vi "grading table searching.vi"() -> ()   [LabVIEW 2019, in "database.lvlib"]
uses:
  database.lvlib
panel:
  in  "OK":bool
  out "Query String":string
  out "String 4":string="Parameter"
  out "String 3":string="Operation"
  out "String 2":string="Value 2"
  out "String 1":string="Value 1"
  out "Value String 12":string="Value"
  out "Value String 11":string="Value"
  out "Value String 10":string="Value"
  out "Value String 9":string="Value"
  out "Value String 8":string="Value"
  out "Value String 7":string="Value"
  out "Value String 6":string="Value"
  out "Value String 5":string="Value"
  out "Value String 4":string="Value"
  out "Value String 3":string="Value"
  out "Value String 2":string="Value"
  out "Value String 1":string="Value"
  in  "Operator 17":u16(ring) items=["AND", "OR"]
  in  "Operator 16":u16(ring) items=["AND", "OR"]
  in  "Operator 15":u16(ring) items=["AND", "OR"]
  in  "Operator 14":u16(ring) items=["AND", "OR"]
  in  "Operator 13":u16(ring) items=["AND", "OR"]
  in  "sub 5":bool=TRUE
  in  "sub 4":bool=TRUE
  in  "sub 3":bool=TRUE
  in  "sub 2":bool=TRUE
  in  "sub 1":bool=TRUE
  in  "add 5":bool=TRUE
  in  "add 4":bool=TRUE
  in  "add 3":bool=TRUE
  in  "add 2":bool=TRUE
  in  "Operator 11":u16(ring) items=["All", "P=V1", "P#V1", "P<V1", "P<=V1", "P>V1", "P>=V1", "V1<P<V2", "V1<=P<V2", "V1<P<=V2", "V1<=P<=V2"]
  in  "Operator 9":u16(ring) items=["All", "P=V1", "P#V1", "P<V1", "P<=V1", "P>V1", "P>=V1", "V1<P<V2", "V1<=P<V2", "V1<P<=V2", "V1<=P<=V2"]
  in  "Operator 7":u16(ring) items=["All", "P=V1", "P#V1", "P<V1", "P<=V1", "P>V1", "P>=V1", "V1<P<V2", "V1<=P<V2", "V1<P<=V2", "V1<=P<=V2"]
  in  "Projector Situation 12":u16(ring) items=["OFF", "ON"]
  in  "Projector Situation 11":u16(ring) items=["OFF", "ON"]
  in  "Camera Situation 12":u16(ring) items=["OFF", "ON"]
  in  "Camera Situation 11":u16(ring) items=["OFF", "ON"]
  in  "Control Mode 12":u16(ring) items=["Manual", "Auto"]
  in  "Control Mode 11":u16(ring) items=["Manual", "Auto"]
  in  "Disc Situation 12":u16(ring) items=["Stop", "Run"]
  in  "Disc Situation 11":u16(ring) items=["Stop", "Run"]
  in  "Time 12":timestamp format="%<%H:%M:%S>T"
  in  "Time 11":timestamp format="%<%H:%M:%S>T"
  in  "Date 12":timestamp format="%<%Y/%m/%d>T"
  in  "Date 11":timestamp format="%<%Y/%m/%d>T"
  in  "Parameter 11":u16(ring) items=["Choose parameter", "Date", "Time", "Disc Situation", "Control Mode", "Camera Situation", "Projector Situation"]
  in  "Projector Situation 10":u16(ring) items=["OFF", "ON"]
  in  "Projector Situation 9":u16(ring) items=["OFF", "ON"]
  in  "Camera Situation 10":u16(ring) items=["OFF", "ON"]
  in  "Camera Situation 9":u16(ring) items=["OFF", "ON"]
  in  "Control Mode 10":u16(ring) items=["Manual", "Auto"]
  in  "Control Mode 9":u16(ring) items=["Manual", "Auto"]
  in  "Disc Situation 10":u16(ring) items=["Stop", "Run"]
  in  "Disc Situation 9":u16(ring) items=["Stop", "Run"]
  in  "Time 10":timestamp format="%<%H:%M:%S>T"
  in  "Time 9":timestamp format="%<%H:%M:%S>T"
  in  "Date 10":timestamp format="%<%Y/%m/%d>T"
  in  "Date 9":timestamp format="%<%Y/%m/%d>T"
  in  "Operator 5":u16(ring) items=["All", "P=V1", "P#V1", "P<V1", "P<=V1", "P>V1", "P>=V1", "V1<P<V2", "V1<=P<V2", "V1<P<=V2", "V1<=P<=V2"]
  in  "Parameter 9":u16(ring) items=["Choose parameter", "Date", "Time", "Disc Situation", "Control Mode", "Camera Situation", "Projector Situation"]
  in  "Projector Situation 8":u16(ring) items=["OFF", "ON"]
  in  "Projector Situation 7":u16(ring) items=["OFF", "ON"]
  in  "Camera Situation 8":u16(ring) items=["OFF", "ON"]
  in  "Camera Situation 7":u16(ring) items=["OFF", "ON"]
  in  "Control Mode 8":u16(ring) items=["Manual", "Auto"]
  in  "Control Mode 7":u16(ring) items=["Manual", "Auto"]
  in  "Disc Situation 8":u16(ring) items=["Stop", "Run"]
  in  "Disc Situation 7":u16(ring) items=["Stop", "Run"]
  in  "Time 8":timestamp format="%<%H:%M:%S>T"
  in  "Time 7":timestamp format="%<%H:%M:%S>T"
  in  "Date 8":timestamp format="%<%Y/%m/%d>T"
  in  "Date 7":timestamp format="%<%Y/%m/%d>T"
  in  "Parameter 7":u16(ring) items=["Choose parameter", "Date", "Time", "Disc Situation", "Control Mode", "Camera Situation", "Projector Situation"]
  in  "Projector Situation 6":u16(ring) items=["OFF", "ON"]
  in  "Projector Situation 5":u16(ring) items=["OFF", "ON"]
  in  "Camera Situation 6":u16(ring) items=["OFF", "ON"]
  in  "Camera Situation 5":u16(ring) items=["OFF", "ON"]
  in  "Control Mode 6":u16(ring) items=["Manual", "Auto"]
  in  "Control Mode 5":u16(ring) items=["Manual", "Auto"]
  in  "Disc Situation 6":u16(ring) items=["Stop", "Run"]
  in  "Disc Situation 5":u16(ring) items=["Stop", "Run"]
  in  "Time 6":timestamp format="%<%H:%M:%S>T"
  in  "Time 5":timestamp format="%<%H:%M:%S>T"
  in  "Date 6":timestamp format="%<%Y/%m/%d>T"
  in  "Date 5":timestamp format="%<%Y/%m/%d>T"
  in  "Operator 3":u16(ring) items=["All", "P=V1", "P#V1", "P<V1", "P<=V1", "P>V1", "P>=V1", "V1<P<V2", "V1<=P<V2", "V1<P<=V2", "V1<=P<=V2"]
  in  "Parameter 5":u16(ring) items=["Choose parameter", "Date", "Time", "Disc Situation", "Control Mode", "Camera Situation", "Projector Situation"]
  in  "Projector Situation 4":u16(ring) items=["OFF", "ON"]
  in  "Projector Situation 3":u16(ring) items=["OFF", "ON"]
  in  "Camera Situation 4":u16(ring) items=["OFF", "ON"]
  in  "Camera Situation 3":u16(ring) items=["OFF", "ON"]
  in  "Control Mode 4":u16(ring) items=["Manual", "Auto"]
  in  "Control Mode 3":u16(ring) items=["Manual", "Auto"]
  in  "Disc Situation 4":u16(ring) items=["Stop", "Run"]
  in  "Disc Situation 3":u16(ring) items=["Stop", "Run"]
  in  "Time 4":timestamp format="%<%H:%M:%S>T"
  in  "Time 3":timestamp format="%<%H:%M:%S>T"
  in  "Date 4":timestamp format="%<%Y/%m/%d>T"
  in  "Date 3":timestamp format="%<%Y/%m/%d>T"
  in  "Parameter 3":u16(ring) items=["Choose parameter", "Date", "Time", "Disc Situation", "Control Mode", "Camera Situation", "Projector Situation"]
  in  "Projector Situation 2":u16(ring) items=["OFF", "ON"]
  in  "Projector Situation 1":u16(ring) items=["OFF", "ON"]
  in  "Camera Situation 2":u16(ring) items=["OFF", "ON"]
  in  "Camera Situation 1":u16(ring) items=["OFF", "ON"]
  in  "Control Mode 2":u16(ring) items=["Manual", "Auto"]
  in  "Control Mode 1":u16(ring) items=["Manual", "Auto"]
  in  "Disc Situation 2":u16(ring) items=["Stop", "Run"]
  in  "Disc Situation 1":u16(ring) items=["Stop", "Run"]
  in  "Time 2":timestamp format="%<%H:%M:%S>T"
  in  "Time 1":timestamp format="%<%H:%M:%S>T"
  in  "Date 2":timestamp format="%<%Y/%m/%d>T"
  in  "Date 1":timestamp format="%<%Y/%m/%d>T"
  in  "Operator 1":u16(ring) items=["All", "P=V1", "P#V1", "P<V1", "P<=V1", "P>V1", "P>=V1", "V1<P<V2", "V1<=P<V2", "V1<P<=V2", "V1<=P<=V2"]
  in  "add 1":bool=TRUE
  in  "Parameter 1":u16(ring) items=["Choose parameter", "Date", "Time", "Disc Situation", "Control Mode", "Camera Situation", "Projector Situation"]
  out "Name":string="Search in Database"
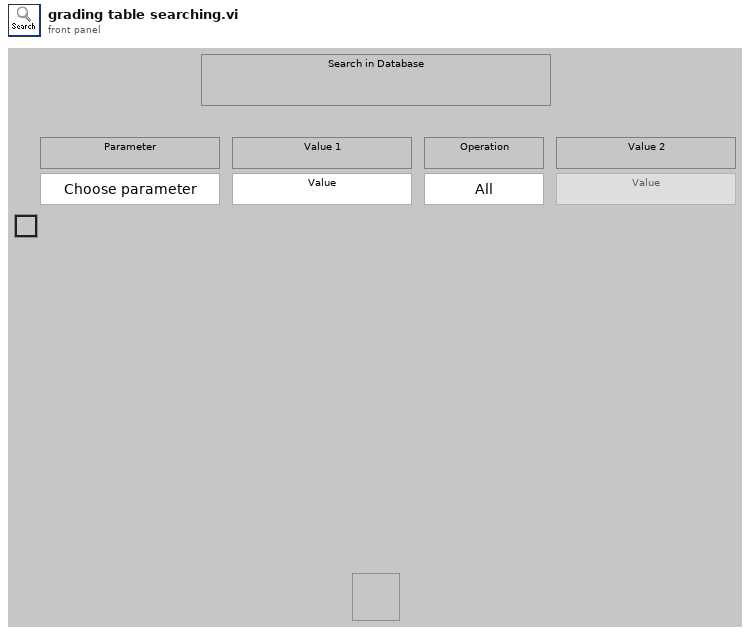
[diagram p1: front panel]
types:
  T1 = enum8{"Enabled", "Disabled", "Disabled and Grayed Out"}
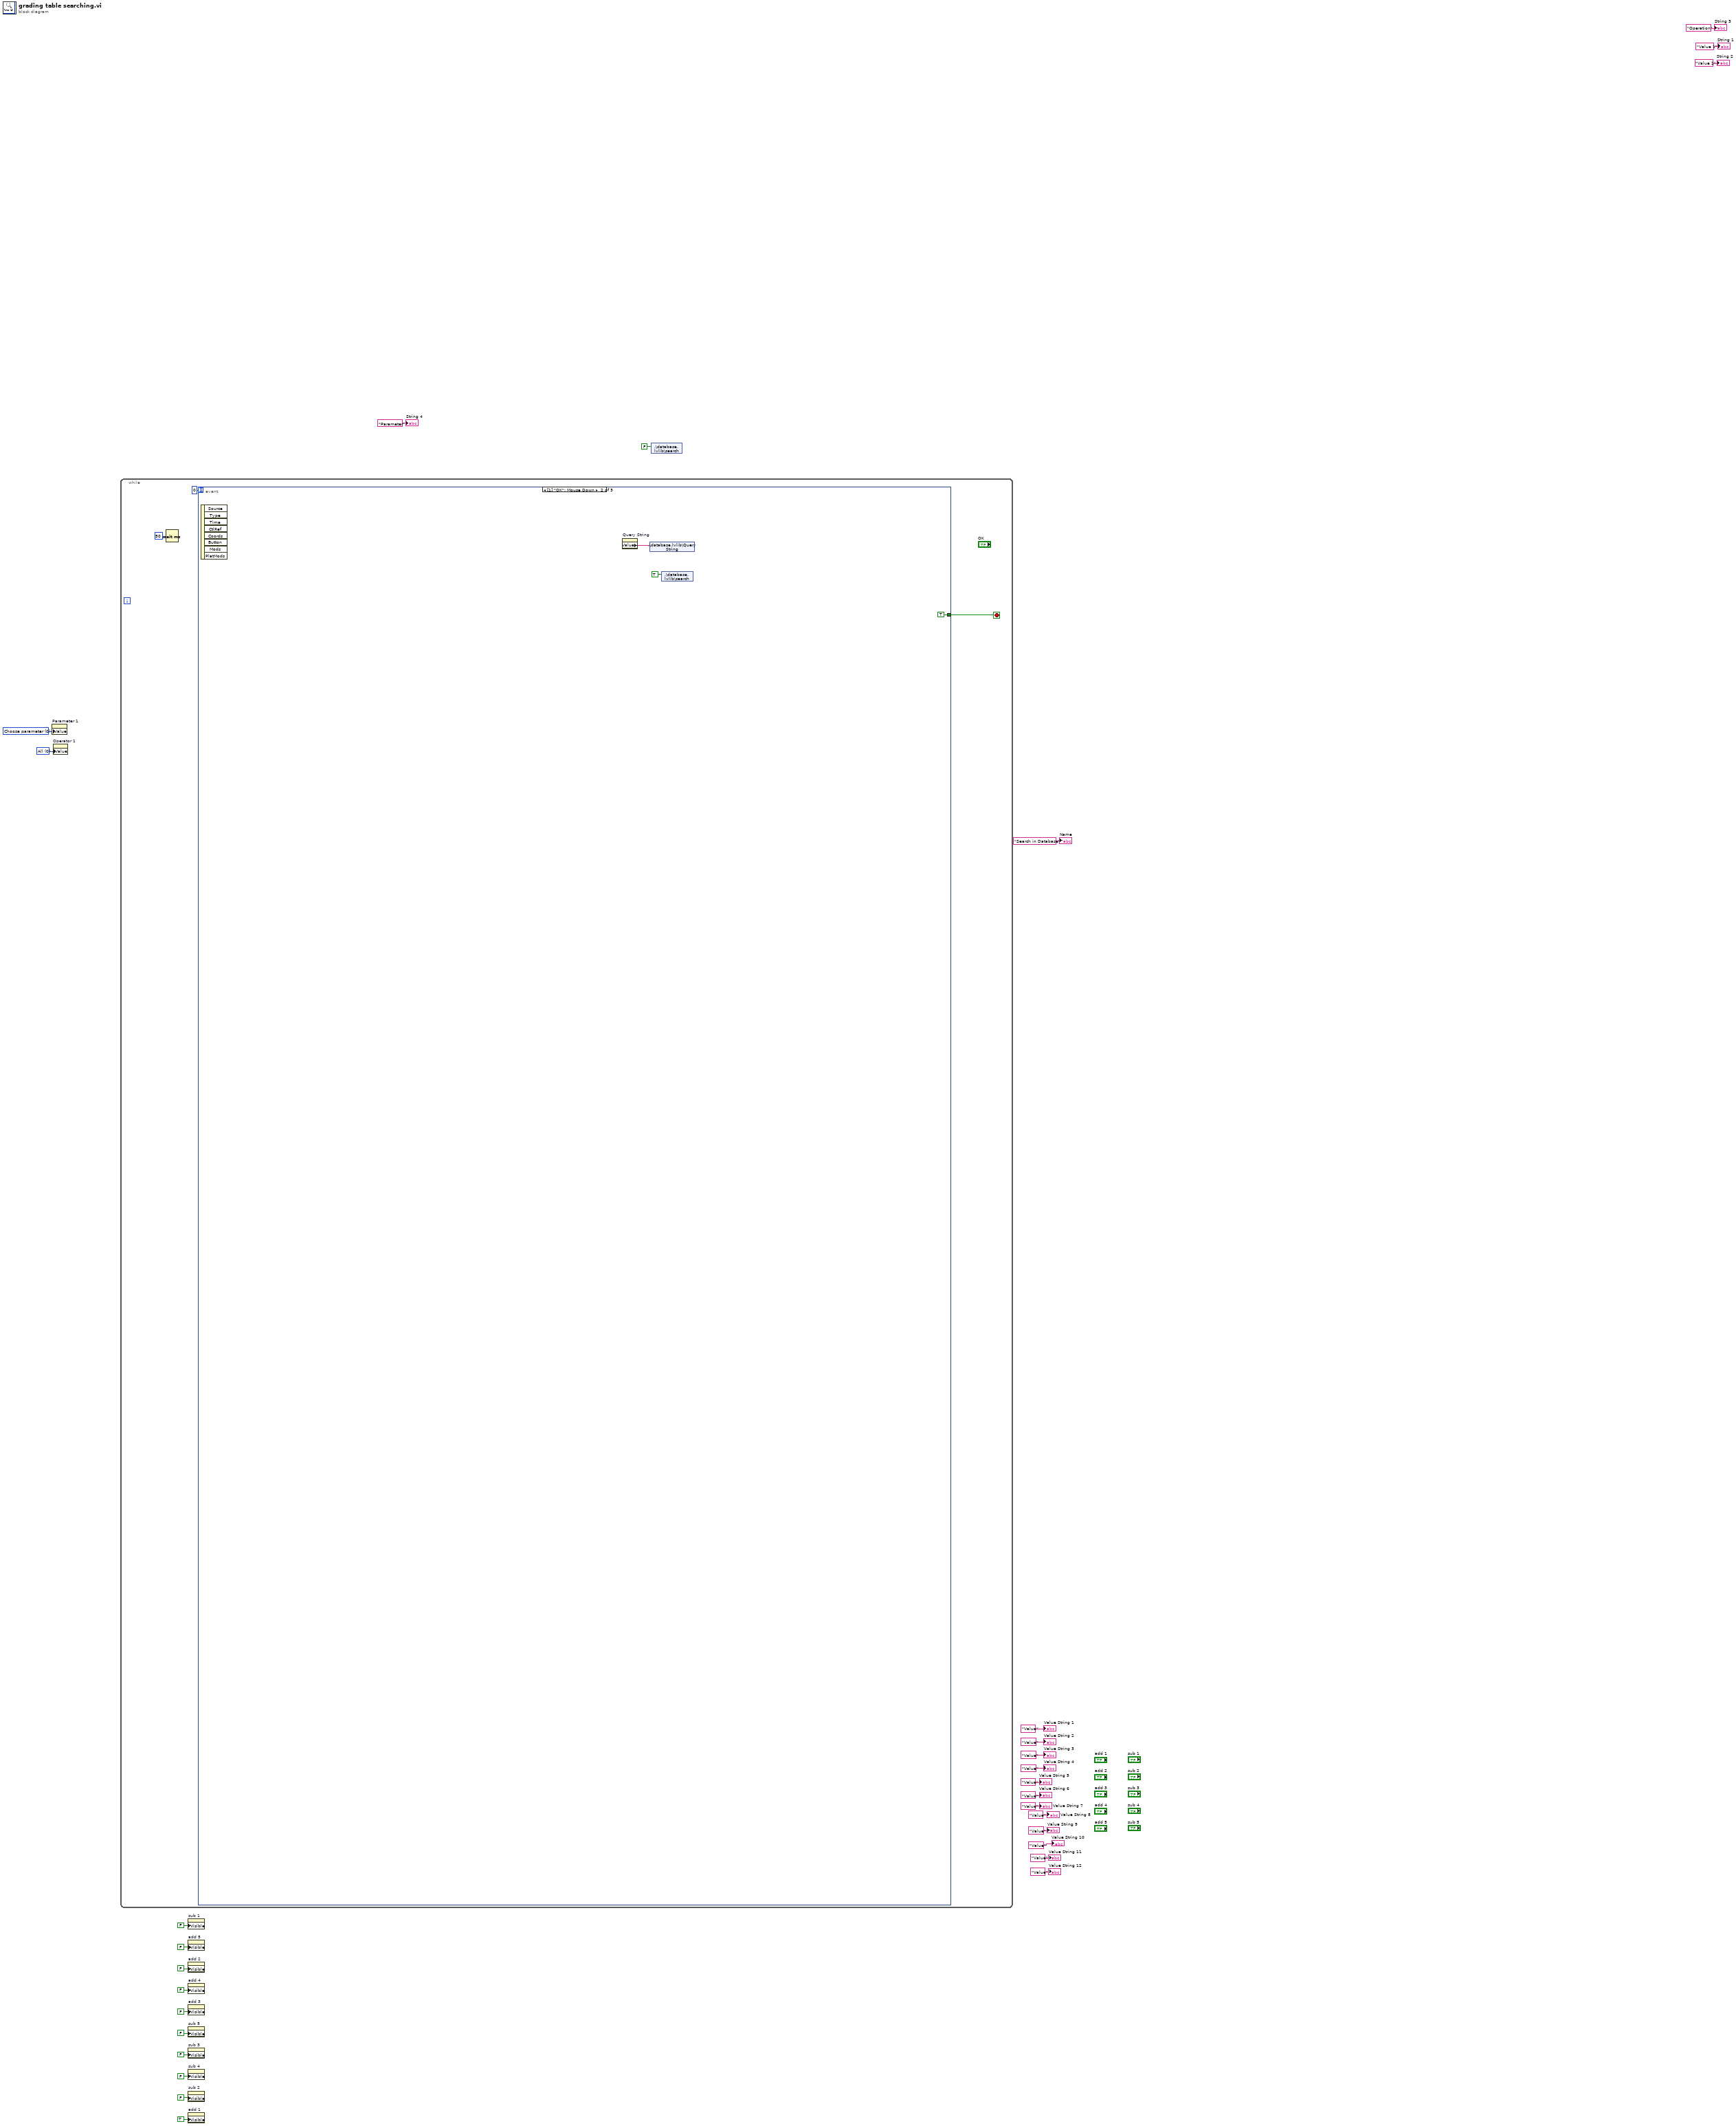
[diagram p0: block diagram]
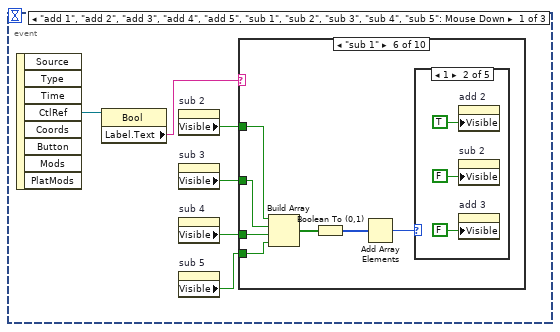
[diagram p2: hidden frame]
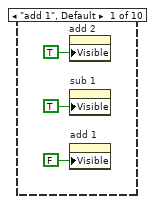
[diagram p3: hidden frame]
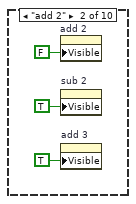
[diagram p4: hidden frame]
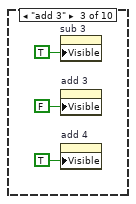
[diagram p5: hidden frame]
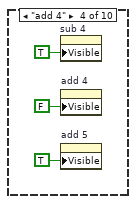
[diagram p6: hidden frame]
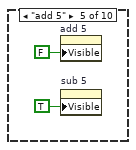
[diagram p7: hidden frame]
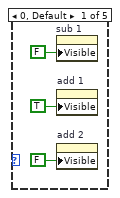
[diagram p8: hidden frame]
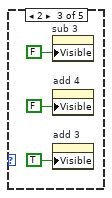
[diagram p9: hidden frame]
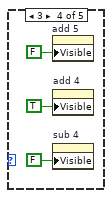
[diagram p10: hidden frame]
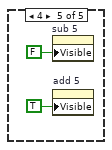
[diagram p11: hidden frame]
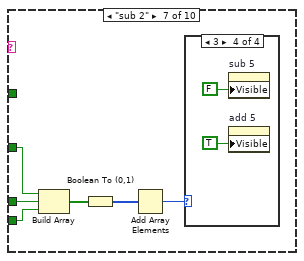
[diagram p12: hidden frame]
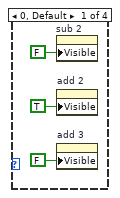
[diagram p13: hidden frame]
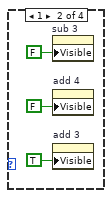
[diagram p14: hidden frame]
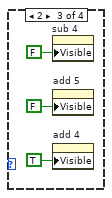
[diagram p15: hidden frame]
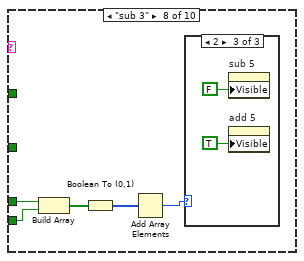
[diagram p16: hidden frame]
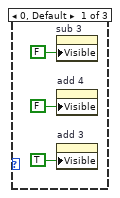
[diagram p17: hidden frame]
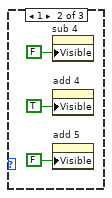
[diagram p18: hidden frame]
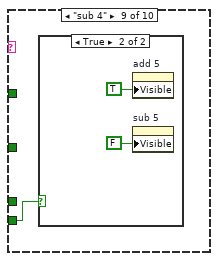
[diagram p19: hidden frame]
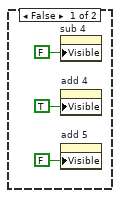
[diagram p20: hidden frame]
diagram:
  w3 = u16 0 items=["All", "P=V1", "P#V1", "P<V1", "P<=V1", "P>V1", "P>=V1", "V1<P<V2", "V1<=P<V2", "V1<P<=V2", "V1<=P<=V2"] ("Operator 1")
  w4 = u16 0 items=["Choose parameter", "Date", "Time", "Disc Situation", "Control Mode", "Camera Situation", "Projector Situation"] ("Parameter 1")
  n1 = property on="Parameter 1" class="Ring (strict)"("Value"=w4) -> ()  [unwired: 2 in, 2 out]
  n2 = property on="Operator 1" class="Ring (strict)"("Value"=w3) -> ()  [unwired: 2 in, 2 out]
  n3 = while {
    stop <- w31 stop-if-true
    n4 = Wait (ms)(milliseconds to wait=u32 50) -> ()  [unwired: 1 out]
    n5 = event shown="[1] \"OK\": Mouse Down" {
      selector: _ -> [_ _ _]
      dyn-events: _ -> [_ _ _]
      timeout: 0 -> [_ _ _]
      tunnel: [_ TRUE _] -> w31
      event "add 1", "add 2", "add 3", "add 4", "add 5", "sub 1", "sub 2", "sub 3", "sub 4", "sub 5": Mouse Down {
        n6 = event-data() -> ("CtlRef"=w39:refnum<vi>)  [unwired: 1 in, 7 out]
        n7 = property class="Bool"(reference=w39) -> ("Label.Text"=w38:string)  [unwired: 1 in, 2 out]
        n8 = property on="sub 2" class="Bool"() -> ("Visible"=w37:bool)  [unwired: 2 in, 2 out]
        n9 = property on="sub 3" class="Bool"() -> ("Visible"=w36:bool)  [unwired: 2 in, 2 out]
        n10 = property on="sub 4" class="Bool"() -> ("Visible"=w35:bool)  [unwired: 2 in, 2 out]
        n11 = property on="sub 5" class="Bool"() -> ("Visible"=w34:bool)  [unwired: 2 in, 2 out]
        n12 = case shown="\"sub 1\"" w38 {
          tunnel: w37 -> [_ _ _ _ _ w58 _ _ _ _]
          tunnel: w36 -> [_ _ _ _ _ w57 w78 _ _ _]
          tunnel: w35 -> [_ _ _ _ _ w56 w77 w94 _ _]
          tunnel: w34 -> [_ _ _ _ _ w55 w76 w93 w105 _]
          frame "add 1", Default {
            n13 = property on="add 2" class="Bool"("Visible"=TRUE) -> ()  [unwired: 2 in, 2 out]
            n14 = property on="sub 1" class="Bool"("Visible"=TRUE) -> ()  [unwired: 2 in, 2 out]
            n15 = property on="add 1" class="Bool"("Visible"=FALSE) -> ()  [unwired: 2 in, 2 out]
          }
          frame "add 2" {
            n16 = property on="add 2" class="Bool"("Visible"=FALSE) -> ()  [unwired: 2 in, 2 out]
            n17 = property on="sub 2" class="Bool"("Visible"=TRUE) -> ()  [unwired: 2 in, 2 out]
            n18 = property on="add 3" class="Bool"("Visible"=TRUE) -> ()  [unwired: 2 in, 2 out]
          }
          frame "add 3" {
            n19 = property on="sub 3" class="Bool"("Visible"=TRUE) -> ()  [unwired: 2 in, 2 out]
            n20 = property on="add 3" class="Bool"("Visible"=FALSE) -> ()  [unwired: 2 in, 2 out]
            n21 = property on="add 4" class="Bool"("Visible"=TRUE) -> ()  [unwired: 2 in, 2 out]
          }
          frame "add 4" {
            n22 = property on="sub 4" class="Bool"("Visible"=TRUE) -> ()  [unwired: 2 in, 2 out]
            n23 = property on="add 4" class="Bool"("Visible"=FALSE) -> ()  [unwired: 2 in, 2 out]
            n24 = property on="add 5" class="Bool"("Visible"=TRUE) -> ()  [unwired: 2 in, 2 out]
          }
          frame "add 5" {
            n25 = property on="add 5" class="Bool"("Visible"=FALSE) -> ()  [unwired: 2 in, 2 out]
            n26 = property on="sub 5" class="Bool"("Visible"=TRUE) -> ()  [unwired: 2 in, 2 out]
          }
          frame "sub 1" {
            n27 = Build Array(w58, w57, w56, w55) -> (w54:bool[])
            n28 = Boolean To (0,1)(Boolean=w54) -> (0, 1=w59:i16[])
            n29 = Add Array Elements(numeric array=w59) -> (sum=w60:i16)
            n30 = case shown="1" w60 {
              frame 0, Default {
                n31 = property on="sub 1" class="Bool"("Visible"=FALSE) -> ()  [unwired: 2 in, 2 out]
                n32 = property on="add 1" class="Bool"("Visible"=TRUE) -> ()  [unwired: 2 in, 2 out]
                n33 = property on="add 2" class="Bool"("Visible"=FALSE) -> ()  [unwired: 2 in, 2 out]
              }
              frame 1 {
                n34 = property on="add 2" class="Bool"("Visible"=TRUE) -> ()  [unwired: 2 in, 2 out]
                n35 = property on="sub 2" class="Bool"("Visible"=FALSE) -> ()  [unwired: 2 in, 2 out]
                n36 = property on="add 3" class="Bool"("Visible"=FALSE) -> ()  [unwired: 2 in, 2 out]
              }
              frame 2 {
                n37 = property on="sub 3" class="Bool"("Visible"=FALSE) -> ()  [unwired: 2 in, 2 out]
                n38 = property on="add 4" class="Bool"("Visible"=FALSE) -> ()  [unwired: 2 in, 2 out]
                n39 = property on="add 3" class="Bool"("Visible"=TRUE) -> ()  [unwired: 2 in, 2 out]
              }
              frame 3 {
                n40 = property on="add 5" class="Bool"("Visible"=FALSE) -> ()  [unwired: 2 in, 2 out]
                n41 = property on="add 4" class="Bool"("Visible"=TRUE) -> ()  [unwired: 2 in, 2 out]
                n42 = property on="sub 4" class="Bool"("Visible"=FALSE) -> ()  [unwired: 2 in, 2 out]
              }
              frame 4 {
                n43 = property on="sub 5" class="Bool"("Visible"=FALSE) -> ()  [unwired: 2 in, 2 out]
                n44 = property on="add 5" class="Bool"("Visible"=TRUE) -> ()  [unwired: 2 in, 2 out]
              }
            }
          }
          frame "sub 2" {
            n45 = Build Array(w78, w77, w76) -> (w79:bool[])
            n46 = Boolean To (0,1)(Boolean=w79) -> (0, 1=w80:i16[])
            n47 = Add Array Elements(numeric array=w80) -> (sum=w75:i16)
            n48 = case shown="3" w75 {
              frame 0, Default {
                n49 = property on="sub 2" class="Bool"("Visible"=FALSE) -> ()  [unwired: 2 in, 2 out]
                n50 = property on="add 2" class="Bool"("Visible"=TRUE) -> ()  [unwired: 2 in, 2 out]
                n51 = property on="add 3" class="Bool"("Visible"=FALSE) -> ()  [unwired: 2 in, 2 out]
              }
              frame 1 {
                n52 = property on="sub 3" class="Bool"("Visible"=FALSE) -> ()  [unwired: 2 in, 2 out]
                n53 = property on="add 4" class="Bool"("Visible"=FALSE) -> ()  [unwired: 2 in, 2 out]
                n54 = property on="add 3" class="Bool"("Visible"=TRUE) -> ()  [unwired: 2 in, 2 out]
              }
              frame 2 {
                n55 = property on="sub 4" class="Bool"("Visible"=FALSE) -> ()  [unwired: 2 in, 2 out]
                n56 = property on="add 5" class="Bool"("Visible"=FALSE) -> ()  [unwired: 2 in, 2 out]
                n57 = property on="add 4" class="Bool"("Visible"=TRUE) -> ()  [unwired: 2 in, 2 out]
              }
              frame 3 {
                n58 = property on="sub 5" class="Bool"("Visible"=FALSE) -> ()  [unwired: 2 in, 2 out]
                n59 = property on="add 5" class="Bool"("Visible"=TRUE) -> ()  [unwired: 2 in, 2 out]
              }
            }
          }
          frame "sub 3" {
            n60 = Build Array(w94, w93) -> (w95:bool[])
            n61 = Boolean To (0,1)(Boolean=w95) -> (0, 1=w96:i16[])
            n62 = Add Array Elements(numeric array=w96) -> (sum=w92:i16)
            n63 = case shown="2" w92 {
              frame 0, Default {
                n64 = property on="sub 3" class="Bool"("Visible"=FALSE) -> ()  [unwired: 2 in, 2 out]
                n65 = property on="add 4" class="Bool"("Visible"=FALSE) -> ()  [unwired: 2 in, 2 out]
                n66 = property on="add 3" class="Bool"("Visible"=TRUE) -> ()  [unwired: 2 in, 2 out]
              }
              frame 1 {
                n67 = property on="sub 4" class="Bool"("Visible"=FALSE) -> ()  [unwired: 2 in, 2 out]
                n68 = property on="add 4" class="Bool"("Visible"=TRUE) -> ()  [unwired: 2 in, 2 out]
                n69 = property on="add 5" class="Bool"("Visible"=FALSE) -> ()  [unwired: 2 in, 2 out]
              }
              frame 2 {
                n70 = property on="sub 5" class="Bool"("Visible"=FALSE) -> ()  [unwired: 2 in, 2 out]
                n71 = property on="add 5" class="Bool"("Visible"=TRUE) -> ()  [unwired: 2 in, 2 out]
              }
            }
          }
          frame "sub 4" {
            n72 = case shown="True" w105 {
              frame False {
                n73 = property on="sub 4" class="Bool"("Visible"=FALSE) -> ()  [unwired: 2 in, 2 out]
                n74 = property on="add 4" class="Bool"("Visible"=TRUE) -> ()  [unwired: 2 in, 2 out]
                n75 = property on="add 5" class="Bool"("Visible"=FALSE) -> ()  [unwired: 2 in, 2 out]
              }
              frame True {
                n76 = property on="add 5" class="Bool"("Visible"=TRUE) -> ()  [unwired: 2 in, 2 out]
                n77 = property on="sub 5" class="Bool"("Visible"=FALSE) -> ()  [unwired: 2 in, 2 out]
              }
            }
          }
          frame "sub 5" {
            n78 = property on="sub 5" class="Bool"("Visible"=FALSE) -> ()  [unwired: 2 in, 2 out]
            n79 = property on="add 5" class="Bool"("Visible"=TRUE) -> ()  [unwired: 2 in, 2 out]
          }
        }
      }
      event "OK": Mouse Down {
        n80 = event-data() -> ()  [unwired: 1 in, 8 out]
        n81 = property on="Query String" class="Str"() -> ("Value"=w115:string)  [unwired: 2 in, 2 out]
        n82 = shared-variable ".\\database.lvlib\\Query String"(w115) -> ()  [unwired: 1 in, 1 out]
        n83 = shared-variable ".\\database.lvlib\\search"(TRUE ("search")) -> ()  [unwired: 1 in, 1 out]
      }
      event Timeout {
        n84 = event-data() -> ()  [unwired: 1 in, 3 out]
        n85 = property on="sub 5" class="Bool"() -> ("Visible"=w158:bool)  [unwired: 2 in, 2 out]
        n86 = property on="sub 2" class="Bool"() -> ("Visible"=w173:bool)  [unwired: 2 in, 2 out]
        n87 = property on="sub 4" class="Bool"() -> ("Visible"=w159:bool)  [unwired: 2 in, 2 out]
        n88 = property on="sub 3" class="Bool"() -> ("Visible"=w164:bool)  [unwired: 2 in, 2 out]
        n89 = property on="sub 1" class="Bool"() -> ("Visible"=w174:bool)  [unwired: 2 in, 2 out]
        n90 = property on="sub 1" class="Bool"() -> ("Visible"=w188:bool)  [unwired: 2 in, 2 out]
        n91 = property on="sub 2" class="Bool"() -> ("Visible"=w189:bool)  [unwired: 2 in, 2 out]
        n92 = property on="sub 3" class="Bool"() -> ("Visible"=w190:bool)  [unwired: 2 in, 2 out]
        n93 = property on="sub 4" class="Bool"() -> ("Visible"=w191:bool)  [unwired: 2 in, 2 out]
        n94 = property on="sub 5" class="Bool"() -> ("Visible"=w192:bool)  [unwired: 2 in, 2 out]
        n95 = case shown="True" w158 {
          tunnel: "Parameter 11" -> [_ w375]
          tunnel: ["" ("format string") w374] -> w156
          tunnel: ["" w373] -> w155
          tunnel: ["" ("date/time string") w372] -> w154
          frame False {
            w356 = u16 0 items=["Choose parameter", "Date", "Time", "Disc Situation", "Control Mode", "Camera Situation", "Projector Situation"] ("Parameter 11")
            w357 = u16 0 items=["All", "P=V1", "P#V1", "P<V1", "P<=V1", "P>V1", "P>=V1", "V1<P<V2", "V1<=P<V2", "V1<P<=V2", "V1<=P<=V2"] ("Operator 11")
            n96 = property on="Date 12" class="AbsTime (strict)"("Visible"=FALSE) -> ()  [unwired: 2 in, 2 out]
            n97 = property on="Date 11" class="AbsTime (strict)"("Visible"=FALSE) -> ()  [unwired: 2 in, 2 out]
            n98 = property on="Time 11" class="AbsTime (strict)"("Visible"=FALSE) -> ()  [unwired: 2 in, 2 out]
            n99 = property on="Time 12" class="AbsTime (strict)"("Visible"=FALSE) -> ()  [unwired: 2 in, 2 out]
            n100 = property on="Disc Situation 12" class="Ring (strict)"("Visible"=FALSE) -> ()  [unwired: 2 in, 2 out]
            n101 = property on="Disc Situation 11" class="Ring (strict)"("Visible"=FALSE) -> ()  [unwired: 2 in, 2 out]
            n102 = property on="Camera Situation 11" class="Ring (strict)"("Visible"=FALSE) -> ()  [unwired: 2 in, 2 out]
            n103 = property on="Camera Situation 12" class="Ring (strict)"("Visible"=FALSE) -> ()  [unwired: 2 in, 2 out]
            n104 = property on="Value String 11" class="Str"("Visible"=FALSE) -> ()  [unwired: 2 in, 2 out]
            n105 = property on="Value String 12" class="Str"("Visible"=FALSE) -> ()  [unwired: 2 in, 2 out]
            n106 = property on="Control Mode 11" class="Ring (strict)"("Visible"=FALSE) -> ()  [unwired: 2 in, 2 out]
            n107 = property on="Control Mode 12" class="Ring (strict)"("Visible"=FALSE) -> ()  [unwired: 2 in, 2 out]
            n108 = property on="Operator 11" class="Ring (strict)"("Value"=w357) -> ()  [unwired: 2 in, 2 out]
            n109 = property on="Parameter 11" class="Ring (strict)"("Value"=w356) -> ()  [unwired: 2 in, 2 out]
            n110 = property on="Projector Situation 11" class="Ring (strict)"("Visible"=FALSE) -> ()  [unwired: 2 in, 2 out]
            n111 = property on="Projector Situation 12" class="Ring (strict)"("Visible"=FALSE) -> ()  [unwired: 2 in, 2 out]
          }
          frame True {
            n112 = case shown="0, Default" w375 {
              tunnel: ["" "date" ("format string") "time" ("format string") "disc_situation" ("format string") "control_mode" ("format string") "camera_situation" ("format string") "projector_situation" ("format string")] -> w374
              tunnel: ["" w398 w427 w454 w474 w495 w517] -> w373
              tunnel: ["" ("date/time string") w397 w425 "" ("date/time string") "" ("date/time string") "" ("date/time string") "" ("date/time string")] -> w372
              frame 0, Default {
                w376 = u16 0 items=["All", "P=V1", "P#V1", "P<V1", "P<=V1", "P>V1", "P>=V1", "V1<P<V2", "V1<=P<V2", "V1<P<=V2", "V1<=P<=V2"] ("Operator 11")
                n113 = property on="Date 12" class="AbsTime (strict)"("Visible"=FALSE) -> ()  [unwired: 2 in, 2 out]
                n114 = property on="Date 11" class="AbsTime (strict)"("Visible"=FALSE) -> ()  [unwired: 2 in, 2 out]
                n115 = property on="Time 11" class="AbsTime (strict)"("Visible"=FALSE) -> ()  [unwired: 2 in, 2 out]
                n116 = property on="Time 12" class="AbsTime (strict)"("Visible"=FALSE) -> ()  [unwired: 2 in, 2 out]
                n117 = property on="Disc Situation 12" class="Ring (strict)"("Visible"=FALSE) -> ()  [unwired: 2 in, 2 out]
                n118 = property on="Disc Situation 11" class="Ring (strict)"("Visible"=FALSE) -> ()  [unwired: 2 in, 2 out]
                n119 = property on="Camera Situation 11" class="Ring (strict)"("Visible"=FALSE) -> ()  [unwired: 2 in, 2 out]
                n120 = property on="Camera Situation 12" class="Ring (strict)"("Visible"=FALSE) -> ()  [unwired: 2 in, 2 out]
                n121 = property on="Value String 11" class="Str"("Visible"=TRUE) -> ()  [unwired: 2 in, 2 out]
                n122 = property on="Value String 12" class="Str"("Visible"=TRUE) -> ()  [unwired: 2 in, 2 out]
                n123 = property on="Control Mode 11" class="Ring (strict)"("Visible"=FALSE) -> ()  [unwired: 2 in, 2 out]
                n124 = property on="Control Mode 12" class="Ring (strict)"("Visible"=FALSE) -> ()  [unwired: 2 in, 2 out]
                n125 = property on="Projector Situation 11" class="Ring (strict)"("Visible"=FALSE) -> ()  [unwired: 2 in, 2 out]
                n126 = property on="Projector Situation 12" class="Ring (strict)"("Visible"=FALSE) -> ()  [unwired: 2 in, 2 out]
                n127 = property on="Operator 11" class="Ring (strict)"("Disabled Items []"=i32[] [1, 2, 3, 4, 5, 6, 7, 8, 9, 10], "Value"=w376) -> ()  [unwired: 2 in, 2 out]
              }
              frame 1 {
                n128 = property on="Date 12" class="AbsTime (strict)"("Visible"=TRUE) -> ()  [unwired: 2 in, 2 out]
                n129 = property on="Date 11" class="AbsTime (strict)"("Visible"=TRUE) -> ()  [unwired: 2 in, 2 out]
                n130 = property on="Time 11" class="AbsTime (strict)"("Visible"=FALSE) -> ()  [unwired: 2 in, 2 out]
                n131 = property on="Time 12" class="AbsTime (strict)"("Visible"=FALSE) -> ()  [unwired: 2 in, 2 out]
                n132 = property on="Disc Situation 12" class="Ring (strict)"("Visible"=FALSE) -> ()  [unwired: 2 in, 2 out]
                n133 = property on="Disc Situation 11" class="Ring (strict)"("Visible"=FALSE) -> ()  [unwired: 2 in, 2 out]
                n134 = property on="Camera Situation 11" class="Ring (strict)"("Visible"=FALSE) -> ()  [unwired: 2 in, 2 out]
                n135 = property on="Camera Situation 12" class="Ring (strict)"("Visible"=FALSE) -> ()  [unwired: 2 in, 2 out]
                n136 = property on="Value String 11" class="Str"("Visible"=FALSE) -> ()  [unwired: 2 in, 2 out]
                n137 = property on="Value String 12" class="Str"("Visible"=FALSE) -> ()  [unwired: 2 in, 2 out]
                n138 = property on="Control Mode 11" class="Ring (strict)"("Visible"=FALSE) -> ()  [unwired: 2 in, 2 out]
                n139 = property on="Control Mode 12" class="Ring (strict)"("Visible"=FALSE) -> ()  [unwired: 2 in, 2 out]
                n140 = Format Date/Time String(time format string (%c)="%Y/%m/%d", seconds (now)="Date 12") -> (date/time string=w407:string)  [unwired: 1 in]
                n141 = Format Date/Time String(time format string (%c)="%Y/%m/%d", seconds (now)="Date 11") -> (date/time string=w406:string)  [unwired: 1 in]
                n142 = property on="Projector Situation 11" class="Ring (strict)"("Visible"=FALSE) -> ()  [unwired: 2 in, 2 out]
                n143 = property on="Projector Situation 12" class="Ring (strict)"("Visible"=FALSE) -> ()  [unwired: 2 in, 2 out]
                n144 = property on="Operator 11" class="Ring (strict)"("Disabled Items []"=i32[] []) -> ()  [unwired: 2 in, 2 out]
                n145 = Concatenate Strings("'" ("string"), w406, "'" ("string")) -> (w398:string)
                n146 = Concatenate Strings("'" ("string"), w407, "'" ("string")) -> (w397:string)
              }
              frame 2 {
                n147 = property on="Date 12" class="AbsTime (strict)"("Visible"=FALSE) -> ()  [unwired: 2 in, 2 out]
                n148 = property on="Date 11" class="AbsTime (strict)"("Visible"=FALSE) -> ()  [unwired: 2 in, 2 out]
                n149 = property on="Time 11" class="AbsTime (strict)"("Visible"=TRUE) -> ()  [unwired: 2 in, 2 out]
                n150 = property on="Time 12" class="AbsTime (strict)"("Visible"=TRUE) -> ()  [unwired: 2 in, 2 out]
                n151 = property on="Disc Situation 12" class="Ring (strict)"("Visible"=FALSE) -> ()  [unwired: 2 in, 2 out]
                n152 = property on="Disc Situation 11" class="Ring (strict)"("Visible"=FALSE) -> ()  [unwired: 2 in, 2 out]
                n153 = property on="Camera Situation 11" class="Ring (strict)"("Visible"=FALSE) -> ()  [unwired: 2 in, 2 out]
                n154 = property on="Camera Situation 12" class="Ring (strict)"("Visible"=FALSE) -> ()  [unwired: 2 in, 2 out]
                n155 = property on="Value String 11" class="Str"("Visible"=FALSE) -> ()  [unwired: 2 in, 2 out]
                n156 = property on="Value String 12" class="Str"("Visible"=FALSE) -> ()  [unwired: 2 in, 2 out]
                n157 = property on="Control Mode 11" class="Ring (strict)"("Visible"=FALSE) -> ()  [unwired: 2 in, 2 out]
                n158 = property on="Control Mode 12" class="Ring (strict)"("Visible"=FALSE) -> ()  [unwired: 2 in, 2 out]
                n159 = Format Date/Time String(time format string (%c)="%H:%M:%S", seconds (now)="Time 11") -> (date/time string=w435:string)  [unwired: 1 in]
                n160 = Format Date/Time String(time format string (%c)="%H:%M:%S", seconds (now)="Time 12") -> (date/time string=w434:string)  [unwired: 1 in]
                n161 = property on="Projector Situation 11" class="Ring (strict)"("Visible"=FALSE) -> ()  [unwired: 2 in, 2 out]
                n162 = property on="Projector Situation 12" class="Ring (strict)"("Visible"=FALSE) -> ()  [unwired: 2 in, 2 out]
                n163 = Concatenate Strings("'" ("string"), w435, "'" ("string")) -> (w427:string)
                n164 = Concatenate Strings("'" ("string"), w434, "'" ("string")) -> (w425:string)
                n165 = property on="Operator 11" class="Ring (strict)"("Disabled Items []"=i32[] []) -> ()  [unwired: 2 in, 2 out]
              }
              frame 3 {
                n166 = property on="Date 12" class="AbsTime (strict)"("Visible"=FALSE) -> ()  [unwired: 2 in, 2 out]
                n167 = property on="Date 11" class="AbsTime (strict)"("Visible"=FALSE) -> ()  [unwired: 2 in, 2 out]
                n168 = property on="Time 11" class="AbsTime (strict)"("Visible"=FALSE) -> ()  [unwired: 2 in, 2 out]
                n169 = property on="Time 12" class="AbsTime (strict)"("Visible"=FALSE) -> ()  [unwired: 2 in, 2 out]
                n170 = property on="Disc Situation 12" class="Ring (strict)"("Visible"=TRUE) -> ()  [unwired: 2 in, 2 out]
                n171 = property on="Disc Situation 11" class="Ring (strict)"("Visible"=TRUE) -> ()  [unwired: 2 in, 2 out]
                n172 = property on="Camera Situation 11" class="Ring (strict)"("Visible"=FALSE) -> ()  [unwired: 2 in, 2 out]
                n173 = property on="Camera Situation 12" class="Ring (strict)"("Visible"=FALSE) -> ()  [unwired: 2 in, 2 out]
                n174 = property on="Value String 11" class="Str"("Visible"=FALSE) -> ()  [unwired: 2 in, 2 out]
                n175 = property on="Value String 12" class="Str"("Visible"=FALSE) -> ()  [unwired: 2 in, 2 out]
                n176 = property on="Control Mode 11" class="Ring (strict)"("Visible"=FALSE) -> ()  [unwired: 2 in, 2 out]
                n177 = property on="Control Mode 12" class="Ring (strict)"("Visible"=FALSE) -> ()  [unwired: 2 in, 2 out]
                n178 = case shown="0, Default" "Disc Situation 11" {
                  tunnel: ["'Stop'" "'Run'"] -> w454
                  frame 0, Default {
                  }
                  frame 1 {
                  }
                }
                n179 = property on="Projector Situation 11" class="Ring (strict)"("Visible"=FALSE) -> ()  [unwired: 2 in, 2 out]
                n180 = property on="Projector Situation 12" class="Ring (strict)"("Visible"=FALSE) -> ()  [unwired: 2 in, 2 out]
                n181 = property on="Operator 11" class="Ring (strict)"("Disabled Items []"=i32[] [2, 3, 4, 5, 6, 7, 8, 9, 10]) -> ()  [unwired: 2 in, 2 out]
              }
              frame 4 {
                n182 = property on="Date 12" class="AbsTime (strict)"("Visible"=FALSE) -> ()  [unwired: 2 in, 2 out]
                n183 = property on="Date 11" class="AbsTime (strict)"("Visible"=FALSE) -> ()  [unwired: 2 in, 2 out]
                n184 = property on="Time 11" class="AbsTime (strict)"("Visible"=FALSE) -> ()  [unwired: 2 in, 2 out]
                n185 = property on="Time 12" class="AbsTime (strict)"("Visible"=FALSE) -> ()  [unwired: 2 in, 2 out]
                n186 = property on="Disc Situation 12" class="Ring (strict)"("Visible"=FALSE) -> ()  [unwired: 2 in, 2 out]
                n187 = property on="Disc Situation 11" class="Ring (strict)"("Visible"=FALSE) -> ()  [unwired: 2 in, 2 out]
                n188 = property on="Camera Situation 11" class="Ring (strict)"("Visible"=FALSE) -> ()  [unwired: 2 in, 2 out]
                n189 = property on="Camera Situation 12" class="Ring (strict)"("Visible"=FALSE) -> ()  [unwired: 2 in, 2 out]
                n190 = property on="Value String 11" class="Str"("Visible"=FALSE) -> ()  [unwired: 2 in, 2 out]
                n191 = property on="Value String 12" class="Str"("Visible"=FALSE) -> ()  [unwired: 2 in, 2 out]
                n192 = property on="Control Mode 11" class="Ring (strict)"("Visible"=TRUE) -> ()  [unwired: 2 in, 2 out]
                n193 = property on="Control Mode 12" class="Ring (strict)"("Visible"=TRUE) -> ()  [unwired: 2 in, 2 out]
                n194 = case shown="1" "Control Mode 11" {
                  tunnel: ["'Manual'" "'Auto'"] -> w474
                  frame 0, Default {
                  }
                  frame 1 {
                  }
                }
                n195 = property on="Projector Situation 11" class="Ring (strict)"("Visible"=FALSE) -> ()  [unwired: 2 in, 2 out]
                n196 = property on="Projector Situation 12" class="Ring (strict)"("Visible"=FALSE) -> ()  [unwired: 2 in, 2 out]
                n197 = property on="Operator 11" class="Ring (strict)"("Disabled Items []"=i32[] [2, 3, 4, 5, 6, 7, 8, 9, 10]) -> ()  [unwired: 2 in, 2 out]
              }
              frame 5 {
                n198 = property on="Date 12" class="AbsTime (strict)"("Visible"=FALSE) -> ()  [unwired: 2 in, 2 out]
                n199 = property on="Date 11" class="AbsTime (strict)"("Visible"=FALSE) -> ()  [unwired: 2 in, 2 out]
                n200 = property on="Time 11" class="AbsTime (strict)"("Visible"=FALSE) -> ()  [unwired: 2 in, 2 out]
                n201 = property on="Time 12" class="AbsTime (strict)"("Visible"=FALSE) -> ()  [unwired: 2 in, 2 out]
                n202 = property on="Disc Situation 12" class="Ring (strict)"("Visible"=FALSE) -> ()  [unwired: 2 in, 2 out]
                n203 = property on="Disc Situation 11" class="Ring (strict)"("Visible"=FALSE) -> ()  [unwired: 2 in, 2 out]
                n204 = property on="Camera Situation 11" class="Ring (strict)"("Visible"=TRUE) -> ()  [unwired: 2 in, 2 out]
                n205 = property on="Camera Situation 12" class="Ring (strict)"("Visible"=TRUE) -> ()  [unwired: 2 in, 2 out]
                n206 = property on="Value String 11" class="Str"("Visible"=FALSE) -> ()  [unwired: 2 in, 2 out]
                n207 = property on="Value String 12" class="Str"("Visible"=FALSE) -> ()  [unwired: 2 in, 2 out]
                n208 = property on="Control Mode 11" class="Ring (strict)"("Visible"=FALSE) -> ()  [unwired: 2 in, 2 out]
                n209 = property on="Control Mode 12" class="Ring (strict)"("Visible"=FALSE) -> ()  [unwired: 2 in, 2 out]
                n210 = case shown="1" "Camera Situation 11" {
                  tunnel: ["'OFF'" "'ON'"] -> w495
                  frame 0, Default {
                  }
                  frame 1 {
                  }
                }
                n211 = property on="Projector Situation 11" class="Ring (strict)"("Visible"=FALSE) -> ()  [unwired: 2 in, 2 out]
                n212 = property on="Projector Situation 12" class="Ring (strict)"("Visible"=FALSE) -> ()  [unwired: 2 in, 2 out]
                n213 = property on="Operator 11" class="Ring (strict)"("Disabled Items []"=i32[] [2, 3, 4, 5, 6, 7, 8, 9, 10]) -> ()  [unwired: 2 in, 2 out]
              }
              frame 6 {
                n214 = property on="Date 12" class="AbsTime (strict)"("Visible"=FALSE) -> ()  [unwired: 2 in, 2 out]
                n215 = property on="Date 11" class="AbsTime (strict)"("Visible"=FALSE) -> ()  [unwired: 2 in, 2 out]
                n216 = property on="Time 11" class="AbsTime (strict)"("Visible"=FALSE) -> ()  [unwired: 2 in, 2 out]
                n217 = property on="Time 12" class="AbsTime (strict)"("Visible"=FALSE) -> ()  [unwired: 2 in, 2 out]
                n218 = property on="Disc Situation 12" class="Ring (strict)"("Visible"=FALSE) -> ()  [unwired: 2 in, 2 out]
                n219 = property on="Disc Situation 11" class="Ring (strict)"("Visible"=FALSE) -> ()  [unwired: 2 in, 2 out]
                n220 = property on="Camera Situation 11" class="Ring (strict)"("Visible"=FALSE) -> ()  [unwired: 2 in, 2 out]
                n221 = property on="Camera Situation 12" class="Ring (strict)"("Visible"=FALSE) -> ()  [unwired: 2 in, 2 out]
                n222 = property on="Value String 11" class="Str"("Visible"=FALSE) -> ()  [unwired: 2 in, 2 out]
                n223 = property on="Value String 12" class="Str"("Visible"=FALSE) -> ()  [unwired: 2 in, 2 out]
                n224 = property on="Control Mode 11" class="Ring (strict)"("Visible"=FALSE) -> ()  [unwired: 2 in, 2 out]
                n225 = property on="Control Mode 12" class="Ring (strict)"("Visible"=FALSE) -> ()  [unwired: 2 in, 2 out]
                n226 = property on="Projector Situation 11" class="Ring (strict)"("Visible"=TRUE) -> ()  [unwired: 2 in, 2 out]
                n227 = property on="Projector Situation 12" class="Ring (strict)"("Visible"=TRUE) -> ()  [unwired: 2 in, 2 out]
                n228 = case shown="0, Default" "Projector Situation 11" {
                  tunnel: ["'OFF'" "'ON'"] -> w517
                  frame 0, Default {
                  }
                  frame 1 {
                  }
                }
                n229 = property on="Operator 11" class="Ring (strict)"("Disabled Items []"=i32[] [2, 3, 4, 5, 6, 7, 8, 9, 10]) -> ()  [unwired: 2 in, 2 out]
              }
            }
          }
        }
        n230 = case shown="True" w164 {
          tunnel: "Parameter 7" -> [_ w814]
          tunnel: ["" ("format string") w813] -> w162
          tunnel: ["" w812] -> w161
          tunnel: ["" ("date/time string") w811] -> w160
          frame False {
            w795 = u16 0 items=["All", "P=V1", "P#V1", "P<V1", "P<=V1", "P>V1", "P>=V1", "V1<P<V2", "V1<=P<V2", "V1<P<=V2", "V1<=P<=V2"] ("Operator 7")
            w796 = u16 0 items=["Choose parameter", "Date", "Time", "Disc Situation", "Control Mode", "Camera Situation", "Projector Situation"] ("Parameter 7")
            n231 = property on="Camera Situation 8" class="Ring (strict)"("Visible"=FALSE) -> ()  [unwired: 2 in, 2 out]
            n232 = property on="Camera Situation 7" class="Ring (strict)"("Visible"=FALSE) -> ()  [unwired: 2 in, 2 out]
            n233 = property on="Date 7" class="AbsTime (strict)"("Visible"=FALSE) -> ()  [unwired: 2 in, 2 out]
            n234 = property on="Date 8" class="AbsTime (strict)"("Visible"=FALSE) -> ()  [unwired: 2 in, 2 out]
            n235 = property on="Time 7" class="AbsTime (strict)"("Visible"=FALSE) -> ()  [unwired: 2 in, 2 out]
            n236 = property on="Time 8" class="AbsTime (strict)"("Visible"=FALSE) -> ()  [unwired: 2 in, 2 out]
            n237 = property on="Value String 7" class="Str"("Visible"=FALSE) -> ()  [unwired: 2 in, 2 out]
            n238 = property on="Value String 8" class="Str"("Visible"=FALSE) -> ()  [unwired: 2 in, 2 out]
            n239 = property on="Disc Situation 7" class="Ring (strict)"("Visible"=FALSE) -> ()  [unwired: 2 in, 2 out]
            n240 = property on="Disc Situation 8" class="Ring (strict)"("Visible"=FALSE) -> ()  [unwired: 2 in, 2 out]
            n241 = property on="Operator 7" class="Ring (strict)"("Value"=w795) -> ()  [unwired: 2 in, 2 out]
            n242 = property on="Parameter 7" class="Ring (strict)"("Value"=w796) -> ()  [unwired: 2 in, 2 out]
            n243 = property on="Projector Situation 7" class="Ring (strict)"("Visible"=FALSE) -> ()  [unwired: 2 in, 2 out]
            n244 = property on="Projector Situation 8" class="Ring (strict)"("Visible"=FALSE) -> ()  [unwired: 2 in, 2 out]
            n245 = property on="Control Mode 7" class="Ring (strict)"("Visible"=FALSE) -> ()  [unwired: 2 in, 2 out]
            n246 = property on="Control Mode 8" class="Ring (strict)"("Visible"=FALSE) -> ()  [unwired: 2 in, 2 out]
          }
          frame True {
            n247 = case shown="0, Default" w814 {
              tunnel: ["" ("format string") "date" ("format string") "time" ("format string") "disc_situation" ("format string") "control_mode" ("format string") "camera_situation" ("format string") "projector_situation" ("format string")] -> w813
              tunnel: ["" w837 w863 w893 w914 w933 w956] -> w812
              tunnel: ["" ("date/time string") w836 w862 "" ("date/time string") "" ("date/time string") "" ("date/time string") "" ("date/time string")] -> w811
              frame 0, Default {
                w815 = u16 0 items=["All", "P=V1", "P#V1", "P<V1", "P<=V1", "P>V1", "P>=V1", "V1<P<V2", "V1<=P<V2", "V1<P<=V2", "V1<=P<=V2"] ("Operator 7")
                n248 = property on="Camera Situation 8" class="Ring (strict)"("Visible"=FALSE) -> ()  [unwired: 2 in, 2 out]
                n249 = property on="Camera Situation 7" class="Ring (strict)"("Visible"=FALSE) -> ()  [unwired: 2 in, 2 out]
                n250 = property on="Date 7" class="AbsTime (strict)"("Visible"=FALSE) -> ()  [unwired: 2 in, 2 out]
                n251 = property on="Date 8" class="AbsTime (strict)"("Visible"=FALSE) -> ()  [unwired: 2 in, 2 out]
                n252 = property on="Disc Situation 7" class="Ring (strict)"("Visible"=FALSE) -> ()  [unwired: 2 in, 2 out]
                n253 = property on="Disc Situation 8" class="Ring (strict)"("Visible"=FALSE) -> ()  [unwired: 2 in, 2 out]
                n254 = property on="Value String 7" class="Str"("Visible"=TRUE) -> ()  [unwired: 2 in, 2 out]
                n255 = property on="Value String 8" class="Str"("Visible"=TRUE) -> ()  [unwired: 2 in, 2 out]
                n256 = property on="Time 7" class="AbsTime (strict)"("Visible"=FALSE) -> ()  [unwired: 2 in, 2 out]
                n257 = property on="Time 8" class="AbsTime (strict)"("Visible"=FALSE) -> ()  [unwired: 2 in, 2 out]
                n258 = property on="Control Mode 7" class="Ring (strict)"("Visible"=FALSE) -> ()  [unwired: 2 in, 2 out]
                n259 = property on="Control Mode 8" class="Ring (strict)"("Visible"=FALSE) -> ()  [unwired: 2 in, 2 out]
                n260 = property on="Projector Situation 7" class="Ring (strict)"("Visible"=FALSE) -> ()  [unwired: 2 in, 2 out]
                n261 = property on="Projector Situation 8" class="Ring (strict)"("Visible"=FALSE) -> ()  [unwired: 2 in, 2 out]
                n262 = property on="Operator 7" class="Ring (strict)"("Disabled Items []"=i32[] [1, 2, 3, 4, 5, 6, 7, 8, 9, 10], "Value"=w815) -> ()  [unwired: 2 in, 2 out]
              }
              frame 1 {
                n263 = property on="Camera Situation 8" class="Ring (strict)"("Visible"=FALSE) -> ()  [unwired: 2 in, 2 out]
                n264 = property on="Camera Situation 7" class="Ring (strict)"("Visible"=FALSE) -> ()  [unwired: 2 in, 2 out]
                n265 = property on="Date 7" class="AbsTime (strict)"("Visible"=TRUE) -> ()  [unwired: 2 in, 2 out]
                n266 = property on="Date 8" class="AbsTime (strict)"("Visible"=TRUE) -> ()  [unwired: 2 in, 2 out]
                n267 = property on="Disc Situation 7" class="Ring (strict)"("Visible"=FALSE) -> ()  [unwired: 2 in, 2 out]
                n268 = property on="Disc Situation 8" class="Ring (strict)"("Visible"=FALSE) -> ()  [unwired: 2 in, 2 out]
                n269 = property on="Value String 7" class="Str"("Visible"=FALSE) -> ()  [unwired: 2 in, 2 out]
                n270 = property on="Value String 8" class="Str"("Visible"=FALSE) -> ()  [unwired: 2 in, 2 out]
                n271 = property on="Time 7" class="AbsTime (strict)"("Visible"=FALSE) -> ()  [unwired: 2 in, 2 out]
                n272 = property on="Time 8" class="AbsTime (strict)"("Visible"=FALSE) -> ()  [unwired: 2 in, 2 out]
                n273 = property on="Control Mode 7" class="Ring (strict)"("Visible"=FALSE) -> ()  [unwired: 2 in, 2 out]
                n274 = property on="Control Mode 8" class="Ring (strict)"("Visible"=FALSE) -> ()  [unwired: 2 in, 2 out]
                n275 = Format Date/Time String(time format string (%c)="%Y/%m/%d", seconds (now)="Date 8") -> (date/time string=w846:string)  [unwired: 1 in]
                n276 = Format Date/Time String(time format string (%c)="%Y/%m/%d", seconds (now)="Date 7") -> (date/time string=w845:string)  [unwired: 1 in]
                n277 = property on="Projector Situation 7" class="Ring (strict)"("Visible"=FALSE) -> ()  [unwired: 2 in, 2 out]
                n278 = property on="Projector Situation 8" class="Ring (strict)"("Visible"=FALSE) -> ()  [unwired: 2 in, 2 out]
                n279 = property on="Operator 7" class="Ring (strict)"("Disabled Items []"=i32[] []) -> ()  [unwired: 2 in, 2 out]
                n280 = Concatenate Strings("'" ("string"), w845, "'" ("string")) -> (w837:string)
                n281 = Concatenate Strings("'" ("string"), w846, "'" ("string")) -> (w836:string)
              }
              frame 2 {
                n282 = property on="Camera Situation 8" class="Ring (strict)"("Visible"=FALSE) -> ()  [unwired: 2 in, 2 out]
                n283 = property on="Camera Situation 7" class="Ring (strict)"("Visible"=FALSE) -> ()  [unwired: 2 in, 2 out]
                n284 = property on="Date 7" class="AbsTime (strict)"("Visible"=FALSE) -> ()  [unwired: 2 in, 2 out]
                n285 = property on="Date 8" class="AbsTime (strict)"("Visible"=FALSE) -> ()  [unwired: 2 in, 2 out]
                n286 = property on="Disc Situation 7" class="Ring (strict)"("Visible"=FALSE) -> ()  [unwired: 2 in, 2 out]
                n287 = property on="Disc Situation 8" class="Ring (strict)"("Visible"=FALSE) -> ()  [unwired: 2 in, 2 out]
                n288 = property on="Value String 7" class="Str"("Visible"=FALSE) -> ()  [unwired: 2 in, 2 out]
                n289 = property on="Value String 8" class="Str"("Visible"=FALSE) -> ()  [unwired: 2 in, 2 out]
                n290 = property on="Time 7" class="AbsTime (strict)"("Visible"=TRUE) -> ()  [unwired: 2 in, 2 out]
                n291 = property on="Time 8" class="AbsTime (strict)"("Visible"=TRUE) -> ()  [unwired: 2 in, 2 out]
                n292 = property on="Control Mode 7" class="Ring (strict)"("Visible"=FALSE) -> ()  [unwired: 2 in, 2 out]
                n293 = property on="Control Mode 8" class="Ring (strict)"("Visible"=FALSE) -> ()  [unwired: 2 in, 2 out]
                n294 = Format Date/Time String(time format string (%c)="%H:%M:%S", seconds (now)="Time 8") -> (date/time string=w874:string)  [unwired: 1 in]
                n295 = Format Date/Time String(time format string (%c)="%H:%M:%S", seconds (now)="Time 7") -> (date/time string=w873:string)  [unwired: 1 in]
                n296 = property on="Projector Situation 7" class="Ring (strict)"("Visible"=FALSE) -> ()  [unwired: 2 in, 2 out]
                n297 = property on="Projector Situation 8" class="Ring (strict)"("Visible"=FALSE) -> ()  [unwired: 2 in, 2 out]
                n298 = property on="Operator 7" class="Ring (strict)"("Disabled Items []"=i32[] []) -> ()  [unwired: 2 in, 2 out]
                n299 = Concatenate Strings("'" ("string"), w874, "'" ("string")) -> (w863:string)
                n300 = Concatenate Strings("'" ("string"), w873, "'" ("string")) -> (w862:string)
              }
              frame 3 {
                n301 = property on="Camera Situation 8" class="Ring (strict)"("Visible"=FALSE) -> ()  [unwired: 2 in, 2 out]
                n302 = property on="Camera Situation 7" class="Ring (strict)"("Visible"=FALSE) -> ()  [unwired: 2 in, 2 out]
                n303 = property on="Date 7" class="AbsTime (strict)"("Visible"=FALSE) -> ()  [unwired: 2 in, 2 out]
                n304 = property on="Date 8" class="AbsTime (strict)"("Visible"=FALSE) -> ()  [unwired: 2 in, 2 out]
                n305 = property on="Disc Situation 7" class="Ring (strict)"("Visible"=TRUE) -> ()  [unwired: 2 in, 2 out]
                n306 = property on="Disc Situation 8" class="Ring (strict)"("Visible"=TRUE) -> ()  [unwired: 2 in, 2 out]
                n307 = property on="Value String 7" class="Str"("Visible"=FALSE) -> ()  [unwired: 2 in, 2 out]
                n308 = property on="Value String 8" class="Str"("Visible"=FALSE) -> ()  [unwired: 2 in, 2 out]
                n309 = property on="Time 7" class="AbsTime (strict)"("Visible"=FALSE) -> ()  [unwired: 2 in, 2 out]
                n310 = property on="Time 8" class="AbsTime (strict)"("Visible"=FALSE) -> ()  [unwired: 2 in, 2 out]
                n311 = property on="Control Mode 7" class="Ring (strict)"("Visible"=FALSE) -> ()  [unwired: 2 in, 2 out]
                n312 = property on="Control Mode 8" class="Ring (strict)"("Visible"=FALSE) -> ()  [unwired: 2 in, 2 out]
                n313 = case shown="0, Default" "Disc Situation 7" {
                  tunnel: ["'Stop'" "'Run'"] -> w893
                  frame 0, Default {
                  }
                  frame 1 {
                  }
                }
                n314 = property on="Projector Situation 7" class="Ring (strict)"("Visible"=FALSE) -> ()  [unwired: 2 in, 2 out]
                n315 = property on="Projector Situation 8" class="Ring (strict)"("Visible"=FALSE) -> ()  [unwired: 2 in, 2 out]
                n316 = property on="Operator 7" class="Ring (strict)"("Disabled Items []"=i32[] [2, 3, 4, 5, 6, 7, 8, 9, 10]) -> ()  [unwired: 2 in, 2 out]
              }
              frame 4 {
                n317 = property on="Camera Situation 8" class="Ring (strict)"("Visible"=FALSE) -> ()  [unwired: 2 in, 2 out]
                n318 = property on="Camera Situation 7" class="Ring (strict)"("Visible"=FALSE) -> ()  [unwired: 2 in, 2 out]
                n319 = property on="Date 7" class="AbsTime (strict)"("Visible"=FALSE) -> ()  [unwired: 2 in, 2 out]
                n320 = property on="Date 8" class="AbsTime (strict)"("Visible"=FALSE) -> ()  [unwired: 2 in, 2 out]
                n321 = property on="Disc Situation 7" class="Ring (strict)"("Visible"=FALSE) -> ()  [unwired: 2 in, 2 out]
                n322 = property on="Disc Situation 8" class="Ring (strict)"("Visible"=FALSE) -> ()  [unwired: 2 in, 2 out]
                n323 = property on="Value String 7" class="Str"("Visible"=FALSE) -> ()  [unwired: 2 in, 2 out]
                n324 = property on="Value String 8" class="Str"("Visible"=FALSE) -> ()  [unwired: 2 in, 2 out]
                n325 = property on="Time 7" class="AbsTime (strict)"("Visible"=FALSE) -> ()  [unwired: 2 in, 2 out]
                n326 = property on="Time 8" class="AbsTime (strict)"("Visible"=FALSE) -> ()  [unwired: 2 in, 2 out]
                n327 = property on="Control Mode 7" class="Ring (strict)"("Visible"=TRUE) -> ()  [unwired: 2 in, 2 out]
                n328 = property on="Control Mode 8" class="Ring (strict)"("Visible"=TRUE) -> ()  [unwired: 2 in, 2 out]
                n329 = case shown="1" "Control Mode 7" {
                  tunnel: ["'Manual'" "'Auto'"] -> w914
                  frame 0, Default {
                  }
                  frame 1 {
                  }
                }
                n330 = property on="Projector Situation 7" class="Ring (strict)"("Visible"=FALSE) -> ()  [unwired: 2 in, 2 out]
                n331 = property on="Projector Situation 8" class="Ring (strict)"("Visible"=FALSE) -> ()  [unwired: 2 in, 2 out]
                n332 = property on="Operator 7" class="Ring (strict)"("Disabled Items []"=i32[] [2, 3, 4, 5, 6, 7, 8, 9, 10]) -> ()  [unwired: 2 in, 2 out]
              }
              frame 5 {
                n333 = property on="Camera Situation 8" class="Ring (strict)"("Visible"=TRUE) -> ()  [unwired: 2 in, 2 out]
                n334 = property on="Camera Situation 7" class="Ring (strict)"("Visible"=TRUE) -> ()  [unwired: 2 in, 2 out]
                n335 = property on="Date 7" class="AbsTime (strict)"("Visible"=FALSE) -> ()  [unwired: 2 in, 2 out]
                n336 = property on="Date 8" class="AbsTime (strict)"("Visible"=FALSE) -> ()  [unwired: 2 in, 2 out]
                n337 = property on="Disc Situation 7" class="Ring (strict)"("Visible"=FALSE) -> ()  [unwired: 2 in, 2 out]
                n338 = property on="Disc Situation 8" class="Ring (strict)"("Visible"=FALSE) -> ()  [unwired: 2 in, 2 out]
                n339 = property on="Value String 7" class="Str"("Visible"=FALSE) -> ()  [unwired: 2 in, 2 out]
                n340 = property on="Value String 8" class="Str"("Visible"=FALSE) -> ()  [unwired: 2 in, 2 out]
                n341 = property on="Time 7" class="AbsTime (strict)"("Visible"=FALSE) -> ()  [unwired: 2 in, 2 out]
                n342 = property on="Time 8" class="AbsTime (strict)"("Visible"=FALSE) -> ()  [unwired: 2 in, 2 out]
                n343 = property on="Control Mode 7" class="Ring (strict)"("Visible"=FALSE) -> ()  [unwired: 2 in, 2 out]
                n344 = property on="Control Mode 8" class="Ring (strict)"("Visible"=FALSE) -> ()  [unwired: 2 in, 2 out]
                n345 = case shown="1" "Camera Situation 7" {
                  tunnel: ["'OFF'" "'ON'"] -> w933
                  frame 0, Default {
                  }
                  frame 1 {
                  }
                }
                n346 = property on="Projector Situation 7" class="Ring (strict)"("Visible"=FALSE) -> ()  [unwired: 2 in, 2 out]
                n347 = property on="Projector Situation 8" class="Ring (strict)"("Visible"=FALSE) -> ()  [unwired: 2 in, 2 out]
                n348 = property on="Operator 7" class="Ring (strict)"("Disabled Items []"=i32[] [2, 3, 4, 5, 6, 7, 8, 9, 10]) -> ()  [unwired: 2 in, 2 out]
              }
              frame 6 {
                n349 = property on="Camera Situation 8" class="Ring (strict)"("Visible"=FALSE) -> ()  [unwired: 2 in, 2 out]
                n350 = property on="Camera Situation 7" class="Ring (strict)"("Visible"=FALSE) -> ()  [unwired: 2 in, 2 out]
                n351 = property on="Date 7" class="AbsTime (strict)"("Visible"=FALSE) -> ()  [unwired: 2 in, 2 out]
                n352 = property on="Date 8" class="AbsTime (strict)"("Visible"=FALSE) -> ()  [unwired: 2 in, 2 out]
                n353 = property on="Disc Situation 7" class="Ring (strict)"("Visible"=FALSE) -> ()  [unwired: 2 in, 2 out]
                n354 = property on="Disc Situation 8" class="Ring (strict)"("Visible"=FALSE) -> ()  [unwired: 2 in, 2 out]
                n355 = property on="Value String 7" class="Str"("Visible"=FALSE) -> ()  [unwired: 2 in, 2 out]
                n356 = property on="Value String 8" class="Str"("Visible"=FALSE) -> ()  [unwired: 2 in, 2 out]
                n357 = property on="Time 7" class="AbsTime (strict)"("Visible"=FALSE) -> ()  [unwired: 2 in, 2 out]
                n358 = property on="Time 8" class="AbsTime (strict)"("Visible"=FALSE) -> ()  [unwired: 2 in, 2 out]
                n359 = property on="Control Mode 7" class="Ring (strict)"("Visible"=FALSE) -> ()  [unwired: 2 in, 2 out]
                n360 = property on="Control Mode 8" class="Ring (strict)"("Visible"=FALSE) -> ()  [unwired: 2 in, 2 out]
                n361 = case shown="0, Default" "Projector Situation 7" {
                  tunnel: ["'OFF'" "'ON'"] -> w956
                  frame 0, Default {
                  }
                  frame 1 {
                  }
                }
                n362 = property on="Projector Situation 7" class="Ring (strict)"("Visible"=TRUE) -> ()  [unwired: 2 in, 2 out]
                n363 = property on="Projector Situation 8" class="Ring (strict)"("Visible"=TRUE) -> ()  [unwired: 2 in, 2 out]
                n364 = property on="Operator 7" class="Ring (strict)"("Disabled Items []"=i32[] [2, 3, 4, 5, 6, 7, 8, 9, 10]) -> ()  [unwired: 2 in, 2 out]
              }
            }
          }
        }
        n365 = case shown="True" w159 {
          tunnel: "Parameter 9" -> [_ w557]
          tunnel: ["" ("format string") w556] -> w152
          tunnel: ["" w555] -> w151
          tunnel: ["" ("date/time string") w554] -> w150
          frame False {
            w538 = u16 0 items=["All", "P=V1", "P#V1", "P<V1", "P<=V1", "P>V1", "P>=V1", "V1<P<V2", "V1<=P<V2", "V1<P<=V2", "V1<=P<=V2"] ("Operator 9")
            w539 = u16 0 items=["Choose parameter", "Date", "Time", "Disc Situation", "Control Mode", "Camera Situation", "Projector Situation"] ("Parameter 9")
            n366 = property on="Date 10" class="AbsTime (strict)"("Visible"=FALSE) -> ()  [unwired: 2 in, 2 out]
            n367 = property on="Time 10" class="AbsTime (strict)"("Visible"=FALSE) -> ()  [unwired: 2 in, 2 out]
            n368 = property on="Date 9" class="AbsTime (strict)"("Visible"=FALSE) -> ()  [unwired: 2 in, 2 out]
            n369 = property on="Time 9" class="AbsTime (strict)"("Visible"=FALSE) -> ()  [unwired: 2 in, 2 out]
            n370 = property on="Disc Situation 9" class="Ring (strict)"("Visible"=FALSE) -> ()  [unwired: 2 in, 2 out]
            n371 = property on="Disc Situation 10" class="Ring (strict)"("Visible"=FALSE) -> ()  [unwired: 2 in, 2 out]
            n372 = property on="Camera Situation 10" class="Ring (strict)"("Visible"=FALSE) -> ()  [unwired: 2 in, 2 out]
            n373 = property on="Camera Situation 9" class="Ring (strict)"("Visible"=FALSE) -> ()  [unwired: 2 in, 2 out]
            n374 = property on="Control Mode 10" class="Ring (strict)"("Visible"=FALSE) -> ()  [unwired: 2 in, 2 out]
            n375 = property on="Control Mode 9" class="Ring (strict)"("Visible"=FALSE) -> ()  [unwired: 2 in, 2 out]
            n376 = property on="Value String 10" class="Str"("Visible"=FALSE) -> ()  [unwired: 2 in, 2 out]
            n377 = property on="Value String 9" class="Str"("Visible"=FALSE) -> ()  [unwired: 2 in, 2 out]
            n378 = property on="Projector Situation 9" class="Ring (strict)"("Visible"=FALSE) -> ()  [unwired: 2 in, 2 out]
            n379 = property on="Projector Situation 10" class="Ring (strict)"("Visible"=FALSE) -> ()  [unwired: 2 in, 2 out]
            n380 = property on="Parameter 9" class="Ring (strict)"("Value"=w539) -> ()  [unwired: 2 in, 2 out]
            n381 = property on="Operator 9" class="Ring (strict)"("Value"=w538) -> ()  [unwired: 2 in, 2 out]
          }
          frame True {
            n382 = case shown="5" w557 {
              tunnel: ["" ("format string") "date" ("format string") "time" ("format string") "disc_situation" ("format string") "control_mode" ("format string") "camera_situation" ("format string") "projector_situation" ("format string")] -> w556
              tunnel: ["" w581 w608 w636 w657 w677 w698] -> w555
              tunnel: ["" ("date/time string") w580 w607 "" ("date/time string") "" ("date/time string") "" ("date/time string") "" ("date/time string")] -> w554
              frame 0, Default {
                w558 = u16 0 items=["All", "P=V1", "P#V1", "P<V1", "P<=V1", "P>V1", "P>=V1", "V1<P<V2", "V1<=P<V2", "V1<P<=V2", "V1<=P<=V2"] ("Operator 9")
                n383 = property on="Date 10" class="AbsTime (strict)"("Visible"=FALSE) -> ()  [unwired: 2 in, 2 out]
                n384 = property on="Time 10" class="AbsTime (strict)"("Visible"=FALSE) -> ()  [unwired: 2 in, 2 out]
                n385 = property on="Date 9" class="AbsTime (strict)"("Visible"=FALSE) -> ()  [unwired: 2 in, 2 out]
                n386 = property on="Time 9" class="AbsTime (strict)"("Visible"=FALSE) -> ()  [unwired: 2 in, 2 out]
                n387 = property on="Disc Situation 9" class="Ring (strict)"("Visible"=FALSE) -> ()  [unwired: 2 in, 2 out]
                n388 = property on="Disc Situation 10" class="Ring (strict)"("Visible"=FALSE) -> ()  [unwired: 2 in, 2 out]
                n389 = property on="Camera Situation 10" class="Ring (strict)"("Visible"=FALSE) -> ()  [unwired: 2 in, 2 out]
                n390 = property on="Camera Situation 9" class="Ring (strict)"("Visible"=FALSE) -> ()  [unwired: 2 in, 2 out]
                n391 = property on="Control Mode 10" class="Ring (strict)"("Visible"=FALSE) -> ()  [unwired: 2 in, 2 out]
                n392 = property on="Control Mode 9" class="Ring (strict)"("Visible"=FALSE) -> ()  [unwired: 2 in, 2 out]
                n393 = property on="Value String 10" class="Str"("Visible"=TRUE) -> ()  [unwired: 2 in, 2 out]
                n394 = property on="Value String 9" class="Str"("Visible"=TRUE) -> ()  [unwired: 2 in, 2 out]
                n395 = property on="Projector Situation 9" class="Ring (strict)"("Visible"=FALSE) -> ()  [unwired: 2 in, 2 out]
                n396 = property on="Projector Situation 10" class="Ring (strict)"("Visible"=FALSE) -> ()  [unwired: 2 in, 2 out]
                n397 = property on="Operator 9" class="Ring (strict)"("Disabled Items []"=i32[] [1, 2, 3, 4, 5, 6, 7, 8, 9, 10], "Value"=w558) -> ()  [unwired: 2 in, 2 out]
              }
              frame 1 {
                n398 = property on="Date 10" class="AbsTime (strict)"("Visible"=TRUE) -> ()  [unwired: 2 in, 2 out]
                n399 = property on="Time 10" class="AbsTime (strict)"("Visible"=FALSE) -> ()  [unwired: 2 in, 2 out]
                n400 = property on="Date 9" class="AbsTime (strict)"("Visible"=TRUE) -> ()  [unwired: 2 in, 2 out]
                n401 = property on="Time 9" class="AbsTime (strict)"("Visible"=FALSE) -> ()  [unwired: 2 in, 2 out]
                n402 = property on="Disc Situation 9" class="Ring (strict)"("Visible"=FALSE) -> ()  [unwired: 2 in, 2 out]
                n403 = property on="Disc Situation 10" class="Ring (strict)"("Visible"=FALSE) -> ()  [unwired: 2 in, 2 out]
                n404 = property on="Camera Situation 10" class="Ring (strict)"("Visible"=FALSE) -> ()  [unwired: 2 in, 2 out]
                n405 = property on="Camera Situation 9" class="Ring (strict)"("Visible"=FALSE) -> ()  [unwired: 2 in, 2 out]
                n406 = property on="Control Mode 10" class="Ring (strict)"("Visible"=FALSE) -> ()  [unwired: 2 in, 2 out]
                n407 = property on="Control Mode 9" class="Ring (strict)"("Visible"=FALSE) -> ()  [unwired: 2 in, 2 out]
                n408 = property on="Value String 10" class="Str"("Visible"=FALSE) -> ()  [unwired: 2 in, 2 out]
                n409 = property on="Value String 9" class="Str"("Visible"=FALSE) -> ()  [unwired: 2 in, 2 out]
                n410 = property on="Projector Situation 9" class="Ring (strict)"("Visible"=FALSE) -> ()  [unwired: 2 in, 2 out]
                n411 = property on="Projector Situation 10" class="Ring (strict)"("Visible"=FALSE) -> ()  [unwired: 2 in, 2 out]
                n412 = Format Date/Time String(time format string (%c)="%Y/%m/%d", seconds (now)="Date 9") -> (date/time string=w589:string)  [unwired: 1 in]
                n413 = Format Date/Time String(time format string (%c)="%Y/%m/%d", seconds (now)="Date 10") -> (date/time string=w588:string)  [unwired: 1 in]
                n414 = property on="Operator 9" class="Ring (strict)"("Disabled Items []"=i32[] []) -> ()  [unwired: 2 in, 2 out]
                n415 = Concatenate Strings("'" ("string"), w589, "'" ("string")) -> (w581:string)
                n416 = Concatenate Strings("'" ("string"), w588, "'" ("string")) -> (w580:string)
              }
              frame 2 {
                n417 = property on="Date 10" class="AbsTime (strict)"("Visible"=FALSE) -> ()  [unwired: 2 in, 2 out]
                n418 = property on="Time 10" class="AbsTime (strict)"("Visible"=TRUE) -> ()  [unwired: 2 in, 2 out]
                n419 = property on="Date 9" class="AbsTime (strict)"("Visible"=FALSE) -> ()  [unwired: 2 in, 2 out]
                n420 = property on="Time 9" class="AbsTime (strict)"("Visible"=TRUE) -> ()  [unwired: 2 in, 2 out]
                n421 = property on="Disc Situation 9" class="Ring (strict)"("Visible"=FALSE) -> ()  [unwired: 2 in, 2 out]
                n422 = property on="Disc Situation 10" class="Ring (strict)"("Visible"=FALSE) -> ()  [unwired: 2 in, 2 out]
                n423 = property on="Camera Situation 10" class="Ring (strict)"("Visible"=FALSE) -> ()  [unwired: 2 in, 2 out]
                n424 = property on="Camera Situation 9" class="Ring (strict)"("Visible"=FALSE) -> ()  [unwired: 2 in, 2 out]
                n425 = property on="Control Mode 10" class="Ring (strict)"("Visible"=FALSE) -> ()  [unwired: 2 in, 2 out]
                n426 = property on="Control Mode 9" class="Ring (strict)"("Visible"=FALSE) -> ()  [unwired: 2 in, 2 out]
                n427 = property on="Value String 10" class="Str"("Visible"=FALSE) -> ()  [unwired: 2 in, 2 out]
                n428 = property on="Value String 9" class="Str"("Visible"=FALSE) -> ()  [unwired: 2 in, 2 out]
                n429 = property on="Projector Situation 9" class="Ring (strict)"("Visible"=FALSE) -> ()  [unwired: 2 in, 2 out]
                n430 = property on="Projector Situation 10" class="Ring (strict)"("Visible"=FALSE) -> ()  [unwired: 2 in, 2 out]
                n431 = Format Date/Time String(time format string (%c)="%H:%M:%S", seconds (now)="Time 9") -> (date/time string=w617:string)  [unwired: 1 in]
                n432 = Format Date/Time String(time format string (%c)="%H:%M:%S", seconds (now)="Time 10") -> (date/time string=w616:string)  [unwired: 1 in]
                n433 = property on="Operator 9" class="Ring (strict)"("Disabled Items []"=i32[] []) -> ()  [unwired: 2 in, 2 out]
                n434 = Concatenate Strings("'" ("string"), w617, "'" ("string")) -> (w608:string)
                n435 = Concatenate Strings("'" ("string"), w616, "'" ("string")) -> (w607:string)
              }
              frame 3 {
                n436 = property on="Date 10" class="AbsTime (strict)"("Visible"=FALSE) -> ()  [unwired: 2 in, 2 out]
                n437 = property on="Time 10" class="AbsTime (strict)"("Visible"=FALSE) -> ()  [unwired: 2 in, 2 out]
                n438 = property on="Date 9" class="AbsTime (strict)"("Visible"=FALSE) -> ()  [unwired: 2 in, 2 out]
                n439 = property on="Time 9" class="AbsTime (strict)"("Visible"=FALSE) -> ()  [unwired: 2 in, 2 out]
                n440 = property on="Disc Situation 9" class="Ring (strict)"("Visible"=TRUE) -> ()  [unwired: 2 in, 2 out]
                n441 = property on="Disc Situation 10" class="Ring (strict)"("Visible"=TRUE) -> ()  [unwired: 2 in, 2 out]
                n442 = property on="Camera Situation 10" class="Ring (strict)"("Visible"=FALSE) -> ()  [unwired: 2 in, 2 out]
                n443 = property on="Camera Situation 9" class="Ring (strict)"("Visible"=FALSE) -> ()  [unwired: 2 in, 2 out]
                n444 = property on="Control Mode 10" class="Ring (strict)"("Visible"=FALSE) -> ()  [unwired: 2 in, 2 out]
                n445 = property on="Control Mode 9" class="Ring (strict)"("Visible"=FALSE) -> ()  [unwired: 2 in, 2 out]
                n446 = property on="Value String 10" class="Str"("Visible"=FALSE) -> ()  [unwired: 2 in, 2 out]
                n447 = property on="Value String 9" class="Str"("Visible"=FALSE) -> ()  [unwired: 2 in, 2 out]
                n448 = case shown="0, Default" "Disc Situation 9" {
                  tunnel: ["'Stop'" "'Run'"] -> w636
                  frame 0, Default {
                  }
                  frame 1 {
                  }
                }
                n449 = property on="Projector Situation 9" class="Ring (strict)"("Visible"=FALSE) -> ()  [unwired: 2 in, 2 out]
                n450 = property on="Projector Situation 10" class="Ring (strict)"("Visible"=FALSE) -> ()  [unwired: 2 in, 2 out]
                n451 = property on="Operator 9" class="Ring (strict)"("Disabled Items []"=i32[] [2, 3, 4, 5, 6, 7, 8, 9, 10]) -> ()  [unwired: 2 in, 2 out]
              }
              frame 4 {
                n452 = property on="Date 10" class="AbsTime (strict)"("Visible"=FALSE) -> ()  [unwired: 2 in, 2 out]
                n453 = property on="Time 10" class="AbsTime (strict)"("Visible"=FALSE) -> ()  [unwired: 2 in, 2 out]
                n454 = property on="Date 9" class="AbsTime (strict)"("Visible"=FALSE) -> ()  [unwired: 2 in, 2 out]
                n455 = property on="Time 9" class="AbsTime (strict)"("Visible"=FALSE) -> ()  [unwired: 2 in, 2 out]
                n456 = property on="Disc Situation 9" class="Ring (strict)"("Visible"=FALSE) -> ()  [unwired: 2 in, 2 out]
                n457 = property on="Disc Situation 10" class="Ring (strict)"("Visible"=FALSE) -> ()  [unwired: 2 in, 2 out]
                n458 = property on="Camera Situation 10" class="Ring (strict)"("Visible"=FALSE) -> ()  [unwired: 2 in, 2 out]
                n459 = property on="Camera Situation 9" class="Ring (strict)"("Visible"=FALSE) -> ()  [unwired: 2 in, 2 out]
                n460 = property on="Control Mode 10" class="Ring (strict)"("Visible"=TRUE) -> ()  [unwired: 2 in, 2 out]
                n461 = property on="Control Mode 9" class="Ring (strict)"("Visible"=TRUE) -> ()  [unwired: 2 in, 2 out]
                n462 = property on="Value String 10" class="Str"("Visible"=FALSE) -> ()  [unwired: 2 in, 2 out]
                n463 = property on="Value String 9" class="Str"("Visible"=FALSE) -> ()  [unwired: 2 in, 2 out]
                n464 = property on="Projector Situation 9" class="Ring (strict)"("Visible"=FALSE) -> ()  [unwired: 2 in, 2 out]
                n465 = property on="Projector Situation 10" class="Ring (strict)"("Visible"=FALSE) -> ()  [unwired: 2 in, 2 out]
                n466 = case shown="1" "Control Mode 9" {
                  tunnel: ["'Manual'" "'Auto'"] -> w657
                  frame 0, Default {
                  }
                  frame 1 {
                  }
                }
                n467 = property on="Operator 9" class="Ring (strict)"("Disabled Items []"=i32[] [2, 3, 4, 5, 6, 7, 8, 9, 10]) -> ()  [unwired: 2 in, 2 out]
              }
              frame 5 {
                n468 = property on="Date 10" class="AbsTime (strict)"("Visible"=FALSE) -> ()  [unwired: 2 in, 2 out]
                n469 = property on="Time 10" class="AbsTime (strict)"("Visible"=FALSE) -> ()  [unwired: 2 in, 2 out]
                n470 = property on="Date 9" class="AbsTime (strict)"("Visible"=FALSE) -> ()  [unwired: 2 in, 2 out]
                n471 = property on="Time 9" class="AbsTime (strict)"("Visible"=FALSE) -> ()  [unwired: 2 in, 2 out]
                n472 = property on="Disc Situation 9" class="Ring (strict)"("Visible"=FALSE) -> ()  [unwired: 2 in, 2 out]
                n473 = property on="Disc Situation 10" class="Ring (strict)"("Visible"=FALSE) -> ()  [unwired: 2 in, 2 out]
                n474 = property on="Camera Situation 10" class="Ring (strict)"("Visible"=TRUE) -> ()  [unwired: 2 in, 2 out]
                n475 = property on="Camera Situation 9" class="Ring (strict)"("Visible"=TRUE) -> ()  [unwired: 2 in, 2 out]
                n476 = property on="Control Mode 10" class="Ring (strict)"("Visible"=FALSE) -> ()  [unwired: 2 in, 2 out]
                n477 = property on="Control Mode 9" class="Ring (strict)"("Visible"=FALSE) -> ()  [unwired: 2 in, 2 out]
                n478 = property on="Value String 10" class="Str"("Visible"=FALSE) -> ()  [unwired: 2 in, 2 out]
                n479 = property on="Value String 9" class="Str"("Visible"=FALSE) -> ()  [unwired: 2 in, 2 out]
                n480 = property on="Projector Situation 9" class="Ring (strict)"("Visible"=FALSE) -> ()  [unwired: 2 in, 2 out]
                n481 = property on="Projector Situation 10" class="Ring (strict)"("Visible"=FALSE) -> ()  [unwired: 2 in, 2 out]
                n482 = case shown="1" "Camera Situation 9" {
                  tunnel: ["'OFF'" "'ON'"] -> w677
                  frame 0, Default {
                  }
                  frame 1 {
                  }
                }
                n483 = property on="Operator 9" class="Ring (strict)"("Disabled Items []"=i32[] [2, 3, 4, 5, 6, 7, 8, 9, 10]) -> ()  [unwired: 2 in, 2 out]
              }
              frame 6 {
                n484 = property on="Date 10" class="AbsTime (strict)"("Visible"=FALSE) -> ()  [unwired: 2 in, 2 out]
                n485 = property on="Time 10" class="AbsTime (strict)"("Visible"=FALSE) -> ()  [unwired: 2 in, 2 out]
                n486 = property on="Date 9" class="AbsTime (strict)"("Visible"=FALSE) -> ()  [unwired: 2 in, 2 out]
                n487 = property on="Time 9" class="AbsTime (strict)"("Visible"=FALSE) -> ()  [unwired: 2 in, 2 out]
                n488 = property on="Disc Situation 9" class="Ring (strict)"("Visible"=FALSE) -> ()  [unwired: 2 in, 2 out]
                n489 = property on="Disc Situation 10" class="Ring (strict)"("Visible"=FALSE) -> ()  [unwired: 2 in, 2 out]
                n490 = property on="Camera Situation 10" class="Ring (strict)"("Visible"=FALSE) -> ()  [unwired: 2 in, 2 out]
                n491 = property on="Camera Situation 9" class="Ring (strict)"("Visible"=FALSE) -> ()  [unwired: 2 in, 2 out]
                n492 = property on="Control Mode 10" class="Ring (strict)"("Visible"=FALSE) -> ()  [unwired: 2 in, 2 out]
                n493 = property on="Control Mode 9" class="Ring (strict)"("Visible"=FALSE) -> ()  [unwired: 2 in, 2 out]
                n494 = property on="Value String 10" class="Str"("Visible"=FALSE) -> ()  [unwired: 2 in, 2 out]
                n495 = property on="Value String 9" class="Str"("Visible"=FALSE) -> ()  [unwired: 2 in, 2 out]
                n496 = property on="Projector Situation 9" class="Ring (strict)"("Visible"=TRUE) -> ()  [unwired: 2 in, 2 out]
                n497 = property on="Projector Situation 10" class="Ring (strict)"("Visible"=TRUE) -> ()  [unwired: 2 in, 2 out]
                n498 = case shown="0, Default" "Projector Situation 9" {
                  tunnel: ["'OFF'" "'ON'"] -> w698
                  frame 0, Default {
                  }
                  frame 1 {
                  }
                }
                n499 = property on="Operator 9" class="Ring (strict)"("Disabled Items []"=i32[] [2, 3, 4, 5, 6, 7, 8, 9, 10]) -> ()  [unwired: 2 in, 2 out]
              }
            }
          }
        }
        n500 = Build Array(w188, w189, w190, w191, w192) -> (w186:bool[])
        n501 = case shown="True" w174 {
          tunnel: "Parameter 3" -> [_ w1328]
          tunnel: ["" ("format string") w1327] -> w171
          tunnel: ["" ("date/time string") w1326] -> w170
          tunnel: ["" ("date/time string") w1325] -> w169
          frame False {
            w1306 = u16 0 items=["All", "P=V1", "P#V1", "P<V1", "P<=V1", "P>V1", "P>=V1", "V1<P<V2", "V1<=P<V2", "V1<P<=V2", "V1<=P<=V2"] ("Operator 3")
            w1310 = u16 0 items=["Choose parameter", "Date", "Time", "Disc Situation", "Control Mode", "Camera Situation", "Projector Situation"] ("Parameter 3")
            n502 = property on="Projector Situation 4" class="Ring (strict)"("Visible"=FALSE) -> ()  [unwired: 2 in, 2 out]
            n503 = property on="Projector Situation 3" class="Ring (strict)"("Visible"=FALSE) -> ()  [unwired: 2 in, 2 out]
            n504 = property on="Control Mode 3" class="Ring (strict)"("Visible"=FALSE) -> ()  [unwired: 2 in, 2 out]
            n505 = property on="Control Mode 4" class="Ring (strict)"("Visible"=FALSE) -> ()  [unwired: 2 in, 2 out]
            n506 = property on="Camera Situation 3" class="Ring (strict)"("Visible"=FALSE) -> ()  [unwired: 2 in, 2 out]
            n507 = property on="Camera Situation 4" class="Ring (strict)"("Visible"=FALSE) -> ()  [unwired: 2 in, 2 out]
            n508 = property on="Date 3" class="AbsTime (strict)"("Visible"=FALSE) -> ()  [unwired: 2 in, 2 out]
            n509 = property on="Date 4" class="AbsTime (strict)"("Visible"=FALSE) -> ()  [unwired: 2 in, 2 out]
            n510 = property on="Value String 4" class="Str"("Visible"=FALSE) -> ()  [unwired: 2 in, 2 out]
            n511 = property on="Value String 3" class="Str"("Visible"=FALSE) -> ()  [unwired: 2 in, 2 out]
            n512 = property on="Disc Situation 3" class="Ring (strict)"("Visible"=FALSE) -> ()  [unwired: 2 in, 2 out]
            n513 = property on="Disc Situation 4" class="Ring (strict)"("Visible"=FALSE) -> ()  [unwired: 2 in, 2 out]
            n514 = property on="Parameter 3" class="Ring (strict)"("Value"=w1310) -> ()  [unwired: 2 in, 2 out]
            n515 = property on="Operator 3" class="Ring (strict)"("Value"=w1306) -> ()  [unwired: 2 in, 2 out]
            n516 = property on="Time 3" class="AbsTime (strict)"("Visible"=FALSE) -> ()  [unwired: 2 in, 2 out]
            n517 = property on="Time 4" class="AbsTime (strict)"("Visible"=FALSE) -> ()  [unwired: 2 in, 2 out]
          }
          frame True {
            n518 = case shown="0, Default" w1328 {
              tunnel: ["" ("format string") "date" ("format string") "time" ("format string") "disc_situation" ("format string") "control_mode" ("format string") "camera_situation" ("format string") "projector_situation" ("format string")] -> w1327
              tunnel: ["" ("date/time string") w1349 w1379 w1406 w1427 w1448 w1469] -> w1326
              tunnel: ["" ("date/time string") w1348 w1378 "" ("date/time string") "" ("date/time string") "" ("date/time string") "" ("date/time string")] -> w1325
              frame 0, Default {
                w1329 = u16 0 items=["All", "P=V1", "P#V1", "P<V1", "P<=V1", "P>V1", "P>=V1", "V1<P<V2", "V1<=P<V2", "V1<P<=V2", "V1<=P<=V2"] ("Operator 3")
                n519 = property on="Projector Situation 4" class="Ring (strict)"("Visible"=FALSE) -> ()  [unwired: 2 in, 2 out]
                n520 = property on="Projector Situation 3" class="Ring (strict)"("Visible"=FALSE) -> ()  [unwired: 2 in, 2 out]
                n521 = property on="Control Mode 3" class="Ring (strict)"("Visible"=FALSE) -> ()  [unwired: 2 in, 2 out]
                n522 = property on="Control Mode 4" class="Ring (strict)"("Visible"=FALSE) -> ()  [unwired: 2 in, 2 out]
                n523 = property on="Camera Situation 3" class="Ring (strict)"("Visible"=FALSE) -> ()  [unwired: 2 in, 2 out]
                n524 = property on="Camera Situation 4" class="Ring (strict)"("Visible"=FALSE) -> ()  [unwired: 2 in, 2 out]
                n525 = property on="Date 3" class="AbsTime (strict)"("Visible"=FALSE) -> ()  [unwired: 2 in, 2 out]
                n526 = property on="Date 4" class="AbsTime (strict)"("Visible"=FALSE) -> ()  [unwired: 2 in, 2 out]
                n527 = property on="Operator 3" class="Ring (strict)"("Disabled Items []"=i32[] [1, 2, 3, 4, 5, 6, 7, 8, 9, 10], "Value"=w1329) -> ()  [unwired: 2 in, 2 out]
                n528 = property on="Value String 4" class="Str"("Visible"=TRUE) -> ()  [unwired: 2 in, 2 out]
                n529 = property on="Value String 3" class="Str"("Visible"=TRUE) -> ()  [unwired: 2 in, 2 out]
                n530 = property on="Disc Situation 3" class="Ring (strict)"("Visible"=FALSE) -> ()  [unwired: 2 in, 2 out]
                n531 = property on="Disc Situation 4" class="Ring (strict)"("Visible"=FALSE) -> ()  [unwired: 2 in, 2 out]
                n532 = property on="Time 3" class="AbsTime (strict)"("Visible"=FALSE) -> ()  [unwired: 2 in, 2 out]
                n533 = property on="Time 4" class="AbsTime (strict)"("Visible"=FALSE) -> ()  [unwired: 2 in, 2 out]
              }
              frame 1 {
                n534 = property on="Projector Situation 4" class="Ring (strict)"("Visible"=FALSE) -> ()  [unwired: 2 in, 2 out]
                n535 = property on="Projector Situation 3" class="Ring (strict)"("Visible"=FALSE) -> ()  [unwired: 2 in, 2 out]
                n536 = property on="Control Mode 3" class="Ring (strict)"("Visible"=FALSE) -> ()  [unwired: 2 in, 2 out]
                n537 = property on="Control Mode 4" class="Ring (strict)"("Visible"=FALSE) -> ()  [unwired: 2 in, 2 out]
                n538 = property on="Camera Situation 3" class="Ring (strict)"("Visible"=FALSE) -> ()  [unwired: 2 in, 2 out]
                n539 = property on="Camera Situation 4" class="Ring (strict)"("Visible"=FALSE) -> ()  [unwired: 2 in, 2 out]
                n540 = property on="Date 3" class="AbsTime (strict)"("Visible"=TRUE) -> ()  [unwired: 2 in, 2 out]
                n541 = property on="Date 4" class="AbsTime (strict)"("Visible"=TRUE) -> ()  [unwired: 2 in, 2 out]
                n542 = property on="Value String 4" class="Str"("Visible"=FALSE) -> ()  [unwired: 2 in, 2 out]
                n543 = property on="Value String 3" class="Str"("Visible"=FALSE) -> ()  [unwired: 2 in, 2 out]
                n544 = Format Date/Time String(time format string (%c)="%Y/%m/%d", seconds (now)="Date 4") -> (date/time string=w1360:string)  [unwired: 1 in]
                n545 = Format Date/Time String(time format string (%c)="%Y/%m/%d", seconds (now)="Date 3") -> (date/time string=w1359:string)  [unwired: 1 in]
                n546 = property on="Disc Situation 3" class="Ring (strict)"("Visible"=FALSE) -> ()  [unwired: 2 in, 2 out]
                n547 = property on="Disc Situation 4" class="Ring (strict)"("Visible"=FALSE) -> ()  [unwired: 2 in, 2 out]
                n548 = Concatenate Strings("'" ("string"), w1359, "'" ("string")) -> (w1349:string)
                n549 = Concatenate Strings("'" ("string"), w1360, "'" ("string")) -> (w1348:string)
                n550 = property on="Time 3" class="AbsTime (strict)"("Visible"=FALSE) -> ()  [unwired: 2 in, 2 out]
                n551 = property on="Time 4" class="AbsTime (strict)"("Visible"=FALSE) -> ()  [unwired: 2 in, 2 out]
                n552 = property on="Operator 3" class="Ring (strict)"("Disabled Items []"=i32[] []) -> ()  [unwired: 2 in, 2 out]
              }
              frame 2 {
                n553 = property on="Projector Situation 4" class="Ring (strict)"("Visible"=FALSE) -> ()  [unwired: 2 in, 2 out]
                n554 = property on="Projector Situation 3" class="Ring (strict)"("Visible"=FALSE) -> ()  [unwired: 2 in, 2 out]
                n555 = property on="Control Mode 3" class="Ring (strict)"("Visible"=FALSE) -> ()  [unwired: 2 in, 2 out]
                n556 = property on="Control Mode 4" class="Ring (strict)"("Visible"=FALSE) -> ()  [unwired: 2 in, 2 out]
                n557 = property on="Camera Situation 3" class="Ring (strict)"("Visible"=FALSE) -> ()  [unwired: 2 in, 2 out]
                n558 = property on="Camera Situation 4" class="Ring (strict)"("Visible"=FALSE) -> ()  [unwired: 2 in, 2 out]
                n559 = property on="Date 3" class="AbsTime (strict)"("Visible"=FALSE) -> ()  [unwired: 2 in, 2 out]
                n560 = property on="Date 4" class="AbsTime (strict)"("Visible"=FALSE) -> ()  [unwired: 2 in, 2 out]
                n561 = property on="Operator 3" class="Ring (strict)"("Disabled Items []"=i32[] []) -> ()  [unwired: 2 in, 2 out]
                n562 = property on="Value String 4" class="Str"("Visible"=FALSE) -> ()  [unwired: 2 in, 2 out]
                n563 = property on="Value String 3" class="Str"("Visible"=FALSE) -> ()  [unwired: 2 in, 2 out]
                n564 = property on="Disc Situation 3" class="Ring (strict)"("Visible"=FALSE) -> ()  [unwired: 2 in, 2 out]
                n565 = property on="Disc Situation 4" class="Ring (strict)"("Visible"=FALSE) -> ()  [unwired: 2 in, 2 out]
                n566 = Format Date/Time String(time format string (%c)="%H:%M:%S", seconds (now)="Time 3") -> (date/time string=w1376:string)  [unwired: 1 in]
                n567 = Format Date/Time String(time format string (%c)="%H:%M:%S", seconds (now)="Time 4") -> (date/time string=w1377:string)  [unwired: 1 in]
                n568 = property on="Time 3" class="AbsTime (strict)"("Visible"=TRUE) -> ()  [unwired: 2 in, 2 out]
                n569 = property on="Time 4" class="AbsTime (strict)"("Visible"=TRUE) -> ()  [unwired: 2 in, 2 out]
                n570 = Concatenate Strings("'" ("string"), w1376, "'" ("string")) -> (w1379:string)
                n571 = Concatenate Strings("'" ("string"), w1377, "'" ("string")) -> (w1378:string)
              }
              frame 3 {
                n572 = property on="Projector Situation 4" class="Ring (strict)"("Visible"=FALSE) -> ()  [unwired: 2 in, 2 out]
                n573 = property on="Projector Situation 3" class="Ring (strict)"("Visible"=FALSE) -> ()  [unwired: 2 in, 2 out]
                n574 = property on="Control Mode 3" class="Ring (strict)"("Visible"=FALSE) -> ()  [unwired: 2 in, 2 out]
                n575 = property on="Control Mode 4" class="Ring (strict)"("Visible"=FALSE) -> ()  [unwired: 2 in, 2 out]
                n576 = property on="Camera Situation 3" class="Ring (strict)"("Visible"=FALSE) -> ()  [unwired: 2 in, 2 out]
                n577 = property on="Camera Situation 4" class="Ring (strict)"("Visible"=FALSE) -> ()  [unwired: 2 in, 2 out]
                n578 = property on="Date 3" class="AbsTime (strict)"("Visible"=FALSE) -> ()  [unwired: 2 in, 2 out]
                n579 = property on="Date 4" class="AbsTime (strict)"("Visible"=FALSE) -> ()  [unwired: 2 in, 2 out]
                n580 = property on="Value String 4" class="Str"("Visible"=FALSE) -> ()  [unwired: 2 in, 2 out]
                n581 = property on="Value String 3" class="Str"("Visible"=FALSE) -> ()  [unwired: 2 in, 2 out]
                n582 = property on="Disc Situation 3" class="Ring (strict)"("Visible"=TRUE) -> ()  [unwired: 2 in, 2 out]
                n583 = property on="Disc Situation 4" class="Ring (strict)"("Visible"=TRUE) -> ()  [unwired: 2 in, 2 out]
                n584 = case shown="0, Default" "Disc Situation 3" {
                  tunnel: ["'Stop'" "'Run'"] -> w1406
                  frame 0, Default {
                  }
                  frame 1 {
                  }
                }
                n585 = property on="Time 3" class="AbsTime (strict)"("Visible"=FALSE) -> ()  [unwired: 2 in, 2 out]
                n586 = property on="Time 4" class="AbsTime (strict)"("Visible"=FALSE) -> ()  [unwired: 2 in, 2 out]
                n587 = property on="Operator 3" class="Ring (strict)"("Disabled Items []"=i32[] [2, 3, 4, 5, 6, 7, 8, 9, 10]) -> ()  [unwired: 2 in, 2 out]
              }
              frame 4 {
                n588 = property on="Projector Situation 4" class="Ring (strict)"("Visible"=FALSE) -> ()  [unwired: 2 in, 2 out]
                n589 = property on="Projector Situation 3" class="Ring (strict)"("Visible"=FALSE) -> ()  [unwired: 2 in, 2 out]
                n590 = property on="Control Mode 3" class="Ring (strict)"("Visible"=TRUE) -> ()  [unwired: 2 in, 2 out]
                n591 = property on="Control Mode 4" class="Ring (strict)"("Visible"=TRUE) -> ()  [unwired: 2 in, 2 out]
                n592 = property on="Camera Situation 3" class="Ring (strict)"("Visible"=FALSE) -> ()  [unwired: 2 in, 2 out]
                n593 = property on="Camera Situation 4" class="Ring (strict)"("Visible"=FALSE) -> ()  [unwired: 2 in, 2 out]
                n594 = property on="Date 3" class="AbsTime (strict)"("Visible"=FALSE) -> ()  [unwired: 2 in, 2 out]
                n595 = property on="Date 4" class="AbsTime (strict)"("Visible"=FALSE) -> ()  [unwired: 2 in, 2 out]
                n596 = property on="Value String 4" class="Str"("Visible"=FALSE) -> ()  [unwired: 2 in, 2 out]
                n597 = property on="Value String 3" class="Str"("Visible"=FALSE) -> ()  [unwired: 2 in, 2 out]
                n598 = property on="Disc Situation 3" class="Ring (strict)"("Visible"=FALSE) -> ()  [unwired: 2 in, 2 out]
                n599 = property on="Disc Situation 4" class="Ring (strict)"("Visible"=FALSE) -> ()  [unwired: 2 in, 2 out]
                n600 = case shown="1" "Control Mode 3" {
                  tunnel: ["'Manual'" "'Auto'"] -> w1427
                  frame 0, Default {
                  }
                  frame 1 {
                  }
                }
                n601 = property on="Time 3" class="AbsTime (strict)"("Visible"=FALSE) -> ()  [unwired: 2 in, 2 out]
                n602 = property on="Time 4" class="AbsTime (strict)"("Visible"=FALSE) -> ()  [unwired: 2 in, 2 out]
                n603 = property on="Operator 3" class="Ring (strict)"("Disabled Items []"=i32[] [2, 3, 4, 5, 6, 7, 8, 9, 10]) -> ()  [unwired: 2 in, 2 out]
              }
              frame 5 {
                n604 = property on="Projector Situation 4" class="Ring (strict)"("Visible"=FALSE) -> ()  [unwired: 2 in, 2 out]
                n605 = property on="Projector Situation 3" class="Ring (strict)"("Visible"=FALSE) -> ()  [unwired: 2 in, 2 out]
                n606 = property on="Control Mode 3" class="Ring (strict)"("Visible"=FALSE) -> ()  [unwired: 2 in, 2 out]
                n607 = property on="Control Mode 4" class="Ring (strict)"("Visible"=FALSE) -> ()  [unwired: 2 in, 2 out]
                n608 = property on="Camera Situation 3" class="Ring (strict)"("Visible"=TRUE) -> ()  [unwired: 2 in, 2 out]
                n609 = property on="Camera Situation 4" class="Ring (strict)"("Visible"=TRUE) -> ()  [unwired: 2 in, 2 out]
                n610 = property on="Date 3" class="AbsTime (strict)"("Visible"=FALSE) -> ()  [unwired: 2 in, 2 out]
                n611 = property on="Date 4" class="AbsTime (strict)"("Visible"=FALSE) -> ()  [unwired: 2 in, 2 out]
                n612 = property on="Value String 4" class="Str"("Visible"=FALSE) -> ()  [unwired: 2 in, 2 out]
                n613 = property on="Value String 3" class="Str"("Visible"=FALSE) -> ()  [unwired: 2 in, 2 out]
                n614 = property on="Disc Situation 3" class="Ring (strict)"("Visible"=FALSE) -> ()  [unwired: 2 in, 2 out]
                n615 = property on="Disc Situation 4" class="Ring (strict)"("Visible"=FALSE) -> ()  [unwired: 2 in, 2 out]
                n616 = case shown="1" "Camera Situation 3" {
                  tunnel: ["'OFF'" "'ON'"] -> w1448
                  frame 0, Default {
                  }
                  frame 1 {
                  }
                }
                n617 = property on="Time 3" class="AbsTime (strict)"("Visible"=FALSE) -> ()  [unwired: 2 in, 2 out]
                n618 = property on="Time 4" class="AbsTime (strict)"("Visible"=FALSE) -> ()  [unwired: 2 in, 2 out]
                n619 = property on="Operator 3" class="Ring (strict)"("Disabled Items []"=i32[] [2, 3, 4, 5, 6, 7, 8, 9, 10]) -> ()  [unwired: 2 in, 2 out]
              }
              frame 6 {
                n620 = property on="Projector Situation 4" class="Ring (strict)"("Visible"=TRUE) -> ()  [unwired: 2 in, 2 out]
                n621 = property on="Projector Situation 3" class="Ring (strict)"("Visible"=TRUE) -> ()  [unwired: 2 in, 2 out]
                n622 = property on="Control Mode 3" class="Ring (strict)"("Visible"=FALSE) -> ()  [unwired: 2 in, 2 out]
                n623 = property on="Control Mode 4" class="Ring (strict)"("Visible"=FALSE) -> ()  [unwired: 2 in, 2 out]
                n624 = property on="Camera Situation 3" class="Ring (strict)"("Visible"=FALSE) -> ()  [unwired: 2 in, 2 out]
                n625 = property on="Camera Situation 4" class="Ring (strict)"("Visible"=FALSE) -> ()  [unwired: 2 in, 2 out]
                n626 = property on="Date 3" class="AbsTime (strict)"("Visible"=FALSE) -> ()  [unwired: 2 in, 2 out]
                n627 = property on="Date 4" class="AbsTime (strict)"("Visible"=FALSE) -> ()  [unwired: 2 in, 2 out]
                n628 = property on="Value String 4" class="Str"("Visible"=FALSE) -> ()  [unwired: 2 in, 2 out]
                n629 = property on="Value String 3" class="Str"("Visible"=FALSE) -> ()  [unwired: 2 in, 2 out]
                n630 = property on="Disc Situation 3" class="Ring (strict)"("Visible"=FALSE) -> ()  [unwired: 2 in, 2 out]
                n631 = property on="Disc Situation 4" class="Ring (strict)"("Visible"=FALSE) -> ()  [unwired: 2 in, 2 out]
                n632 = case shown="0, Default" "Projector Situation 3" {
                  tunnel: ["'OFF'" "'ON'"] -> w1469
                  frame 0, Default {
                  }
                  frame 1 {
                  }
                }
                n633 = property on="Time 3" class="AbsTime (strict)"("Visible"=FALSE) -> ()  [unwired: 2 in, 2 out]
                n634 = property on="Time 4" class="AbsTime (strict)"("Visible"=FALSE) -> ()  [unwired: 2 in, 2 out]
                n635 = property on="Operator 3" class="Ring (strict)"("Disabled Items []"=i32[] [2, 3, 4, 5, 6, 7, 8, 9, 10]) -> ()  [unwired: 2 in, 2 out]
              }
            }
          }
        }
        n636 = case shown="True" w173 {
          tunnel: "Parameter 5" -> [_ w1144]
          tunnel: ["" ("format string") w1143] -> w167
          tunnel: ["" ("date/time string") w1142] -> w166
          tunnel: ["" ("date/time string") w1141] -> w165
          frame False {
            w1125 = u16 0 items=["Choose parameter", "Date", "Time", "Disc Situation", "Control Mode", "Camera Situation", "Projector Situation"] ("Parameter 5")
            w1126 = u16 0 items=["All", "P=V1", "P#V1", "P<V1", "P<=V1", "P>V1", "P>=V1", "V1<P<V2", "V1<=P<V2", "V1<P<=V2", "V1<=P<=V2"] ("Operator 5")
            n637 = property on="Time 5" class="AbsTime (strict)"("Visible"=FALSE) -> ()  [unwired: 2 in, 2 out]
            n638 = property on="Time 6" class="AbsTime (strict)"("Visible"=FALSE) -> ()  [unwired: 2 in, 2 out]
            n639 = property on="Disc Situation 5" class="Ring (strict)"("Visible"=FALSE) -> ()  [unwired: 2 in, 2 out]
            n640 = property on="Disc Situation 6" class="Ring (strict)"("Visible"=FALSE) -> ()  [unwired: 2 in, 2 out]
            n641 = property on="Camera Situation 5" class="Ring (strict)"("Visible"=FALSE) -> ()  [unwired: 2 in, 2 out]
            n642 = property on="Camera Situation 6" class="Ring (strict)"("Visible"=FALSE) -> ()  [unwired: 2 in, 2 out]
            n643 = property on="Projector Situation 5" class="Ring (strict)"("Visible"=FALSE) -> ()  [unwired: 2 in, 2 out]
            n644 = property on="Projector Situation 6" class="Ring (strict)"("Visible"=FALSE) -> ()  [unwired: 2 in, 2 out]
            n645 = property on="Value String 6" class="Str"("Visible"=FALSE) -> ()  [unwired: 2 in, 2 out]
            n646 = property on="Date 5" class="AbsTime (strict)"("Visible"=FALSE) -> ()  [unwired: 2 in, 2 out]
            n647 = property on="Date 6" class="AbsTime (strict)"("Visible"=FALSE) -> ()  [unwired: 2 in, 2 out]
            n648 = property on="Value String 5" class="Str"("Visible"=FALSE) -> ()  [unwired: 2 in, 2 out]
            n649 = property on="Operator 5" class="Ring (strict)"("Value"=w1126) -> ()  [unwired: 2 in, 2 out]
            n650 = property on="Parameter 5" class="Ring (strict)"("Value"=w1125) -> ()  [unwired: 2 in, 2 out]
            n651 = property on="Control Mode 5" class="Ring (strict)"("Visible"=FALSE) -> ()  [unwired: 2 in, 2 out]
            n652 = property on="Control Mode 6" class="Ring (strict)"("Visible"=FALSE) -> ()  [unwired: 2 in, 2 out]
          }
          frame True {
            n653 = case shown="0, Default" w1144 {
              tunnel: ["" ("format string") "date" ("format string") "time" ("format string") "disc_situation" ("format string") "control_mode" ("format string") "camera_situation" ("format string") "projector_situation" ("format string")] -> w1143
              tunnel: ["" ("date/time string") w1165 w1195 w1223 w1243 w1264 w1285] -> w1142
              tunnel: ["" ("date/time string") w1164 w1194 "" ("date/time string") "" ("date/time string") "" ("date/time string") "" ("date/time string")] -> w1141
              frame 0, Default {
                w1145 = u16 0 items=["All", "P=V1", "P#V1", "P<V1", "P<=V1", "P>V1", "P>=V1", "V1<P<V2", "V1<=P<V2", "V1<P<=V2", "V1<=P<=V2"] ("Operator 5")
                n654 = property on="Time 5" class="AbsTime (strict)"("Visible"=FALSE) -> ()  [unwired: 2 in, 2 out]
                n655 = property on="Time 6" class="AbsTime (strict)"("Visible"=FALSE) -> ()  [unwired: 2 in, 2 out]
                n656 = property on="Disc Situation 5" class="Ring (strict)"("Visible"=FALSE) -> ()  [unwired: 2 in, 2 out]
                n657 = property on="Disc Situation 6" class="Ring (strict)"("Visible"=FALSE) -> ()  [unwired: 2 in, 2 out]
                n658 = property on="Camera Situation 5" class="Ring (strict)"("Visible"=FALSE) -> ()  [unwired: 2 in, 2 out]
                n659 = property on="Camera Situation 6" class="Ring (strict)"("Visible"=FALSE) -> ()  [unwired: 2 in, 2 out]
                n660 = property on="Projector Situation 5" class="Ring (strict)"("Visible"=FALSE) -> ()  [unwired: 2 in, 2 out]
                n661 = property on="Projector Situation 6" class="Ring (strict)"("Visible"=FALSE) -> ()  [unwired: 2 in, 2 out]
                n662 = property on="Value String 6" class="Str"("Visible"=TRUE) -> ()  [unwired: 2 in, 2 out]
                n663 = property on="Date 5" class="AbsTime (strict)"("Visible"=FALSE) -> ()  [unwired: 2 in, 2 out]
                n664 = property on="Date 6" class="AbsTime (strict)"("Visible"=FALSE) -> ()  [unwired: 2 in, 2 out]
                n665 = property on="Value String 5" class="Str"("Visible"=TRUE) -> ()  [unwired: 2 in, 2 out]
                n666 = property on="Control Mode 5" class="Ring (strict)"("Visible"=FALSE) -> ()  [unwired: 2 in, 2 out]
                n667 = property on="Control Mode 6" class="Ring (strict)"("Visible"=FALSE) -> ()  [unwired: 2 in, 2 out]
                n668 = property on="Operator 5" class="Ring (strict)"("Disabled Items []"=i32[] [1, 2, 3, 4, 5, 6, 7, 8, 9, 10], "Value"=w1145) -> ()  [unwired: 2 in, 2 out]
              }
              frame 1 {
                n669 = property on="Time 5" class="AbsTime (strict)"("Visible"=FALSE) -> ()  [unwired: 2 in, 2 out]
                n670 = property on="Time 6" class="AbsTime (strict)"("Visible"=FALSE) -> ()  [unwired: 2 in, 2 out]
                n671 = property on="Disc Situation 5" class="Ring (strict)"("Visible"=FALSE) -> ()  [unwired: 2 in, 2 out]
                n672 = property on="Disc Situation 6" class="Ring (strict)"("Visible"=FALSE) -> ()  [unwired: 2 in, 2 out]
                n673 = property on="Camera Situation 5" class="Ring (strict)"("Visible"=FALSE) -> ()  [unwired: 2 in, 2 out]
                n674 = property on="Camera Situation 6" class="Ring (strict)"("Visible"=FALSE) -> ()  [unwired: 2 in, 2 out]
                n675 = property on="Projector Situation 5" class="Ring (strict)"("Visible"=FALSE) -> ()  [unwired: 2 in, 2 out]
                n676 = property on="Projector Situation 6" class="Ring (strict)"("Visible"=FALSE) -> ()  [unwired: 2 in, 2 out]
                n677 = property on="Value String 6" class="Str"("Visible"=FALSE) -> ()  [unwired: 2 in, 2 out]
                n678 = property on="Date 5" class="AbsTime (strict)"("Visible"=TRUE) -> ()  [unwired: 2 in, 2 out]
                n679 = property on="Date 6" class="AbsTime (strict)"("Visible"=TRUE) -> ()  [unwired: 2 in, 2 out]
                n680 = property on="Value String 5" class="Str"("Visible"=FALSE) -> ()  [unwired: 2 in, 2 out]
                n681 = Format Date/Time String(time format string (%c)="%Y/%m/%d", seconds (now)="Date 6") -> (date/time string=w1169:string)  [unwired: 1 in]
                n682 = Format Date/Time String(time format string (%c)="%Y/%m/%d", seconds (now)="Date 5") -> (date/time string=w1170:string)  [unwired: 1 in]
                n683 = property on="Control Mode 5" class="Ring (strict)"("Visible"=FALSE) -> ()  [unwired: 2 in, 2 out]
                n684 = property on="Control Mode 6" class="Ring (strict)"("Visible"=FALSE) -> ()  [unwired: 2 in, 2 out]
                n685 = property on="Operator 5" class="Ring (strict)"("Disabled Items []"=i32[] []) -> ()  [unwired: 2 in, 2 out]
                n686 = Concatenate Strings("'" ("string"), w1170, "'" ("string")) -> (w1165:string)
                n687 = Concatenate Strings("'" ("string"), w1169, "'" ("string")) -> (w1164:string)
              }
              frame 2 {
                n688 = property on="Time 5" class="AbsTime (strict)"("Visible"=TRUE) -> ()  [unwired: 2 in, 2 out]
                n689 = property on="Time 6" class="AbsTime (strict)"("Visible"=TRUE) -> ()  [unwired: 2 in, 2 out]
                n690 = property on="Disc Situation 5" class="Ring (strict)"("Visible"=FALSE) -> ()  [unwired: 2 in, 2 out]
                n691 = property on="Disc Situation 6" class="Ring (strict)"("Visible"=FALSE) -> ()  [unwired: 2 in, 2 out]
                n692 = property on="Camera Situation 5" class="Ring (strict)"("Visible"=FALSE) -> ()  [unwired: 2 in, 2 out]
                n693 = property on="Camera Situation 6" class="Ring (strict)"("Visible"=FALSE) -> ()  [unwired: 2 in, 2 out]
                n694 = property on="Projector Situation 5" class="Ring (strict)"("Visible"=FALSE) -> ()  [unwired: 2 in, 2 out]
                n695 = property on="Projector Situation 6" class="Ring (strict)"("Visible"=FALSE) -> ()  [unwired: 2 in, 2 out]
                n696 = property on="Value String 6" class="Str"("Visible"=FALSE) -> ()  [unwired: 2 in, 2 out]
                n697 = property on="Date 5" class="AbsTime (strict)"("Visible"=FALSE) -> ()  [unwired: 2 in, 2 out]
                n698 = property on="Date 6" class="AbsTime (strict)"("Visible"=FALSE) -> ()  [unwired: 2 in, 2 out]
                n699 = property on="Value String 5" class="Str"("Visible"=FALSE) -> ()  [unwired: 2 in, 2 out]
                n700 = Format Date/Time String(time format string (%c)="%H:%M:%S", seconds (now)="Time 5") -> (date/time string=w1192:string)  [unwired: 1 in]
                n701 = Format Date/Time String(time format string (%c)="%H:%M:%S", seconds (now)="Time 6") -> (date/time string=w1193:string)  [unwired: 1 in]
                n702 = property on="Control Mode 5" class="Ring (strict)"("Visible"=FALSE) -> ()  [unwired: 2 in, 2 out]
                n703 = property on="Control Mode 6" class="Ring (strict)"("Visible"=FALSE) -> ()  [unwired: 2 in, 2 out]
                n704 = property on="Operator 5" class="Ring (strict)"("Disabled Items []"=i32[] []) -> ()  [unwired: 2 in, 2 out]
                n705 = Concatenate Strings("'" ("string"), w1192, "'" ("string")) -> (w1195:string)
                n706 = Concatenate Strings("'" ("string"), w1193, "'" ("string")) -> (w1194:string)
              }
              frame 3 {
                n707 = property on="Time 5" class="AbsTime (strict)"("Visible"=FALSE) -> ()  [unwired: 2 in, 2 out]
                n708 = property on="Time 6" class="AbsTime (strict)"("Visible"=FALSE) -> ()  [unwired: 2 in, 2 out]
                n709 = property on="Disc Situation 5" class="Ring (strict)"("Visible"=TRUE) -> ()  [unwired: 2 in, 2 out]
                n710 = property on="Disc Situation 6" class="Ring (strict)"("Visible"=TRUE) -> ()  [unwired: 2 in, 2 out]
                n711 = property on="Camera Situation 5" class="Ring (strict)"("Visible"=FALSE) -> ()  [unwired: 2 in, 2 out]
                n712 = property on="Camera Situation 6" class="Ring (strict)"("Visible"=FALSE) -> ()  [unwired: 2 in, 2 out]
                n713 = property on="Projector Situation 5" class="Ring (strict)"("Visible"=FALSE) -> ()  [unwired: 2 in, 2 out]
                n714 = property on="Projector Situation 6" class="Ring (strict)"("Visible"=FALSE) -> ()  [unwired: 2 in, 2 out]
                n715 = property on="Value String 6" class="Str"("Visible"=FALSE) -> ()  [unwired: 2 in, 2 out]
                n716 = property on="Date 5" class="AbsTime (strict)"("Visible"=FALSE) -> ()  [unwired: 2 in, 2 out]
                n717 = property on="Date 6" class="AbsTime (strict)"("Visible"=FALSE) -> ()  [unwired: 2 in, 2 out]
                n718 = property on="Value String 5" class="Str"("Visible"=FALSE) -> ()  [unwired: 2 in, 2 out]
                n719 = case shown="0, Default" "Disc Situation 5" {
                  tunnel: ["'Stop'" "'Run'"] -> w1223
                  frame 0, Default {
                  }
                  frame 1 {
                  }
                }
                n720 = property on="Control Mode 5" class="Ring (strict)"("Visible"=FALSE) -> ()  [unwired: 2 in, 2 out]
                n721 = property on="Control Mode 6" class="Ring (strict)"("Visible"=FALSE) -> ()  [unwired: 2 in, 2 out]
                n722 = property on="Operator 5" class="Ring (strict)"("Disabled Items []"=i32[] [2, 3, 4, 5, 6, 7, 8, 9, 10]) -> ()  [unwired: 2 in, 2 out]
              }
              frame 4 {
                n723 = property on="Time 5" class="AbsTime (strict)"("Visible"=FALSE) -> ()  [unwired: 2 in, 2 out]
                n724 = property on="Time 6" class="AbsTime (strict)"("Visible"=FALSE) -> ()  [unwired: 2 in, 2 out]
                n725 = property on="Disc Situation 5" class="Ring (strict)"("Visible"=FALSE) -> ()  [unwired: 2 in, 2 out]
                n726 = property on="Disc Situation 6" class="Ring (strict)"("Visible"=FALSE) -> ()  [unwired: 2 in, 2 out]
                n727 = property on="Camera Situation 5" class="Ring (strict)"("Visible"=FALSE) -> ()  [unwired: 2 in, 2 out]
                n728 = property on="Camera Situation 6" class="Ring (strict)"("Visible"=FALSE) -> ()  [unwired: 2 in, 2 out]
                n729 = property on="Projector Situation 5" class="Ring (strict)"("Visible"=FALSE) -> ()  [unwired: 2 in, 2 out]
                n730 = property on="Projector Situation 6" class="Ring (strict)"("Visible"=FALSE) -> ()  [unwired: 2 in, 2 out]
                n731 = property on="Value String 6" class="Str"("Visible"=FALSE) -> ()  [unwired: 2 in, 2 out]
                n732 = property on="Date 5" class="AbsTime (strict)"("Visible"=FALSE) -> ()  [unwired: 2 in, 2 out]
                n733 = property on="Date 6" class="AbsTime (strict)"("Visible"=FALSE) -> ()  [unwired: 2 in, 2 out]
                n734 = property on="Value String 5" class="Str"("Visible"=FALSE) -> ()  [unwired: 2 in, 2 out]
                n735 = property on="Control Mode 5" class="Ring (strict)"("Visible"=TRUE) -> ()  [unwired: 2 in, 2 out]
                n736 = property on="Control Mode 6" class="Ring (strict)"("Visible"=TRUE) -> ()  [unwired: 2 in, 2 out]
                n737 = case shown="1" "Control Mode 5" {
                  tunnel: ["'Manual'" "'Auto'"] -> w1243
                  frame 0, Default {
                  }
                  frame 1 {
                  }
                }
                n738 = property on="Operator 5" class="Ring (strict)"("Disabled Items []"=i32[] [2, 3, 4, 5, 6, 7, 8, 9, 10]) -> ()  [unwired: 2 in, 2 out]
              }
              frame 5 {
                n739 = property on="Time 5" class="AbsTime (strict)"("Visible"=FALSE) -> ()  [unwired: 2 in, 2 out]
                n740 = property on="Time 6" class="AbsTime (strict)"("Visible"=FALSE) -> ()  [unwired: 2 in, 2 out]
                n741 = property on="Disc Situation 5" class="Ring (strict)"("Visible"=FALSE) -> ()  [unwired: 2 in, 2 out]
                n742 = property on="Disc Situation 6" class="Ring (strict)"("Visible"=FALSE) -> ()  [unwired: 2 in, 2 out]
                n743 = property on="Camera Situation 5" class="Ring (strict)"("Visible"=TRUE) -> ()  [unwired: 2 in, 2 out]
                n744 = property on="Camera Situation 6" class="Ring (strict)"("Visible"=TRUE) -> ()  [unwired: 2 in, 2 out]
                n745 = property on="Projector Situation 5" class="Ring (strict)"("Visible"=FALSE) -> ()  [unwired: 2 in, 2 out]
                n746 = property on="Projector Situation 6" class="Ring (strict)"("Visible"=FALSE) -> ()  [unwired: 2 in, 2 out]
                n747 = property on="Value String 6" class="Str"("Visible"=FALSE) -> ()  [unwired: 2 in, 2 out]
                n748 = property on="Date 5" class="AbsTime (strict)"("Visible"=FALSE) -> ()  [unwired: 2 in, 2 out]
                n749 = property on="Date 6" class="AbsTime (strict)"("Visible"=FALSE) -> ()  [unwired: 2 in, 2 out]
                n750 = property on="Value String 5" class="Str"("Visible"=FALSE) -> ()  [unwired: 2 in, 2 out]
                n751 = property on="Control Mode 5" class="Ring (strict)"("Visible"=FALSE) -> ()  [unwired: 2 in, 2 out]
                n752 = property on="Control Mode 6" class="Ring (strict)"("Visible"=FALSE) -> ()  [unwired: 2 in, 2 out]
                n753 = case shown="1" "Camera Situation 6" {
                  tunnel: ["'OFF'" "'ON'"] -> w1264
                  frame 0, Default {
                  }
                  frame 1 {
                  }
                }
                n754 = property on="Operator 5" class="Ring (strict)"("Disabled Items []"=i32[] [2, 3, 4, 5, 6, 7, 8, 9, 10]) -> ()  [unwired: 2 in, 2 out]
              }
              frame 6 {
                n755 = property on="Time 5" class="AbsTime (strict)"("Visible"=FALSE) -> ()  [unwired: 2 in, 2 out]
                n756 = property on="Time 6" class="AbsTime (strict)"("Visible"=FALSE) -> ()  [unwired: 2 in, 2 out]
                n757 = property on="Disc Situation 5" class="Ring (strict)"("Visible"=FALSE) -> ()  [unwired: 2 in, 2 out]
                n758 = property on="Disc Situation 6" class="Ring (strict)"("Visible"=FALSE) -> ()  [unwired: 2 in, 2 out]
                n759 = property on="Camera Situation 5" class="Ring (strict)"("Visible"=FALSE) -> ()  [unwired: 2 in, 2 out]
                n760 = property on="Camera Situation 6" class="Ring (strict)"("Visible"=FALSE) -> ()  [unwired: 2 in, 2 out]
                n761 = property on="Projector Situation 5" class="Ring (strict)"("Visible"=TRUE) -> ()  [unwired: 2 in, 2 out]
                n762 = property on="Projector Situation 6" class="Ring (strict)"("Visible"=TRUE) -> ()  [unwired: 2 in, 2 out]
                n763 = property on="Value String 6" class="Str"("Visible"=FALSE) -> ()  [unwired: 2 in, 2 out]
                n764 = property on="Date 5" class="AbsTime (strict)"("Visible"=FALSE) -> ()  [unwired: 2 in, 2 out]
                n765 = property on="Date 6" class="AbsTime (strict)"("Visible"=FALSE) -> ()  [unwired: 2 in, 2 out]
                n766 = property on="Value String 5" class="Str"("Visible"=FALSE) -> ()  [unwired: 2 in, 2 out]
                n767 = property on="Control Mode 5" class="Ring (strict)"("Visible"=FALSE) -> ()  [unwired: 2 in, 2 out]
                n768 = property on="Control Mode 6" class="Ring (strict)"("Visible"=FALSE) -> ()  [unwired: 2 in, 2 out]
                n769 = case shown="0, Default" "Projector Situation 5" {
                  tunnel: ["'OFF'" "'ON'"] -> w1285
                  frame 0, Default {
                  }
                  frame 1 {
                  }
                }
                n770 = property on="Operator 5" class="Ring (strict)"("Disabled Items []"=i32[] [2, 3, 4, 5, 6, 7, 8, 9, 10]) -> ()  [unwired: 2 in, 2 out]
              }
            }
          }
        }
        n771 = case shown="0, Default" "Parameter 1" {
          tunnel: ["" ("date/time string") w1592 w1610 w1641 w1661 w1682 w1703] -> w182
          tunnel: ["" ("date/time string") w1586 w1611 "" ("date/time string") "" ("date/time string") "" ("date/time string") "" ("date/time string")] -> w181
          tunnel: ["" ("format string") "date" ("format string") "time" ("format string") "disc_situation" ("format string") "control_mode" ("format string") "camera_situation" ("format string") "projector_situation" ("format string")] -> w180
          frame 0, Default {
            w1563 = u16 0 items=["All", "P=V1", "P#V1", "P<V1", "P<=V1", "P>V1", "P>=V1", "V1<P<V2", "V1<=P<V2", "V1<P<=V2", "V1<=P<=V2"] ("Operator 1")
            n772 = property on="Value String 2" class="Str"("Visible"=TRUE) -> ()  [unwired: 2 in, 2 out]
            n773 = property on="Value String 1" class="Str"("Visible"=TRUE) -> ()  [unwired: 2 in, 2 out]
            n774 = property on="Date 1" class="AbsTime (strict)"("Visible"=FALSE) -> ()  [unwired: 2 in, 2 out]
            n775 = property on="Date 2" class="AbsTime (strict)"("Visible"=FALSE) -> ()  [unwired: 2 in, 2 out]
            n776 = property on="Operator 1" class="Ring (strict)"("Disabled Items []"=i32[] [1, 2, 3, 4, 5, 6, 7, 8, 9, 10], "Value"=w1563) -> ()  [unwired: 2 in, 2 out]
            n777 = property on="Control Mode 2" class="Ring (strict)"("Visible"=FALSE) -> ()  [unwired: 2 in, 2 out]
            n778 = property on="Control Mode 1" class="Ring (strict)"("Visible"=FALSE) -> ()  [unwired: 2 in, 2 out]
            n779 = property on="Time 1" class="AbsTime (strict)"("Visible"=FALSE) -> ()  [unwired: 2 in, 2 out]
            n780 = property on="Disc Situation 1" class="Ring (strict)"("Visible"=FALSE) -> ()  [unwired: 2 in, 2 out]
            n781 = property on="Camera Situation 1" class="Ring (strict)"("Visible"=FALSE) -> ()  [unwired: 2 in, 2 out]
            n782 = property on="Time 2" class="AbsTime (strict)"("Visible"=FALSE) -> ()  [unwired: 2 in, 2 out]
            n783 = property on="Projector Situation 2" class="Ring (strict)"("Visible"=FALSE) -> ()  [unwired: 2 in, 2 out]
            n784 = property on="Projector Situation 1" class="Ring (strict)"("Visible"=FALSE) -> ()  [unwired: 2 in, 2 out]
            n785 = property on="Camera Situation 2" class="Ring (strict)"("Visible"=FALSE) -> ()  [unwired: 2 in, 2 out]
            n786 = property on="Disc Situation 2" class="Ring (strict)"("Visible"=FALSE) -> ()  [unwired: 2 in, 2 out]
          }
          frame 1 {
            n787 = property on="Projector Situation 2" class="Ring (strict)"("Visible"=FALSE) -> ()  [unwired: 2 in, 2 out]
            n788 = property on="Projector Situation 1" class="Ring (strict)"("Visible"=FALSE) -> ()  [unwired: 2 in, 2 out]
            n789 = property on="Date 1" class="AbsTime (strict)"("Visible"=TRUE) -> ()  [unwired: 2 in, 2 out]
            n790 = property on="Date 2" class="AbsTime (strict)"("Visible"=TRUE) -> ()  [unwired: 2 in, 2 out]
            n791 = property on="Operator 1" class="Ring (strict)"("Disabled Items []"=i32[] []) -> ()  [unwired: 2 in, 2 out]
            n792 = property on="Time 1" class="AbsTime (strict)"("Visible"=FALSE) -> ()  [unwired: 2 in, 2 out]
            n793 = property on="Time 2" class="AbsTime (strict)"("Visible"=FALSE) -> ()  [unwired: 2 in, 2 out]
            n794 = property on="Camera Situation 1" class="Ring (strict)"("Visible"=FALSE) -> ()  [unwired: 2 in, 2 out]
            n795 = property on="Camera Situation 2" class="Ring (strict)"("Visible"=FALSE) -> ()  [unwired: 2 in, 2 out]
            n796 = property on="Disc Situation 2" class="Ring (strict)"("Visible"=FALSE) -> ()  [unwired: 2 in, 2 out]
            n797 = property on="Disc Situation 1" class="Ring (strict)"("Visible"=FALSE) -> ()  [unwired: 2 in, 2 out]
            n798 = Format Date/Time String(time format string (%c)="%Y/%m/%d", seconds (now)="Date 2") -> (date/time string=w1585:string)  [unwired: 1 in]
            n799 = property on="Control Mode 1" class="Ring (strict)"("Visible"=FALSE) -> ()  [unwired: 2 in, 2 out]
            n800 = property on="Control Mode 2" class="Ring (strict)"("Visible"=FALSE) -> ()  [unwired: 2 in, 2 out]
            n801 = Format Date/Time String(time format string (%c)="%Y/%m/%d", seconds (now)="Date 1") -> (date/time string=w1591:string)  [unwired: 1 in]
            n802 = property on="Value String 1" class="Str"("Visible"=FALSE) -> ()  [unwired: 2 in, 2 out]
            n803 = property on="Value String 2" class="Str"("Visible"=FALSE) -> ()  [unwired: 2 in, 2 out]
            n804 = Concatenate Strings("'" ("string"), w1591, "'" ("string")) -> (w1592:string)
            n805 = Concatenate Strings("'" ("string"), w1585, "'" ("string")) -> (w1586:string)
          }
          frame 2 {
            n806 = property on="Projector Situation 2" class="Ring (strict)"("Visible"=FALSE) -> ()  [unwired: 2 in, 2 out]
            n807 = property on="Projector Situation 1" class="Ring (strict)"("Visible"=FALSE) -> ()  [unwired: 2 in, 2 out]
            n808 = property on="Date 1" class="AbsTime (strict)"("Visible"=FALSE) -> ()  [unwired: 2 in, 2 out]
            n809 = property on="Date 2" class="AbsTime (strict)"("Visible"=FALSE) -> ()  [unwired: 2 in, 2 out]
            n810 = property on="Operator 1" class="Ring (strict)"("Disabled Items []"=i32[] []) -> ()  [unwired: 2 in, 2 out]
            n811 = property on="Time 1" class="AbsTime (strict)"("Visible"=TRUE) -> ()  [unwired: 2 in, 2 out]
            n812 = property on="Time 2" class="AbsTime (strict)"("Visible"=TRUE) -> ()  [unwired: 2 in, 2 out]
            n813 = property on="Camera Situation 1" class="Ring (strict)"("Visible"=FALSE) -> ()  [unwired: 2 in, 2 out]
            n814 = property on="Camera Situation 2" class="Ring (strict)"("Visible"=FALSE) -> ()  [unwired: 2 in, 2 out]
            n815 = property on="Disc Situation 2" class="Ring (strict)"("Visible"=FALSE) -> ()  [unwired: 2 in, 2 out]
            n816 = property on="Disc Situation 1" class="Ring (strict)"("Visible"=FALSE) -> ()  [unwired: 2 in, 2 out]
            n817 = property on="Control Mode 1" class="Ring (strict)"("Visible"=FALSE) -> ()  [unwired: 2 in, 2 out]
            n818 = property on="Control Mode 2" class="Ring (strict)"("Visible"=FALSE) -> ()  [unwired: 2 in, 2 out]
            n819 = Format Date/Time String(time format string (%c)="%H:%M:%S", seconds (now)="Time 1") -> (date/time string=w1613:string)  [unwired: 1 in]
            n820 = Format Date/Time String(time format string (%c)="%H:%M:%S", seconds (now)="Time 2") -> (date/time string=w1612:string)  [unwired: 1 in]
            n821 = property on="Value String 1" class="Str"("Visible"=FALSE) -> ()  [unwired: 2 in, 2 out]
            n822 = property on="Value String 2" class="Str"("Visible"=FALSE) -> ()  [unwired: 2 in, 2 out]
            n823 = Concatenate Strings("'" ("string"), w1613, "'" ("string")) -> (w1610:string)
            n824 = Concatenate Strings("'" ("string"), w1612, "'" ("string")) -> (w1611:string)
          }
          frame 3 {
            n825 = property on="Projector Situation 2" class="Ring (strict)"("Visible"=FALSE) -> ()  [unwired: 2 in, 2 out]
            n826 = property on="Projector Situation 1" class="Ring (strict)"("Visible"=FALSE) -> ()  [unwired: 2 in, 2 out]
            n827 = property on="Date 1" class="AbsTime (strict)"("Visible"=FALSE) -> ()  [unwired: 2 in, 2 out]
            n828 = property on="Date 2" class="AbsTime (strict)"("Visible"=FALSE) -> ()  [unwired: 2 in, 2 out]
            n829 = property on="Operator 1" class="Ring (strict)"("Disabled Items []"=i32[] [2, 3, 4, 5, 6, 7, 8, 9, 10]) -> ()  [unwired: 2 in, 2 out]
            n830 = property on="Time 1" class="AbsTime (strict)"("Visible"=FALSE) -> ()  [unwired: 2 in, 2 out]
            n831 = property on="Time 2" class="AbsTime (strict)"("Visible"=FALSE) -> ()  [unwired: 2 in, 2 out]
            n832 = property on="Camera Situation 1" class="Ring (strict)"("Visible"=FALSE) -> ()  [unwired: 2 in, 2 out]
            n833 = property on="Camera Situation 2" class="Ring (strict)"("Visible"=FALSE) -> ()  [unwired: 2 in, 2 out]
            n834 = property on="Disc Situation 2" class="Ring (strict)"("Visible"=TRUE) -> ()  [unwired: 2 in, 2 out]
            n835 = property on="Disc Situation 1" class="Ring (strict)"("Visible"=TRUE) -> ()  [unwired: 2 in, 2 out]
            n836 = case shown="0, Default" "Disc Situation 1" {
              tunnel: ["'Stop'" "'Run'"] -> w1641
              frame 0, Default {
              }
              frame 1 {
              }
            }
            n837 = property on="Control Mode 1" class="Ring (strict)"("Visible"=FALSE) -> ()  [unwired: 2 in, 2 out]
            n838 = property on="Control Mode 2" class="Ring (strict)"("Visible"=FALSE) -> ()  [unwired: 2 in, 2 out]
            n839 = property on="Value String 1" class="Str"("Visible"=FALSE) -> ()  [unwired: 2 in, 2 out]
            n840 = property on="Value String 2" class="Str"("Visible"=FALSE) -> ()  [unwired: 2 in, 2 out]
          }
          frame 4 {
            n841 = property on="Projector Situation 2" class="Ring (strict)"("Visible"=FALSE) -> ()  [unwired: 2 in, 2 out]
            n842 = property on="Projector Situation 1" class="Ring (strict)"("Visible"=FALSE) -> ()  [unwired: 2 in, 2 out]
            n843 = property on="Date 1" class="AbsTime (strict)"("Visible"=FALSE) -> ()  [unwired: 2 in, 2 out]
            n844 = property on="Date 2" class="AbsTime (strict)"("Visible"=FALSE) -> ()  [unwired: 2 in, 2 out]
            n845 = property on="Operator 1" class="Ring (strict)"("Disabled Items []"=i32[] [2, 3, 4, 5, 6, 7, 8, 9, 10]) -> ()  [unwired: 2 in, 2 out]
            n846 = property on="Time 1" class="AbsTime (strict)"("Visible"=FALSE) -> ()  [unwired: 2 in, 2 out]
            n847 = property on="Time 2" class="AbsTime (strict)"("Visible"=FALSE) -> ()  [unwired: 2 in, 2 out]
            n848 = property on="Camera Situation 1" class="Ring (strict)"("Visible"=FALSE) -> ()  [unwired: 2 in, 2 out]
            n849 = property on="Camera Situation 2" class="Ring (strict)"("Visible"=FALSE) -> ()  [unwired: 2 in, 2 out]
            n850 = case shown="1" "Control Mode 1" {
              tunnel: ["'Manual'" "'Auto'"] -> w1661
              frame 0, Default {
              }
              frame 1 {
              }
            }
            n851 = property on="Disc Situation 2" class="Ring (strict)"("Visible"=FALSE) -> ()  [unwired: 2 in, 2 out]
            n852 = property on="Disc Situation 1" class="Ring (strict)"("Visible"=FALSE) -> ()  [unwired: 2 in, 2 out]
            n853 = property on="Control Mode 1" class="Ring (strict)"("Visible"=TRUE) -> ()  [unwired: 2 in, 2 out]
            n854 = property on="Control Mode 2" class="Ring (strict)"("Visible"=TRUE) -> ()  [unwired: 2 in, 2 out]
            n855 = property on="Value String 1" class="Str"("Visible"=FALSE) -> ()  [unwired: 2 in, 2 out]
            n856 = property on="Value String 2" class="Str"("Visible"=FALSE) -> ()  [unwired: 2 in, 2 out]
          }
          frame 5 {
            n857 = property on="Projector Situation 2" class="Ring (strict)"("Visible"=FALSE) -> ()  [unwired: 2 in, 2 out]
            n858 = property on="Projector Situation 1" class="Ring (strict)"("Visible"=FALSE) -> ()  [unwired: 2 in, 2 out]
            n859 = property on="Date 1" class="AbsTime (strict)"("Visible"=FALSE) -> ()  [unwired: 2 in, 2 out]
            n860 = property on="Date 2" class="AbsTime (strict)"("Visible"=FALSE) -> ()  [unwired: 2 in, 2 out]
            n861 = property on="Operator 1" class="Ring (strict)"("Disabled Items []"=i32[] [2, 3, 4, 5, 6, 7, 8, 9, 10]) -> ()  [unwired: 2 in, 2 out]
            n862 = property on="Time 1" class="AbsTime (strict)"("Visible"=FALSE) -> ()  [unwired: 2 in, 2 out]
            n863 = property on="Time 2" class="AbsTime (strict)"("Visible"=FALSE) -> ()  [unwired: 2 in, 2 out]
            n864 = property on="Camera Situation 1" class="Ring (strict)"("Visible"=TRUE) -> ()  [unwired: 2 in, 2 out]
            n865 = property on="Camera Situation 2" class="Ring (strict)"("Visible"=TRUE) -> ()  [unwired: 2 in, 2 out]
            n866 = case shown="1" "Camera Situation 1" {
              tunnel: ["'OFF'" "'ON'"] -> w1682
              frame 0, Default {
              }
              frame 1 {
              }
            }
            n867 = property on="Disc Situation 2" class="Ring (strict)"("Visible"=FALSE) -> ()  [unwired: 2 in, 2 out]
            n868 = property on="Disc Situation 1" class="Ring (strict)"("Visible"=FALSE) -> ()  [unwired: 2 in, 2 out]
            n869 = property on="Control Mode 1" class="Ring (strict)"("Visible"=FALSE) -> ()  [unwired: 2 in, 2 out]
            n870 = property on="Control Mode 2" class="Ring (strict)"("Visible"=FALSE) -> ()  [unwired: 2 in, 2 out]
            n871 = property on="Value String 1" class="Str"("Visible"=FALSE) -> ()  [unwired: 2 in, 2 out]
            n872 = property on="Value String 2" class="Str"("Visible"=FALSE) -> ()  [unwired: 2 in, 2 out]
          }
          frame 6 {
            n873 = property on="Projector Situation 2" class="Ring (strict)"("Visible"=TRUE) -> ()  [unwired: 2 in, 2 out]
            n874 = property on="Projector Situation 1" class="Ring (strict)"("Visible"=TRUE) -> ()  [unwired: 2 in, 2 out]
            n875 = property on="Date 1" class="AbsTime (strict)"("Visible"=FALSE) -> ()  [unwired: 2 in, 2 out]
            n876 = property on="Date 2" class="AbsTime (strict)"("Visible"=FALSE) -> ()  [unwired: 2 in, 2 out]
            n877 = property on="Operator 1" class="Ring (strict)"("Disabled Items []"=i32[] [2, 3, 4, 5, 6, 7, 8, 9, 10]) -> ()  [unwired: 2 in, 2 out]
            n878 = property on="Time 1" class="AbsTime (strict)"("Visible"=FALSE) -> ()  [unwired: 2 in, 2 out]
            n879 = property on="Time 2" class="AbsTime (strict)"("Visible"=FALSE) -> ()  [unwired: 2 in, 2 out]
            n880 = property on="Camera Situation 1" class="Ring (strict)"("Visible"=FALSE) -> ()  [unwired: 2 in, 2 out]
            n881 = property on="Camera Situation 2" class="Ring (strict)"("Visible"=FALSE) -> ()  [unwired: 2 in, 2 out]
            n882 = property on="Disc Situation 2" class="Ring (strict)"("Visible"=FALSE) -> ()  [unwired: 2 in, 2 out]
            n883 = property on="Disc Situation 1" class="Ring (strict)"("Visible"=FALSE) -> ()  [unwired: 2 in, 2 out]
            n884 = property on="Control Mode 1" class="Ring (strict)"("Visible"=FALSE) -> ()  [unwired: 2 in, 2 out]
            n885 = property on="Control Mode 2" class="Ring (strict)"("Visible"=FALSE) -> ()  [unwired: 2 in, 2 out]
            n886 = case shown="0, Default" "Projector Situation 1" {
              tunnel: ["'OFF'" "'ON'"] -> w1703
              frame 0, Default {
              }
              frame 1 {
              }
            }
            n887 = property on="Value String 1" class="Str"("Visible"=FALSE) -> ()  [unwired: 2 in, 2 out]
            n888 = property on="Value String 2" class="Str"("Visible"=FALSE) -> ()  [unwired: 2 in, 2 out]
          }
        }
        n889 = Boolean To (0,1)(Boolean=w186) -> (0, 1=w187:i16[])
        n890 = Add Array Elements(numeric array=w187) -> (sum=w185:i16)
        n891 = case shown="0, Default" w185 {
          frame 0, Default {
            n892 = property on="Parameter 1" class="Ring (strict)"("Visible"=TRUE) -> ()  [unwired: 2 in, 2 out]
            n893 = property on="Operator 1" class="Ring (strict)"("Visible"=TRUE) -> ()  [unwired: 2 in, 2 out]
            n894 = property on="Operator 13" class="Ring (strict)"("Visible"=FALSE) -> ()  [unwired: 2 in, 2 out]
            n895 = property on="Operator 14" class="Ring (strict)"("Visible"=FALSE) -> ()  [unwired: 2 in, 2 out]
            n896 = property on="Parameter 3" class="Ring (strict)"("Visible"=FALSE) -> ()  [unwired: 2 in, 2 out]
            n897 = property on="Operator 3" class="Ring (strict)"("Visible"=FALSE) -> ()  [unwired: 2 in, 2 out]
            n898 = property on="Operator 15" class="Ring (strict)"("Visible"=FALSE) -> ()  [unwired: 2 in, 2 out]
            n899 = property on="Parameter 5" class="Ring (strict)"("Visible"=FALSE) -> ()  [unwired: 2 in, 2 out]
            n900 = property on="Operator 5" class="Ring (strict)"("Visible"=FALSE) -> ()  [unwired: 2 in, 2 out]
            n901 = property on="Operator 16" class="Ring (strict)"("Visible"=FALSE) -> ()  [unwired: 2 in, 2 out]
            n902 = property on="Operator 7" class="Ring (strict)"("Visible"=FALSE) -> ()  [unwired: 2 in, 2 out]
            n903 = property on="Parameter 7" class="Ring (strict)"("Visible"=FALSE) -> ()  [unwired: 2 in, 2 out]
            n904 = property on="Operator 17" class="Ring (strict)"("Visible"=FALSE) -> ()  [unwired: 2 in, 2 out]
            n905 = property on="Operator 9" class="Ring (strict)"("Visible"=FALSE) -> ()  [unwired: 2 in, 2 out]
            n906 = property on="Parameter 9" class="Ring (strict)"("Visible"=FALSE) -> ()  [unwired: 2 in, 2 out]
            n907 = property on="Parameter 11" class="Ring (strict)"("Visible"=FALSE) -> ()  [unwired: 2 in, 2 out]
            n908 = property on="Operator 11" class="Ring (strict)"("Visible"=FALSE) -> ()  [unwired: 2 in, 2 out]
          }
          frame 1 {
            n909 = property on="Operator 13" class="Ring (strict)"("Visible"=TRUE) -> ()  [unwired: 2 in, 2 out]
            n910 = property on="Parameter 1" class="Ring (strict)"("Visible"=TRUE) -> ()  [unwired: 2 in, 2 out]
            n911 = property on="Operator 1" class="Ring (strict)"("Visible"=TRUE) -> ()  [unwired: 2 in, 2 out]
            n912 = property on="Operator 14" class="Ring (strict)"("Visible"=FALSE) -> ()  [unwired: 2 in, 2 out]
            n913 = property on="Parameter 3" class="Ring (strict)"("Visible"=TRUE) -> ()  [unwired: 2 in, 2 out]
            n914 = property on="Operator 3" class="Ring (strict)"("Visible"=TRUE) -> ()  [unwired: 2 in, 2 out]
            n915 = property on="Operator 15" class="Ring (strict)"("Visible"=FALSE) -> ()  [unwired: 2 in, 2 out]
            n916 = property on="Parameter 5" class="Ring (strict)"("Visible"=FALSE) -> ()  [unwired: 2 in, 2 out]
            n917 = property on="Operator 5" class="Ring (strict)"("Visible"=FALSE) -> ()  [unwired: 2 in, 2 out]
            n918 = property on="Operator 16" class="Ring (strict)"("Visible"=FALSE) -> ()  [unwired: 2 in, 2 out]
            n919 = property on="Operator 7" class="Ring (strict)"("Visible"=FALSE) -> ()  [unwired: 2 in, 2 out]
            n920 = property on="Parameter 7" class="Ring (strict)"("Visible"=FALSE) -> ()  [unwired: 2 in, 2 out]
            n921 = property on="Operator 17" class="Ring (strict)"("Visible"=FALSE) -> ()  [unwired: 2 in, 2 out]
            n922 = property on="Operator 9" class="Ring (strict)"("Visible"=FALSE) -> ()  [unwired: 2 in, 2 out]
            n923 = property on="Parameter 9" class="Ring (strict)"("Visible"=FALSE) -> ()  [unwired: 2 in, 2 out]
            n924 = property on="Parameter 11" class="Ring (strict)"("Visible"=FALSE) -> ()  [unwired: 2 in, 2 out]
            n925 = property on="Operator 11" class="Ring (strict)"("Visible"=FALSE) -> ()  [unwired: 2 in, 2 out]
          }
          frame 2 {
            n926 = property on="Parameter 1" class="Ring (strict)"("Visible"=TRUE) -> ()  [unwired: 2 in, 2 out]
            n927 = property on="Operator 1" class="Ring (strict)"("Visible"=TRUE) -> ()  [unwired: 2 in, 2 out]
            n928 = property on="Operator 13" class="Ring (strict)"("Visible"=TRUE) -> ()  [unwired: 2 in, 2 out]
            n929 = property on="Parameter 3" class="Ring (strict)"("Visible"=TRUE) -> ()  [unwired: 2 in, 2 out]
            n930 = property on="Operator 3" class="Ring (strict)"("Visible"=TRUE) -> ()  [unwired: 2 in, 2 out]
            n931 = property on="Operator 14" class="Ring (strict)"("Visible"=TRUE) -> ()  [unwired: 2 in, 2 out]
            n932 = property on="Parameter 5" class="Ring (strict)"("Visible"=TRUE) -> ()  [unwired: 2 in, 2 out]
            n933 = property on="Operator 5" class="Ring (strict)"("Visible"=TRUE) -> ()  [unwired: 2 in, 2 out]
            n934 = property on="Operator 15" class="Ring (strict)"("Visible"=FALSE) -> ()  [unwired: 2 in, 2 out]
            n935 = property on="Operator 7" class="Ring (strict)"("Visible"=FALSE) -> ()  [unwired: 2 in, 2 out]
            n936 = property on="Parameter 7" class="Ring (strict)"("Visible"=FALSE) -> ()  [unwired: 2 in, 2 out]
            n937 = property on="Operator 16" class="Ring (strict)"("Visible"=FALSE) -> ()  [unwired: 2 in, 2 out]
            n938 = property on="Operator 9" class="Ring (strict)"("Visible"=FALSE) -> ()  [unwired: 2 in, 2 out]
            n939 = property on="Parameter 9" class="Ring (strict)"("Visible"=FALSE) -> ()  [unwired: 2 in, 2 out]
            n940 = property on="Operator 17" class="Ring (strict)"("Visible"=FALSE) -> ()  [unwired: 2 in, 2 out]
            n941 = property on="Parameter 11" class="Ring (strict)"("Visible"=FALSE) -> ()  [unwired: 2 in, 2 out]
            n942 = property on="Operator 11" class="Ring (strict)"("Visible"=FALSE) -> ()  [unwired: 2 in, 2 out]
          }
          frame 3 {
            n943 = property on="Parameter 1" class="Ring (strict)"("Visible"=TRUE) -> ()  [unwired: 2 in, 2 out]
            n944 = property on="Operator 1" class="Ring (strict)"("Visible"=TRUE) -> ()  [unwired: 2 in, 2 out]
            n945 = property on="Operator 13" class="Ring (strict)"("Visible"=TRUE) -> ()  [unwired: 2 in, 2 out]
            n946 = property on="Parameter 3" class="Ring (strict)"("Visible"=TRUE) -> ()  [unwired: 2 in, 2 out]
            n947 = property on="Operator 3" class="Ring (strict)"("Visible"=TRUE) -> ()  [unwired: 2 in, 2 out]
            n948 = property on="Operator 14" class="Ring (strict)"("Visible"=TRUE) -> ()  [unwired: 2 in, 2 out]
            n949 = property on="Operator 15" class="Ring (strict)"("Visible"=TRUE) -> ()  [unwired: 2 in, 2 out]
            n950 = property on="Parameter 5" class="Ring (strict)"("Visible"=TRUE) -> ()  [unwired: 2 in, 2 out]
            n951 = property on="Operator 5" class="Ring (strict)"("Visible"=TRUE) -> ()  [unwired: 2 in, 2 out]
            n952 = property on="Operator 16" class="Ring (strict)"("Visible"=FALSE) -> ()  [unwired: 2 in, 2 out]
            n953 = property on="Operator 7" class="Ring (strict)"("Visible"=TRUE) -> ()  [unwired: 2 in, 2 out]
            n954 = property on="Parameter 7" class="Ring (strict)"("Visible"=TRUE) -> ()  [unwired: 2 in, 2 out]
            n955 = property on="Operator 9" class="Ring (strict)"("Visible"=FALSE) -> ()  [unwired: 2 in, 2 out]
            n956 = property on="Parameter 9" class="Ring (strict)"("Visible"=FALSE) -> ()  [unwired: 2 in, 2 out]
            n957 = property on="Operator 17" class="Ring (strict)"("Visible"=FALSE) -> ()  [unwired: 2 in, 2 out]
            n958 = property on="Parameter 11" class="Ring (strict)"("Visible"=FALSE) -> ()  [unwired: 2 in, 2 out]
            n959 = property on="Operator 11" class="Ring (strict)"("Visible"=FALSE) -> ()  [unwired: 2 in, 2 out]
          }
          frame 4 {
            n960 = property on="Operator 13" class="Ring (strict)"("Visible"=TRUE) -> ()  [unwired: 2 in, 2 out]
            n961 = property on="Parameter 1" class="Ring (strict)"("Visible"=TRUE) -> ()  [unwired: 2 in, 2 out]
            n962 = property on="Operator 1" class="Ring (strict)"("Visible"=TRUE) -> ()  [unwired: 2 in, 2 out]
            n963 = property on="Operator 14" class="Ring (strict)"("Visible"=TRUE) -> ()  [unwired: 2 in, 2 out]
            n964 = property on="Parameter 3" class="Ring (strict)"("Visible"=TRUE) -> ()  [unwired: 2 in, 2 out]
            n965 = property on="Operator 3" class="Ring (strict)"("Visible"=TRUE) -> ()  [unwired: 2 in, 2 out]
            n966 = property on="Operator 15" class="Ring (strict)"("Visible"=TRUE) -> ()  [unwired: 2 in, 2 out]
            n967 = property on="Parameter 5" class="Ring (strict)"("Visible"=TRUE) -> ()  [unwired: 2 in, 2 out]
            n968 = property on="Operator 5" class="Ring (strict)"("Visible"=TRUE) -> ()  [unwired: 2 in, 2 out]
            n969 = property on="Operator 16" class="Ring (strict)"("Visible"=TRUE) -> ()  [unwired: 2 in, 2 out]
            n970 = property on="Operator 7" class="Ring (strict)"("Visible"=TRUE) -> ()  [unwired: 2 in, 2 out]
            n971 = property on="Parameter 7" class="Ring (strict)"("Visible"=TRUE) -> ()  [unwired: 2 in, 2 out]
            n972 = property on="Operator 17" class="Ring (strict)"("Visible"=FALSE) -> ()  [unwired: 2 in, 2 out]
            n973 = property on="Operator 9" class="Ring (strict)"("Visible"=TRUE) -> ()  [unwired: 2 in, 2 out]
            n974 = property on="Parameter 9" class="Ring (strict)"("Visible"=TRUE) -> ()  [unwired: 2 in, 2 out]
            n975 = property on="Parameter 11" class="Ring (strict)"("Visible"=FALSE) -> ()  [unwired: 2 in, 2 out]
            n976 = property on="Operator 11" class="Ring (strict)"("Visible"=FALSE) -> ()  [unwired: 2 in, 2 out]
          }
          frame 5 {
            n977 = property on="Parameter 1" class="Ring (strict)"("Visible"=TRUE) -> ()  [unwired: 2 in, 2 out]
            n978 = property on="Operator 1" class="Ring (strict)"("Visible"=TRUE) -> ()  [unwired: 2 in, 2 out]
            n979 = property on="Operator 13" class="Ring (strict)"("Visible"=TRUE) -> ()  [unwired: 2 in, 2 out]
            n980 = property on="Operator 14" class="Ring (strict)"("Visible"=TRUE) -> ()  [unwired: 2 in, 2 out]
            n981 = property on="Parameter 3" class="Ring (strict)"("Visible"=TRUE) -> ()  [unwired: 2 in, 2 out]
            n982 = property on="Operator 3" class="Ring (strict)"("Visible"=TRUE) -> ()  [unwired: 2 in, 2 out]
            n983 = property on="Operator 15" class="Ring (strict)"("Visible"=TRUE) -> ()  [unwired: 2 in, 2 out]
            n984 = property on="Parameter 5" class="Ring (strict)"("Visible"=TRUE) -> ()  [unwired: 2 in, 2 out]
            n985 = property on="Operator 5" class="Ring (strict)"("Visible"=TRUE) -> ()  [unwired: 2 in, 2 out]
            n986 = property on="Operator 16" class="Ring (strict)"("Visible"=TRUE) -> ()  [unwired: 2 in, 2 out]
            n987 = property on="Operator 7" class="Ring (strict)"("Visible"=TRUE) -> ()  [unwired: 2 in, 2 out]
            n988 = property on="Parameter 7" class="Ring (strict)"("Visible"=TRUE) -> ()  [unwired: 2 in, 2 out]
            n989 = property on="Operator 17" class="Ring (strict)"("Visible"=TRUE) -> ()  [unwired: 2 in, 2 out]
            n990 = property on="Operator 9" class="Ring (strict)"("Visible"=TRUE) -> ()  [unwired: 2 in, 2 out]
            n991 = property on="Parameter 9" class="Ring (strict)"("Visible"=TRUE) -> ()  [unwired: 2 in, 2 out]
            n992 = property on="Parameter 11" class="Ring (strict)"("Visible"=TRUE) -> ()  [unwired: 2 in, 2 out]
            n993 = property on="Operator 11" class="Ring (strict)"("Visible"=TRUE) -> ()  [unwired: 2 in, 2 out]
          }
        }
        n994 = case shown="0..6, Default" "Operator 1" {
          frame 0..6, Default {
            w1561 = T1."Disabled and Grayed Out" ("Disabled")
            n995 = property on="Disc Situation 2" class="Ring (strict)"("DisabledEnum"=w1561) -> ()  [unwired: 2 in, 2 out]
            n996 = property on="Value String 2" class="Str"("DisabledEnum"=w1561) -> ()  [unwired: 2 in, 2 out]
            n997 = property on="Time 2" class="AbsTime (strict)"("DisabledEnum"=w1561) -> ()  [unwired: 2 in, 2 out]
            n998 = property on="Date 2" class="AbsTime (strict)"("DisabledEnum"=w1561) -> ()  [unwired: 2 in, 2 out]
            n999 = property on="Projector Situation 2" class="Ring (strict)"("DisabledEnum"=w1561) -> ()  [unwired: 2 in, 2 out]
            n1000 = property on="Control Mode 2" class="Ring (strict)"("DisabledEnum"=w1561) -> ()  [unwired: 2 in, 2 out]
            n1001 = property on="Camera Situation 2" class="Ring (strict)"("DisabledEnum"=w1561) -> ()  [unwired: 2 in, 2 out]
          }
          frame 7..10 {
            w1562 = T1."Enabled" ("Disabled")
            n1002 = property on="Disc Situation 2" class="Ring (strict)"("DisabledEnum"=w1562) -> ()  [unwired: 2 in, 2 out]
            n1003 = property on="Value String 2" class="Str"("DisabledEnum"=w1562) -> ()  [unwired: 2 in, 2 out]
            n1004 = property on="Time 2" class="AbsTime (strict)"("DisabledEnum"=w1562) -> ()  [unwired: 2 in, 2 out]
            n1005 = property on="Date 2" class="AbsTime (strict)"("DisabledEnum"=w1562) -> ()  [unwired: 2 in, 2 out]
            n1006 = property on="Projector Situation 2" class="Ring (strict)"("DisabledEnum"=w1562) -> ()  [unwired: 2 in, 2 out]
            n1007 = property on="Control Mode 2" class="Ring (strict)"("DisabledEnum"=w1562) -> ()  [unwired: 2 in, 2 out]
            n1008 = property on="Camera Situation 2" class="Ring (strict)"("DisabledEnum"=w1562) -> ()  [unwired: 2 in, 2 out]
          }
        }
        n1009 = case shown="7..10" "Operator 3" {
          frame 0..6, Default {
            w1304 = T1."Disabled and Grayed Out" ("Disabled")
            n1010 = property on="Disc Situation 4" class="Ring (strict)"("DisabledEnum"=w1304) -> ()  [unwired: 2 in, 2 out]
            n1011 = property on="Value String 4" class="Str"("DisabledEnum"=w1304) -> ()  [unwired: 2 in, 2 out]
            n1012 = property on="Time 4" class="AbsTime (strict)"("DisabledEnum"=w1304) -> ()  [unwired: 2 in, 2 out]
            n1013 = property on="Date 4" class="AbsTime (strict)"("DisabledEnum"=w1304) -> ()  [unwired: 2 in, 2 out]
            n1014 = property on="Projector Situation 4" class="Ring (strict)"("DisabledEnum"=w1304) -> ()  [unwired: 2 in, 2 out]
            n1015 = property on="Control Mode 4" class="Ring (strict)"("DisabledEnum"=w1304) -> ()  [unwired: 2 in, 2 out]
            n1016 = property on="Camera Situation 4" class="Ring (strict)"("DisabledEnum"=w1304) -> ()  [unwired: 2 in, 2 out]
          }
          frame 7..10 {
            w1305 = T1."Enabled" ("Disabled")
            n1017 = property on="Disc Situation 4" class="Ring (strict)"("DisabledEnum"=w1305) -> ()  [unwired: 2 in, 2 out]
            n1018 = property on="Value String 4" class="Str"("DisabledEnum"=w1305) -> ()  [unwired: 2 in, 2 out]
            n1019 = property on="Time 4" class="AbsTime (strict)"("DisabledEnum"=w1305) -> ()  [unwired: 2 in, 2 out]
            n1020 = property on="Date 4" class="AbsTime (strict)"("DisabledEnum"=w1305) -> ()  [unwired: 2 in, 2 out]
            n1021 = property on="Projector Situation 4" class="Ring (strict)"("DisabledEnum"=w1305) -> ()  [unwired: 2 in, 2 out]
            n1022 = property on="Control Mode 4" class="Ring (strict)"("DisabledEnum"=w1305) -> ()  [unwired: 2 in, 2 out]
            n1023 = property on="Camera Situation 4" class="Ring (strict)"("DisabledEnum"=w1305) -> ()  [unwired: 2 in, 2 out]
          }
        }
        n1024 = case shown="0..6, Default" "Operator 7" {
          frame 0..6, Default {
            w717 = T1."Disabled and Grayed Out" ("Disabled")
            n1025 = property on="Disc Situation 8" class="Ring (strict)"("DisabledEnum"=w717) -> ()  [unwired: 2 in, 2 out]
            n1026 = property on="Value String 8" class="Str"("DisabledEnum"=w717) -> ()  [unwired: 2 in, 2 out]
            n1027 = property on="Time 8" class="AbsTime (strict)"("DisabledEnum"=w717) -> ()  [unwired: 2 in, 2 out]
            n1028 = property on="Date 8" class="AbsTime (strict)"("DisabledEnum"=w717) -> ()  [unwired: 2 in, 2 out]
            n1029 = property on="Projector Situation 8" class="Ring (strict)"("DisabledEnum"=w717) -> ()  [unwired: 2 in, 2 out]
            n1030 = property on="Control Mode 8" class="Ring (strict)"("DisabledEnum"=w717) -> ()  [unwired: 2 in, 2 out]
            n1031 = property on="Camera Situation 8" class="Ring (strict)"("DisabledEnum"=w717) -> ()  [unwired: 2 in, 2 out]
          }
          frame 7..10 {
            w718 = T1."Enabled" ("Disabled")
            n1032 = property on="Disc Situation 8" class="Ring (strict)"("DisabledEnum"=w718) -> ()  [unwired: 2 in, 2 out]
            n1033 = property on="Value String 8" class="Str"("DisabledEnum"=w718) -> ()  [unwired: 2 in, 2 out]
            n1034 = property on="Time 8" class="AbsTime (strict)"("DisabledEnum"=w718) -> ()  [unwired: 2 in, 2 out]
            n1035 = property on="Date 8" class="AbsTime (strict)"("DisabledEnum"=w718) -> ()  [unwired: 2 in, 2 out]
            n1036 = property on="Projector Situation 8" class="Ring (strict)"("DisabledEnum"=w718) -> ()  [unwired: 2 in, 2 out]
            n1037 = property on="Control Mode 8" class="Ring (strict)"("DisabledEnum"=w718) -> ()  [unwired: 2 in, 2 out]
            n1038 = property on="Camera Situation 8" class="Ring (strict)"("DisabledEnum"=w718) -> ()  [unwired: 2 in, 2 out]
          }
        }
        n1039 = case shown="0, Default" "Operator 7" {
          tunnel: w161 -> [_ w723 w729 w735 w741 w747 w753 w763 w769 w778 w787]
          tunnel: w160 -> [_ _ _ _ _ _ _ w759 w768 w777 w786]
          tunnel: w162 -> [_ w725 w730 w736 w742 w748 w754 w761 w770 w779 w788]
          tunnel: ["( TRUE )" w722 w728 w734 w740 w746 w752 w758 w767 w776 w785] -> w129
          frame 0, Default {
          }
          frame 1 {
            n1040 = Concatenate Strings("( " ("string"), w725, " = " ("string"), w723, " )" ("string")) -> (w722:string)
          }
          frame 2 {
            n1041 = Concatenate Strings("( " ("string"), w730, " != " ("string"), w729, " )" ("string")) -> (w728:string)
          }
          frame 3 {
            n1042 = Concatenate Strings("( " ("string"), w736, " < " ("string"), w735, " )" ("string")) -> (w734:string)
          }
          frame 4 {
            n1043 = Concatenate Strings("( " ("string"), w742, " <= " ("string"), w741, " )" ("string")) -> (w740:string)
          }
          frame 5 {
            n1044 = Concatenate Strings("( " ("string"), w748, " > " ("string"), w747, " )" ("string")) -> (w746:string)
          }
          frame 6 {
            n1045 = Concatenate Strings("( " ("string"), w754, " >= " ("string"), w753, " )" ("string")) -> (w752:string)
          }
          frame 7 {
            n1046 = Concatenate Strings("( " ("string"), w761, " > " ("string"), w763, " AND " ("string"), w761, " < " ("string"), w759, " )" ("string")) -> (w758:string)
          }
          frame 8 {
            n1047 = Concatenate Strings("( " ("string"), w770, " >= " ("string"), w769, " AND " ("string"), w770, " < " ("string"), w768, " )" ("string")) -> (w767:string)
          }
          frame 9 {
            n1048 = Concatenate Strings("( " ("string"), w779, " > " ("string"), w778, " AND " ("string"), w779, " <= " ("string"), w777, " )" ("string")) -> (w776:string)
          }
          frame 10 {
            n1049 = Concatenate Strings("( " ("string"), w788, " >= " ("string"), w787, " AND " ("string"), w788, " <= " ("string"), w786, " )" ("string")) -> (w785:string)
          }
        }
        n1050 = case shown="0, Default" "Operator 3" {
          tunnel: w170 -> [_ w1051 w1057 w1063 w1069 w1075 w1081 w1091 w1097 w1106 w1115]
          tunnel: w169 -> [_ _ _ _ _ _ _ w1087 w1096 w1105 w1114]
          tunnel: w171 -> [_ w1053 w1058 w1064 w1070 w1076 w1082 w1089 w1098 w1107 w1116]
          tunnel: ["( TRUE )" w1050 w1056 w1062 w1068 w1074 w1080 w1086 w1095 w1104 w1113] -> w143
          frame 0, Default {
          }
          frame 1 {
            n1051 = Concatenate Strings("( " ("string"), w1053, " = " ("string"), w1051, " )" ("string")) -> (w1050:string)
          }
          frame 2 {
            n1052 = Concatenate Strings("( " ("string"), w1058, " != " ("string"), w1057, " )" ("string")) -> (w1056:string)
          }
          frame 3 {
            n1053 = Concatenate Strings("( " ("string"), w1064, " < " ("string"), w1063, " )" ("string")) -> (w1062:string)
          }
          frame 4 {
            n1054 = Concatenate Strings("( " ("string"), w1070, " <= " ("string"), w1069, " )" ("string")) -> (w1068:string)
          }
          frame 5 {
            n1055 = Concatenate Strings("( " ("string"), w1076, " > " ("string"), w1075, " )" ("string")) -> (w1074:string)
          }
          frame 6 {
            n1056 = Concatenate Strings("( " ("string"), w1082, " >= " ("string"), w1081, " )" ("string")) -> (w1080:string)
          }
          frame 7 {
            n1057 = Concatenate Strings("( " ("string"), w1089, " > " ("string"), w1091, " AND " ("string"), w1089, " < " ("string"), w1087, " )" ("string")) -> (w1086:string)
          }
          frame 8 {
            n1058 = Concatenate Strings("( " ("string"), w1098, " >= " ("string"), w1097, " AND " ("string"), w1098, " < " ("string"), w1096, " )" ("string")) -> (w1095:string)
          }
          frame 9 {
            n1059 = Concatenate Strings("( " ("string"), w1107, " > " ("string"), w1106, " AND " ("string"), w1107, " <= " ("string"), w1105, " )" ("string")) -> (w1104:string)
          }
          frame 10 {
            n1060 = Concatenate Strings("( " ("string"), w1116, " >= " ("string"), w1115, " AND " ("string"), w1116, " <= " ("string"), w1114, " )" ("string")) -> (w1113:string)
          }
        }
        n1061 = case shown="0, Default" "Operator 5" {
          tunnel: w166 -> [_ w978 w984 w990 w996 w1002 w1008 w1018 w1024 w1033 w1042]
          tunnel: w165 -> [_ _ _ _ _ _ _ w1014 w1023 w1032 w1041]
          tunnel: w167 -> [_ w980 w985 w991 w997 w1003 w1009 w1016 w1025 w1034 w1043]
          tunnel: ["( TRUE )" w977 w983 w989 w995 w1001 w1007 w1013 w1022 w1031 w1040] -> w127
          frame 0, Default {
          }
          frame 1 {
            n1062 = Concatenate Strings("( " ("string"), w980, " = " ("string"), w978, " )" ("string")) -> (w977:string)
          }
          frame 2 {
            n1063 = Concatenate Strings("( " ("string"), w985, " != " ("string"), w984, " )" ("string")) -> (w983:string)
          }
          frame 3 {
            n1064 = Concatenate Strings("( " ("string"), w991, " < " ("string"), w990, " )" ("string")) -> (w989:string)
          }
          frame 4 {
            n1065 = Concatenate Strings("( " ("string"), w997, " <= " ("string"), w996, " )" ("string")) -> (w995:string)
          }
          frame 5 {
            n1066 = Concatenate Strings("( " ("string"), w1003, " > " ("string"), w1002, " )" ("string")) -> (w1001:string)
          }
          frame 6 {
            n1067 = Concatenate Strings("( " ("string"), w1009, " >= " ("string"), w1008, " )" ("string")) -> (w1007:string)
          }
          frame 7 {
            n1068 = Concatenate Strings("( " ("string"), w1016, " > " ("string"), w1018, " AND " ("string"), w1016, " < " ("string"), w1014, " )" ("string")) -> (w1013:string)
          }
          frame 8 {
            n1069 = Concatenate Strings("( " ("string"), w1025, " >= " ("string"), w1024, " AND " ("string"), w1025, " < " ("string"), w1023, " )" ("string")) -> (w1022:string)
          }
          frame 9 {
            n1070 = Concatenate Strings("( " ("string"), w1034, " > " ("string"), w1033, " AND " ("string"), w1034, " <= " ("string"), w1032, " )" ("string")) -> (w1031:string)
          }
          frame 10 {
            n1071 = Concatenate Strings("( " ("string"), w1043, " >= " ("string"), w1042, " AND " ("string"), w1043, " <= " ("string"), w1041, " )" ("string")) -> (w1040:string)
          }
        }
        n1072 = case shown="7..10" "Operator 5" {
          frame 0..6, Default {
            w1120 = T1."Disabled and Grayed Out" ("Disabled")
            n1073 = property on="Disc Situation 6" class="Ring (strict)"("DisabledEnum"=w1120) -> ()  [unwired: 2 in, 2 out]
            n1074 = property on="Value String 6" class="Str"("DisabledEnum"=w1120) -> ()  [unwired: 2 in, 2 out]
            n1075 = property on="Time 6" class="AbsTime (strict)"("DisabledEnum"=w1120) -> ()  [unwired: 2 in, 2 out]
            n1076 = property on="Date 6" class="AbsTime (strict)"("DisabledEnum"=w1120) -> ()  [unwired: 2 in, 2 out]
            n1077 = property on="Projector Situation 6" class="Ring (strict)"("DisabledEnum"=w1120) -> ()  [unwired: 2 in, 2 out]
            n1078 = property on="Control Mode 6" class="Ring (strict)"("DisabledEnum"=w1120) -> ()  [unwired: 2 in, 2 out]
            n1079 = property on="Camera Situation 6" class="Ring (strict)"("DisabledEnum"=w1120) -> ()  [unwired: 2 in, 2 out]
          }
          frame 7..10 {
            w1121 = T1."Enabled" ("Disabled")
            n1080 = property on="Disc Situation 6" class="Ring (strict)"("DisabledEnum"=w1121) -> ()  [unwired: 2 in, 2 out]
            n1081 = property on="Value String 6" class="Str"("DisabledEnum"=w1121) -> ()  [unwired: 2 in, 2 out]
            n1082 = property on="Time 6" class="AbsTime (strict)"("DisabledEnum"=w1121) -> ()  [unwired: 2 in, 2 out]
            n1083 = property on="Date 6" class="AbsTime (strict)"("DisabledEnum"=w1121) -> ()  [unwired: 2 in, 2 out]
            n1084 = property on="Projector Situation 6" class="Ring (strict)"("DisabledEnum"=w1121) -> ()  [unwired: 2 in, 2 out]
            n1085 = property on="Control Mode 6" class="Ring (strict)"("DisabledEnum"=w1121) -> ()  [unwired: 2 in, 2 out]
            n1086 = property on="Camera Situation 6" class="Ring (strict)"("DisabledEnum"=w1121) -> ()  [unwired: 2 in, 2 out]
          }
        }
        n1087 = case shown="0, Default" "Operator 1" {
          tunnel: w182 -> [_ w1492 w1498 w1504 w1510 w1516 w1522 w1532 w1538 w1547 w1556]
          tunnel: w181 -> [_ _ _ _ _ _ _ w1528 w1537 w1546 w1555]
          tunnel: w180 -> [_ w1494 w1499 w1505 w1511 w1517 w1523 w1530 w1539 w1548 w1557]
          tunnel: ["( TRUE )" w1491 w1497 w1503 w1509 w1515 w1521 w1527 w1536 w1545 w1554] -> w145
          frame 0, Default {
          }
          frame 1 {
            n1088 = Concatenate Strings("( " ("string"), w1494, " = " ("string"), w1492, " )" ("string")) -> (w1491:string)
          }
          frame 2 {
            n1089 = Concatenate Strings("( " ("string"), w1499, " != " ("string"), w1498, " )" ("string")) -> (w1497:string)
          }
          frame 3 {
            n1090 = Concatenate Strings("( " ("string"), w1505, " < " ("string"), w1504, " )" ("string")) -> (w1503:string)
          }
          frame 4 {
            n1091 = Concatenate Strings("( " ("string"), w1511, " <= " ("string"), w1510, " )" ("string")) -> (w1509:string)
          }
          frame 5 {
            n1092 = Concatenate Strings("( " ("string"), w1517, " > " ("string"), w1516, " )" ("string")) -> (w1515:string)
          }
          frame 6 {
            n1093 = Concatenate Strings("( " ("string"), w1523, " >= " ("string"), w1522, " )" ("string")) -> (w1521:string)
          }
          frame 7 {
            n1094 = Concatenate Strings("( " ("string"), w1530, " > " ("string"), w1532, " AND " ("string"), w1530, " < " ("string"), w1528, " )" ("string")) -> (w1527:string)
          }
          frame 8 {
            n1095 = Concatenate Strings("( " ("string"), w1539, " >= " ("string"), w1538, " AND " ("string"), w1539, " < " ("string"), w1537, " )" ("string")) -> (w1536:string)
          }
          frame 9 {
            n1096 = Concatenate Strings("( " ("string"), w1548, " > " ("string"), w1547, " AND " ("string"), w1548, " <= " ("string"), w1546, " )" ("string")) -> (w1545:string)
          }
          frame 10 {
            n1097 = Concatenate Strings("( " ("string"), w1557, " >= " ("string"), w1556, " AND " ("string"), w1557, " <= " ("string"), w1555, " )" ("string")) -> (w1554:string)
          }
        }
        n1098 = case shown="7..10" "Operator 9" {
          frame 0..6, Default {
            w203 = T1."Disabled and Grayed Out" ("Disabled")
            n1099 = property on="Disc Situation 10" class="Ring (strict)"("DisabledEnum"=w203) -> ()  [unwired: 2 in, 2 out]
            n1100 = property on="Value String 10" class="Str"("DisabledEnum"=w203) -> ()  [unwired: 2 in, 2 out]
            n1101 = property on="Time 10" class="AbsTime (strict)"("DisabledEnum"=w203) -> ()  [unwired: 2 in, 2 out]
            n1102 = property on="Date 10" class="AbsTime (strict)"("DisabledEnum"=w203) -> ()  [unwired: 2 in, 2 out]
            n1103 = property on="Projector Situation 10" class="Ring (strict)"("DisabledEnum"=w203) -> ()  [unwired: 2 in, 2 out]
            n1104 = property on="Control Mode 10" class="Ring (strict)"("DisabledEnum"=w203) -> ()  [unwired: 2 in, 2 out]
            n1105 = property on="Camera Situation 10" class="Ring (strict)"("DisabledEnum"=w203) -> ()  [unwired: 2 in, 2 out]
          }
          frame 7..10 {
            w204 = T1."Enabled" ("Disabled")
            n1106 = property on="Disc Situation 10" class="Ring (strict)"("DisabledEnum"=w204) -> ()  [unwired: 2 in, 2 out]
            n1107 = property on="Value String 10" class="Str"("DisabledEnum"=w204) -> ()  [unwired: 2 in, 2 out]
            n1108 = property on="Time 10" class="AbsTime (strict)"("DisabledEnum"=w204) -> ()  [unwired: 2 in, 2 out]
            n1109 = property on="Date 10" class="AbsTime (strict)"("DisabledEnum"=w204) -> ()  [unwired: 2 in, 2 out]
            n1110 = property on="Projector Situation 10" class="Ring (strict)"("DisabledEnum"=w204) -> ()  [unwired: 2 in, 2 out]
            n1111 = property on="Control Mode 10" class="Ring (strict)"("DisabledEnum"=w204) -> ()  [unwired: 2 in, 2 out]
            n1112 = property on="Camera Situation 10" class="Ring (strict)"("DisabledEnum"=w204) -> ()  [unwired: 2 in, 2 out]
          }
        }
        n1113 = case shown="0, Default" "Operator 9" {
          tunnel: w151 -> [_ w209 w215 w221 w227 w233 w239 w249 w255 w264 w273]
          tunnel: w150 -> [_ _ _ _ _ _ _ w245 w254 w263 w272]
          tunnel: w152 -> [_ w211 w216 w222 w228 w234 w240 w247 w256 w265 w274]
          tunnel: ["( TRUE )" w208 w214 w220 w226 w232 w238 w244 w253 w262 w271] -> w124
          frame 0, Default {
          }
          frame 1 {
            n1114 = Concatenate Strings("( " ("string"), w211, " = " ("string"), w209, " )" ("string")) -> (w208:string)
          }
          frame 2 {
            n1115 = Concatenate Strings("( " ("string"), w216, " != " ("string"), w215, " )" ("string")) -> (w214:string)
          }
          frame 3 {
            n1116 = Concatenate Strings("( " ("string"), w222, " < " ("string"), w221, " )" ("string")) -> (w220:string)
          }
          frame 4 {
            n1117 = Concatenate Strings("( " ("string"), w228, " <= " ("string"), w227, " )" ("string")) -> (w226:string)
          }
          frame 5 {
            n1118 = Concatenate Strings("( " ("string"), w234, " > " ("string"), w233, " )" ("string")) -> (w232:string)
          }
          frame 6 {
            n1119 = Concatenate Strings("( " ("string"), w240, " >= " ("string"), w239, " )" ("string")) -> (w238:string)
          }
          frame 7 {
            n1120 = Concatenate Strings("( " ("string"), w247, " > " ("string"), w249, " AND " ("string"), w247, " < " ("string"), w245, " )" ("string")) -> (w244:string)
          }
          frame 8 {
            n1121 = Concatenate Strings("( " ("string"), w256, " >= " ("string"), w255, " AND " ("string"), w256, " < " ("string"), w254, " )" ("string")) -> (w253:string)
          }
          frame 9 {
            n1122 = Concatenate Strings("( " ("string"), w265, " > " ("string"), w264, " AND " ("string"), w265, " <= " ("string"), w263, " )" ("string")) -> (w262:string)
          }
          frame 10 {
            n1123 = Concatenate Strings("( " ("string"), w274, " >= " ("string"), w273, " AND " ("string"), w274, " <= " ("string"), w272, " )" ("string")) -> (w271:string)
          }
        }
        n1124 = case shown="7..10" "Operator 11" {
          frame 0..6, Default {
            w351 = T1."Disabled and Grayed Out" ("Disabled")
            n1125 = property on="Disc Situation 12" class="Ring (strict)"("DisabledEnum"=w351) -> ()  [unwired: 2 in, 2 out]
            n1126 = property on="Value String 12" class="Str"("DisabledEnum"=w351) -> ()  [unwired: 2 in, 2 out]
            n1127 = property on="Time 12" class="AbsTime (strict)"("DisabledEnum"=w351) -> ()  [unwired: 2 in, 2 out]
            n1128 = property on="Date 12" class="AbsTime (strict)"("DisabledEnum"=w351) -> ()  [unwired: 2 in, 2 out]
            n1129 = property on="Projector Situation 12" class="Ring (strict)"("DisabledEnum"=w351) -> ()  [unwired: 2 in, 2 out]
            n1130 = property on="Control Mode 12" class="Ring (strict)"("DisabledEnum"=w351) -> ()  [unwired: 2 in, 2 out]
            n1131 = property on="Camera Situation 12" class="Ring (strict)"("DisabledEnum"=w351) -> ()  [unwired: 2 in, 2 out]
          }
          frame 7..10 {
            w352 = T1."Enabled" ("Disabled")
            n1132 = property on="Disc Situation 12" class="Ring (strict)"("DisabledEnum"=w352) -> ()  [unwired: 2 in, 2 out]
            n1133 = property on="Value String 12" class="Str"("DisabledEnum"=w352) -> ()  [unwired: 2 in, 2 out]
            n1134 = property on="Time 12" class="AbsTime (strict)"("DisabledEnum"=w352) -> ()  [unwired: 2 in, 2 out]
            n1135 = property on="Date 12" class="AbsTime (strict)"("DisabledEnum"=w352) -> ()  [unwired: 2 in, 2 out]
            n1136 = property on="Projector Situation 12" class="Ring (strict)"("DisabledEnum"=w352) -> ()  [unwired: 2 in, 2 out]
            n1137 = property on="Control Mode 12" class="Ring (strict)"("DisabledEnum"=w352) -> ()  [unwired: 2 in, 2 out]
            n1138 = property on="Camera Situation 12" class="Ring (strict)"("DisabledEnum"=w352) -> ()  [unwired: 2 in, 2 out]
          }
        }
        n1139 = case shown="0, Default" "Operator 11" {
          tunnel: w155 -> [_ w282 w288 w294 w300 w306 w312 w322 w328 w337 w346]
          tunnel: w154 -> [_ _ _ _ _ _ _ w318 w327 w336 w345]
          tunnel: w156 -> [_ w284 w289 w295 w301 w307 w313 w320 w329 w338 w347]
          tunnel: ["( TRUE )" w281 w287 w293 w299 w305 w311 w317 w326 w335 w344] -> w119
          frame 0, Default {
          }
          frame 1 {
            n1140 = Concatenate Strings("( " ("string"), w284, " = " ("string"), w282, " )" ("string")) -> (w281:string)
          }
          frame 2 {
            n1141 = Concatenate Strings("( " ("string"), w289, " != " ("string"), w288, " )" ("string")) -> (w287:string)
          }
          frame 3 {
            n1142 = Concatenate Strings("( " ("string"), w295, " < " ("string"), w294, " )" ("string")) -> (w293:string)
          }
          frame 4 {
            n1143 = Concatenate Strings("( " ("string"), w301, " <= " ("string"), w300, " )" ("string")) -> (w299:string)
          }
          frame 5 {
            n1144 = Concatenate Strings("( " ("string"), w307, " > " ("string"), w306, " )" ("string")) -> (w305:string)
          }
          frame 6 {
            n1145 = Concatenate Strings("( " ("string"), w313, " >= " ("string"), w312, " )" ("string")) -> (w311:string)
          }
          frame 7 {
            n1146 = Concatenate Strings("( " ("string"), w320, " > " ("string"), w322, " AND " ("string"), w320, " < " ("string"), w318, " )" ("string")) -> (w317:string)
          }
          frame 8 {
            n1147 = Concatenate Strings("( " ("string"), w329, " >= " ("string"), w328, " AND " ("string"), w329, " < " ("string"), w327, " )" ("string")) -> (w326:string)
          }
          frame 9 {
            n1148 = Concatenate Strings("( " ("string"), w338, " > " ("string"), w337, " AND " ("string"), w338, " <= " ("string"), w336, " )" ("string")) -> (w335:string)
          }
          frame 10 {
            n1149 = Concatenate Strings("( " ("string"), w347, " >= " ("string"), w346, " AND " ("string"), w347, " <= " ("string"), w345, " )" ("string")) -> (w344:string)
          }
        }
        n1150 = case shown="0, Default" "Operator 13" {
          tunnel: [" AND " " OR "] -> w148
          frame 0, Default {
          }
          frame 1 {
          }
        }
        n1151 = property on="sub 1" class="Bool"() -> ("Visible"=w146:bool)  [unwired: 2 in, 2 out]
        n1152 = case shown="0, Default" "Operator 15" {
          tunnel: [" AND " " OR "] -> w135
          frame 0, Default {
          }
          frame 1 {
          }
        }
        n1153 = case shown="0, Default" "Operator 14" {
          tunnel: [" AND " " OR "] -> w141
          frame 0, Default {
          }
          frame 1 {
          }
        }
        n1154 = property on="sub 3" class="Bool"() -> ("Visible"=w134:bool)  [unwired: 2 in, 2 out]
        n1155 = property on="sub 2" class="Bool"() -> ("Visible"=w139:bool)  [unwired: 2 in, 2 out]
        n1156 = case shown="0, Default" "Operator 16" {
          tunnel: [" AND " " OR "] -> w130
          frame 0, Default {
          }
          frame 1 {
          }
        }
        n1157 = property on="sub 4" class="Bool"() -> ("Visible"=w132:bool)  [unwired: 2 in, 2 out]
        n1158 = property on="sub 5" class="Bool"() -> ("Visible"=w122:bool)  [unwired: 2 in, 2 out]
        n1159 = case shown="0, Default" "Operator 17" {
          tunnel: [" AND " " OR "] -> w121
          frame 0, Default {
          }
          frame 1 {
          }
        }
        n1160 = Select(t=w148, s=w146, f=" AND ") -> (s? t:f=w144:string)
        n1161 = Select(t=w135, s=w134, f=" AND ") -> (s? t:f=w126:string)
        n1162 = Select(t=w141, s=w139, f=" AND ") -> (s? t:f=w138:string)
        n1163 = Select(t=w130, s=w132, f=" AND ") -> (s? t:f=w125:string)
        n1164 = Select(t=w121, s=w122, f=" AND ") -> (s? t:f=w120:string)
        n1165 = Concatenate Strings("WHERE " ("string"), w145, w144, w143, w138, w127, w126, w129, w125, w124, w120, w119, " ORDER BY id DESC" ("string")) -> (→"Query String":string)
      }
    }
  }
  n1166 = property on="sub 1" class="Bool"("Visible"=FALSE) -> ()  [unwired: 2 in, 2 out]
  n1167 = property on="add 5" class="Bool"("Visible"=FALSE) -> ()  [unwired: 2 in, 2 out]
  n1168 = property on="add 2" class="Bool"("Visible"=FALSE) -> ()  [unwired: 2 in, 2 out]
  n1169 = property on="add 4" class="Bool"("Visible"=FALSE) -> ()  [unwired: 2 in, 2 out]
  n1170 = property on="add 3" class="Bool"("Visible"=FALSE) -> ()  [unwired: 2 in, 2 out]
  n1171 = property on="sub 5" class="Bool"("Visible"=FALSE) -> ()  [unwired: 2 in, 2 out]
  n1172 = property on="sub 3" class="Bool"("Visible"=FALSE) -> ()  [unwired: 2 in, 2 out]
  n1173 = property on="sub 4" class="Bool"("Visible"=FALSE) -> ()  [unwired: 2 in, 2 out]
  n1174 = property on="sub 2" class="Bool"("Visible"=FALSE) -> ()  [unwired: 2 in, 2 out]
  n1175 = property on="add 1" class="Bool"("Visible"=TRUE) -> ()  [unwired: 2 in, 2 out]
  n1176 = shared-variable ".\\database.lvlib\\search"(FALSE ("search")) -> ()  [unwired: 1 in, 1 out]
  "String 1" <- "Value 1" ("String 1")
  "String 2" <- "Value 2" ("String 2")
  "String 3" <- "Operation" ("String 1")
  "String 4" <- "Parameter" ("String 4")
  "Value String 1" <- "Value" ("Value String 1")
  "Value String 2" <- "Value" ("Value String 2")
  "Value String 3" <- "Value" ("Value String 3")
  "Value String 4" <- "Value" ("Value String 4")
  "Value String 5" <- "Value" ("Value String 5")
  "Value String 6" <- "Value" ("Value String 6")
  "Value String 7" <- "Value" ("Value String 7")
  "Value String 8" <- "Value" ("Value String 8")
  "Value String 9" <- "Value" ("Value String 9")
  "Value String 10" <- "Value" ("Value String 10")
  "Value String 11" <- "Value" ("Value String 11")
  "Value String 12" <- "Value" ("Value String 12")
  "Name" <- "Search in Database" ("Name")
